vi "NMLWSD_Stability_8Units Rev B.vi"() -> ()   [LabVIEW 2017]
uses:
  C:/Program Files (x86)/Newport/Newport USB Driver/Bin/UsbDllWrap.dll
  Program Files (x86)/Newport/Newport USB Driver/Bin/UsbDllWrap.dll
  <vilib>/Analysis/baseanly.llb/Mean (DBL).vi
  <vilib>/Utility/file.llb/Read Delimited Spreadsheet (string).vi
  <vilib>/Utility/file.llb/Write Delimited Spreadsheet (string).vi
  <vilib>/Utility/file.llb/Read Delimited Spreadsheet (DBL).vi
  <vilib>/Analysis/NI_AALBase.lvlib
panel:
  out "Start Power":dbl=0.005 format="%.3p"
  out "Max Deviation":dbl format="%.2g %%"
  out "Min Power":dbl format="%.3p"
  out "Max Power":dbl format="%.3p"
  out "First Point":dbl format="%<%I:%M %p %m/%d/%y>T"
  out "Data Error":bool
  out "Timeout":bool
  out "Busy":bool
  out "Error":bool
  out "Msg":string="\n\r" caption="Status"
  in  "Stop":bool
  in  "Menu":T1(tab)
  in  "Comments":string[](array[string])=["", "", "", "", "", "", "", ""]
  in  "Start Test":bool
  out "Time":T2(graph) caption="Datar"
  in  "Display Parameter":u16(ring) items=["FW Version:", "On time (s):", "#shutter cycles:", "#power cycles:", "Temperature (°C):", "Temp set pt (°C):", "Tmax diode: (°C):", "Tmin laser: (°C):", "Tamb max: (°C):", "Hamb max: (RH):", "Current Tamb: (°C):", "Current Hamb: (RH):", "I_TEC (A):", "Laser Current (mA):", "IBias Initial(mA):", "MD Current (uA):", "APC_Set (V):", "Mod_Set (V):", "Vtune (V):", "LHM (V):", "Mode:", "WL:", "LHM Cal Gain:", "LHM Cal Offset:", "Power (W):", "Chamber Temperature (°C):", "V Logic (V):", "I Logic (A):", "V Laser (V):", "I Laser (A):", "V TEC (V):", "I TEC (A):", "V 24V (V):", "I 24V (A):", "Power_closed (W):"]
  out "Time 2":T2(graph) caption="Datar"
  in  "Read":bool
  out "Curs":dbl format="%<%I:%M %p %m/%d/%y>T"
  out "Pos":dbl format="%_3g"
  out "Results":bool
  in  "Display UUT #":i32(ring) items=["194910NPI-8NML", "194918NPI-8NML", "194805NPI-7NML", "194806NPI-7NML", "194911NPI-8NML", "194504NPI-8NML", "175003NPI-7NML", "194804NPI-7NML"]
  in  "New File":bool
  in  "Serial Numbers":string[](array[string])=["", "", "", "", "", "", "", ""]
  in  "DUT Count":i32(ring)=1 items=["1"=1, "2"=2, "3"=3, "4"=4, "5"=5, "6"=6, "7"=7, "8"=8]
  in  "Verify WavL":bool
  out "Re-conf Lambda":bool caption="Restart Test"
  out "Ready":bool caption="Restart Test"
  out "cDAQ2":string
  in  "Parameter File":path=path "C:/Test/WSNM Stability/Firmware_System/FW-Sys.csv"
  in  "Select Unit":i32(ring) items=["Unit 1", "Unit 2", "Unit 3", "Unit 4"]
  in  "Save Data":bool
  in  "850nm Folder":path=path "C:/Test/WSNM Stability/Data/850nm"
  in  "780nm Folder":path=path "C:/Test/WSNM Stability/Data/780nm"
  in  "635nm Folder":path=path "C:/Test/WSNM Stability/Data/635nm"
  out "Tpass Shtr Close":bool
  out "Shtr Close":bool
  out "Shtr Open":bool
  in  "Prep, min":dbl=30.0 min=0.0 format="%.2g"
  out "Com Open":bool[](array[boolean])=[FALSE, FALSE, FALSE, FALSE, FALSE, FALSE, FALSE, FALSE, FALSE, FALSE, TRUE, TRUE, TRUE, TRUE, TRUE, TRUE, TRUE, TRUE, TRUE, TRUE, TRUE, TRUE, TRUE, TRUE, TRUE, TRUE, TRUE, TRUE, TRUE, TRUE]
  out "Points":i32[](array[numeric])
  out "Devices":string[](array[string])
  out "COMs":refnum<visa-resource-name>[](array[refnum])
  out "Serial":string[](array[string])=["1"]
  out "System":string[][](table)
  in  "Open Ports":bool
  in  "Close Ports":bool
  in  "Reset PMs":bool
  out "cDAQ1":string
  in  "Open  Shutters":bool
  in  "Measure":bool
  in  "Power":bool
  in  "Clear Data":bool
  in  "Project Folder":path=path "C:/Test/WSNM Stability/Data"
  in  "Log File":path=path "C:/Test/WSNM Stability/Log.txt"
  in  "Settings File":path=path "C:/Test/WSNM Stability/Settings.txt"
  out "TimeS":string caption="Time"
  out "DateS":string caption="Date"
  in  "Stability Time, min":dbl=120.0 min=0.0 format="%.2f"
  in  "Warm-up, min":dbl=25.0 min=0.0 format="%.2g"
  in  "Interval, Seconds":dbl=10.0 min=0.0 format="%.2f"
  in  "Reset PSs":bool
  in  "Close  Shutters":bool
  in  "Shtr Ctrl Open, min":dbl=0.1 min=0.0 max=60.0 format="%.3f"
  in  "Shtr Ctrl Close, Seconds":dbl=6.0 max=60.0 format="%.3f"
  out "Tpass Shtr Open":bool
  in  "COM":refnum<visa-resource-name>="COM1"
  in  "PM USB Address":i32=1
  out "Lambda, nm":i32[](array[numeric])
  out "NML_WL":u16
  out "FW":u16
  in  "WL: NML Only":i32(ring)=1 items=["Red Only", "IR"]
  in  "FW inTest":u16(ring)=1 items=["WSD Board", "NML Board"]
  out "Enable":bool[](array[boolean])
  out "Module Error":bool[](array[boolean])
  out "PM_Range":i32 min=0 max=7 step=1
  out "System Data":dbl[](array[numeric]) format="%#_5p"
  out "MCU Data":dbl[](array[numeric]) format="%#_5p"
  out "Sys Prm":string[](array[string])=["Power (W):", "Chamber Temperature (°C):", "V Logic (V):", "I Logic (A):", "V Laser (V):", "I Laser (A):", "V TEC (V):", "I TEC (A):", "V 24V (V):", "I 24V (A):", "Power_closed (W):"]
  out "All Results":dbl[][][](array[numeric]) format="%8_4g"
  out "Order":string[](array[string])
  out "FW-SYS Info":string[][](table)
  out "FW ID":string[](array[string])
  out "FW Prm":string[](array[string])
  out "Pause":bool
  in  "Supply-PM Count":i32=4 min=1 max=4 step=1
  out "InitCriteria":bool
  out "PS RST":bool=TRUE
  out "Start Time":timestamp
  out "SysFileDelete":i32=30
  out "New Test":bool
  out "Soak Complete":bool=TRUE
  out "read buffer":string
  out "System Messages":string
  out "work buffer":string
  out "error":errorcluster
  out "DUT Count Old":i32=30
  out "Data Time":timestamp
  out "Old Cursor":dbl format="%<%I:%M %p %m/%d>T"
  out "Parameter Displayed":u16
  in  "Ret Prm IR":string[](array[string])=["FW Version:", "On time (s):", "#shutter cycles:", "#power cycles:", "Temperature (°C):", "Temp set pt (°C):", "Tmax diode: (°C):", "Tmin laser: (°C):", "Tamb max: (°C):", "Hamb max: (RH):", "Current Tamb: (°C):", "Current Hamb: (RH):", "I_TEC (A):", "Laser Current (mA):", "IBias Initial(mA):", "MD Current (uA):", "APC_Set (V):", "Mod_Set (V):", "Vtune (V):", "LHM (V):"]
  in  "Ret Prm Red":string[](array[string])=["Temperature (°C):", "Temp set pt (°C):", "Highest temp seen: (°C):", "Lowest temp seen: (°C):", "TEC current (A):", "Laser Current (mA):", "MD Current (uA):", "Power_Set (V):", "Modulation_Set (V):"]
  out "Powertime":dbl[](array[numeric]) format="%#_5p"
  out "Bytes Rcvd":i32=1000
  out "DUT Selected":i32
  out "Display UUT # Old":i32=30
  out "Meas N":i32
  out "Update Graph":bool
  out "Save":bool
  out "Collect":bool
  out "Shtr Ref Time":timestamp
  out "Shtr Ref0":timestamp
  out "reference Out":refnum<k24>
  out "ShtrCtrl Open Old":dbl=3.0 min=0.0 max=60.0 format="%.1f"
  out "ShtrCtrl Close Old":dbl=3.0 max=60.0 format="%.1f"
  out "MCUTrue":bool[][](array[boolean])
  out "SysTrue":bool[][](array[boolean])
  out "MCUCheck":string[][](array[string])
  out "SysCheck":string[][](array[string])
  out "MCUTrue2":bool[][](array[boolean])
  out "MCUReview2":bool[][](array[boolean])
  out "SysTrue2":bool[][](array[boolean])
  out "SysReview2":bool[][](array[boolean])
  out "FW Criteria":string[][](array[string])
  out "Sys Criteria":string[][](array[string])
  out "Ret Prm":string[](array[string])=["FW Version:", "On time (s):", "#shutter cycles:", "#power cycles:", "Temperature (°C):", "Temp set pt (°C):", "Tmax diode: (°C):", "Tmin laser: (°C):", "Tamb max: (°C):", "Hamb max: (RH):", "Current Tamb: (°C):", "Current Hamb: (RH):", "I_TEC (A):", "Laser Current (mA):", "IBias Initial(mA):", "MD Current (uA):", "APC_Set (V):", "Mod_Set (V):", "Vtune (V):", "LHM (V):"]
  out "MCUReview":bool[][](array[boolean])=[[TRUE], [TRUE], [TRUE], [TRUE], [TRUE], [TRUE], [TRUE], [FALSE], [TRUE], [FALSE], [FALSE], [FALSE], [FALSE], [TRUE], [TRUE], [TRUE], [TRUE], [TRUE], [TRUE], [FALSE], [FALSE], [FALSE], [TRUE], [TRUE], [TRUE], [FALSE], [FALSE], [TRUE], [TRUE], [TRUE], [TRUE], [TRUE], [TRUE], [TRUE], [FALSE], [TRUE], [FALSE], [FALSE]]
  out "SysReview":bool[][](array[boolean])
  # "NML/WSD Stability Test"
  # "Newport ISB"
  # "Configure"
  # "Test"
  # "Data"
  # "Folders"
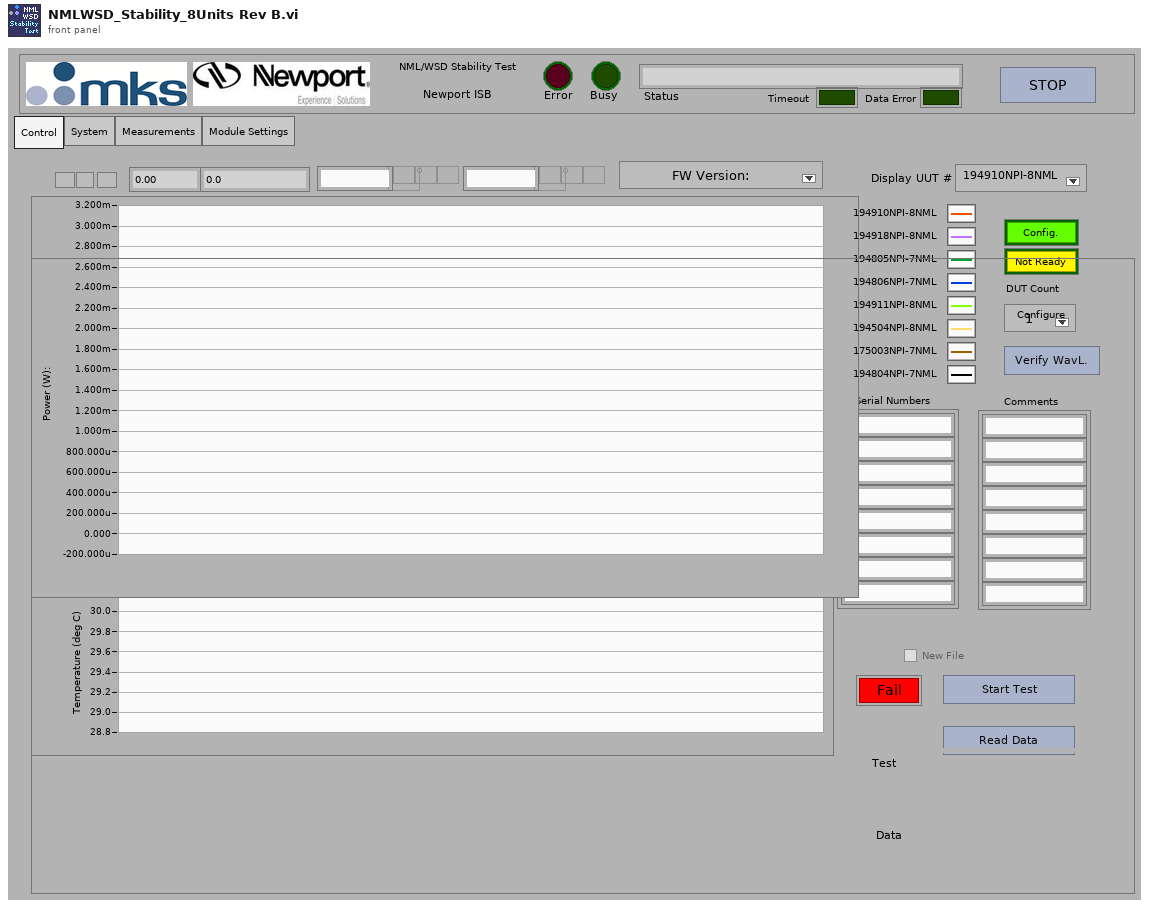
[diagram p1: front panel]
types:
  T1 = enum32{"Control", "System", "Measurements", "Module Settings"}
  T2 = cluster{"TimeStamps":timestamp[], " D Min":dbl[]}[]
  T3 = enum8{"Enabled", "Disabled", "Disabled and Grayed Out"}
  T4 = typedef "LVRangeTypeDef.ctl" = cluster{"Minimum":dbl, "Maximum":dbl, "Increment":dbl, "Minor Increment":dbl, "Start":dbl}
  T5 = typedef "LVRectTypeDef.ctl" = cluster{"Left":i16, "Top":i16, "Right":i16, "Bottom":i16}
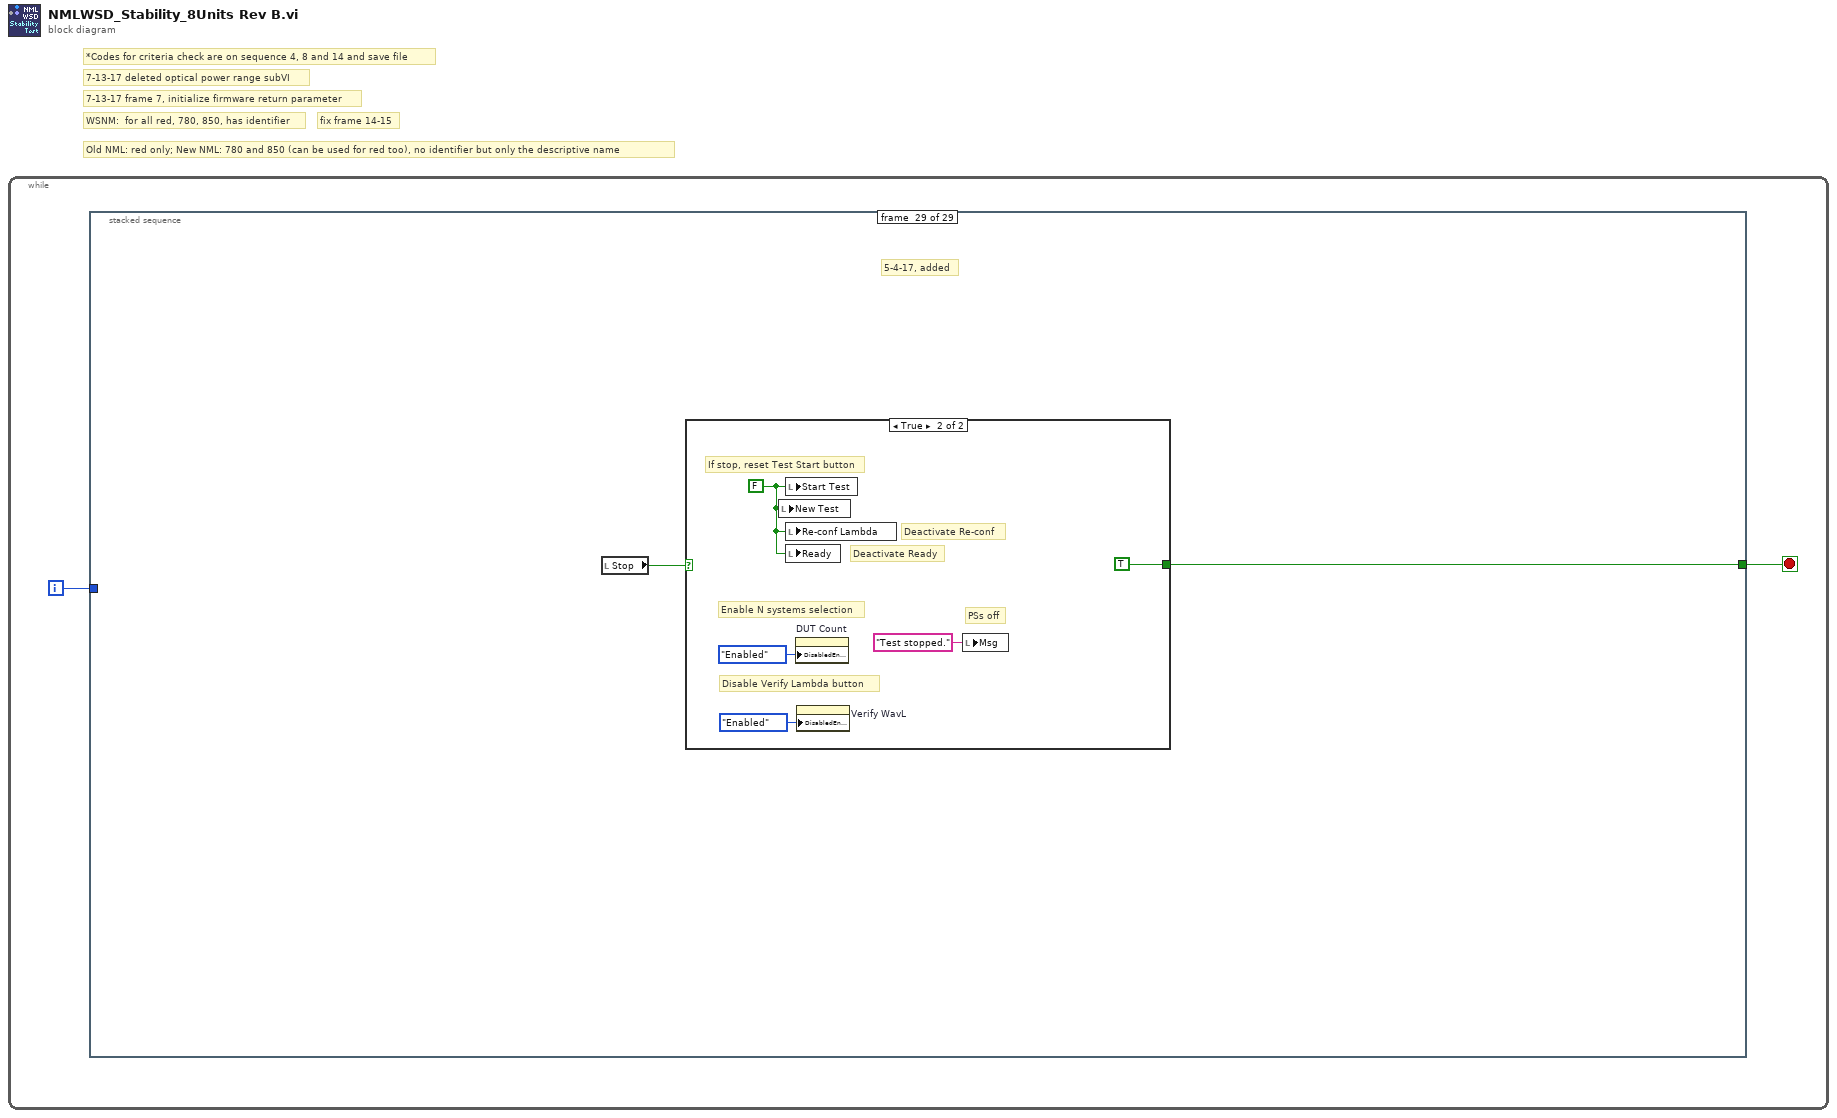
[diagram p0: block diagram]
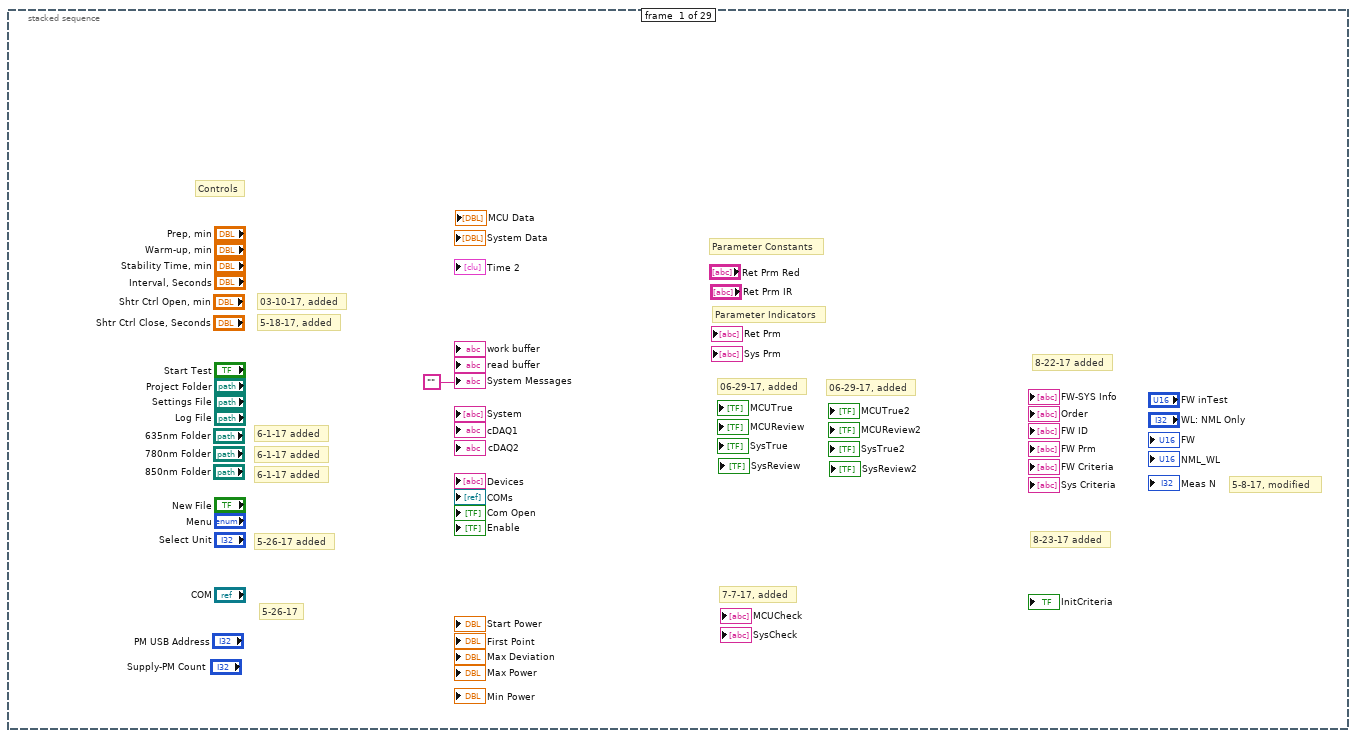
[diagram p2: hidden frame]
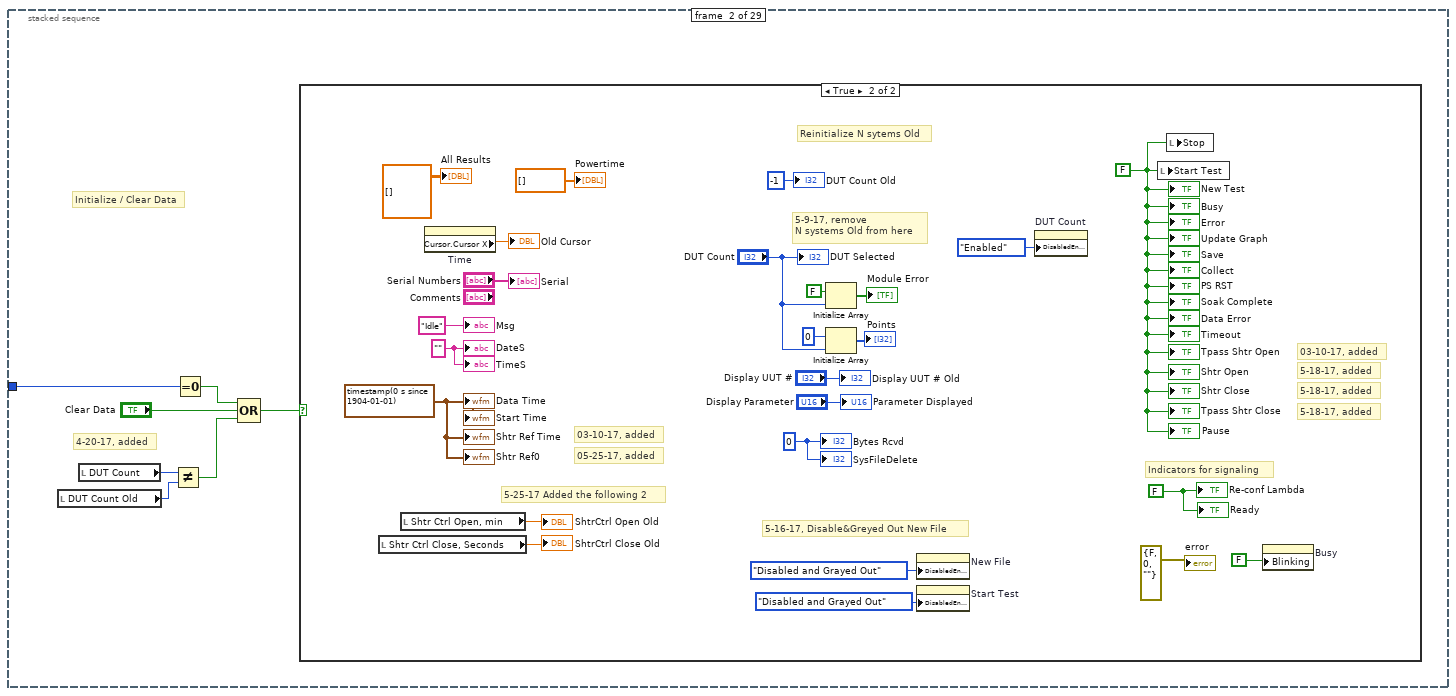
[diagram p3: hidden frame]
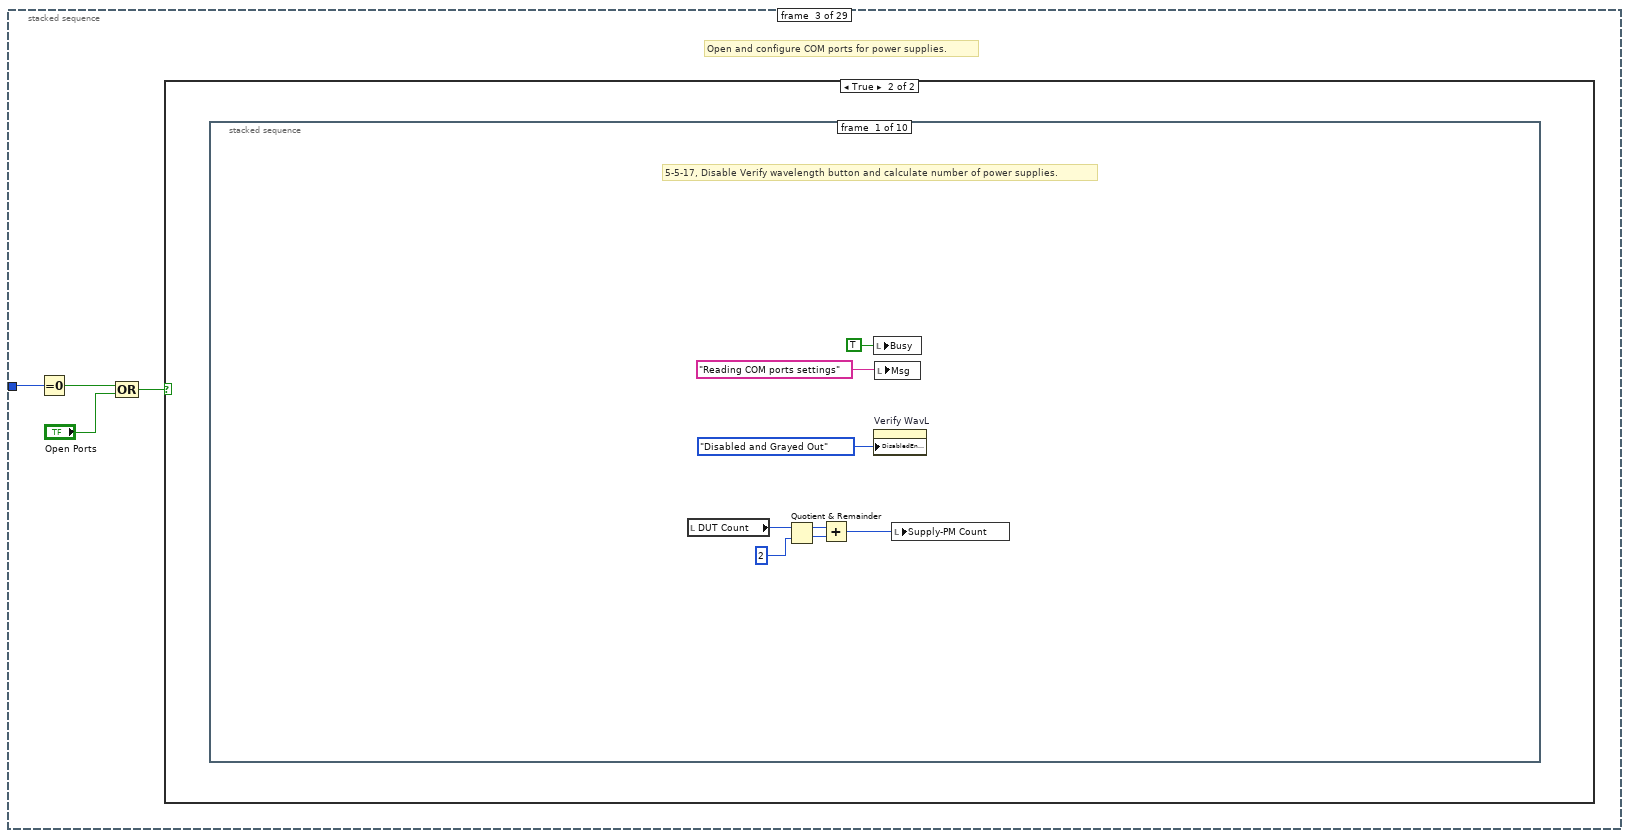
[diagram p5: hidden frame]
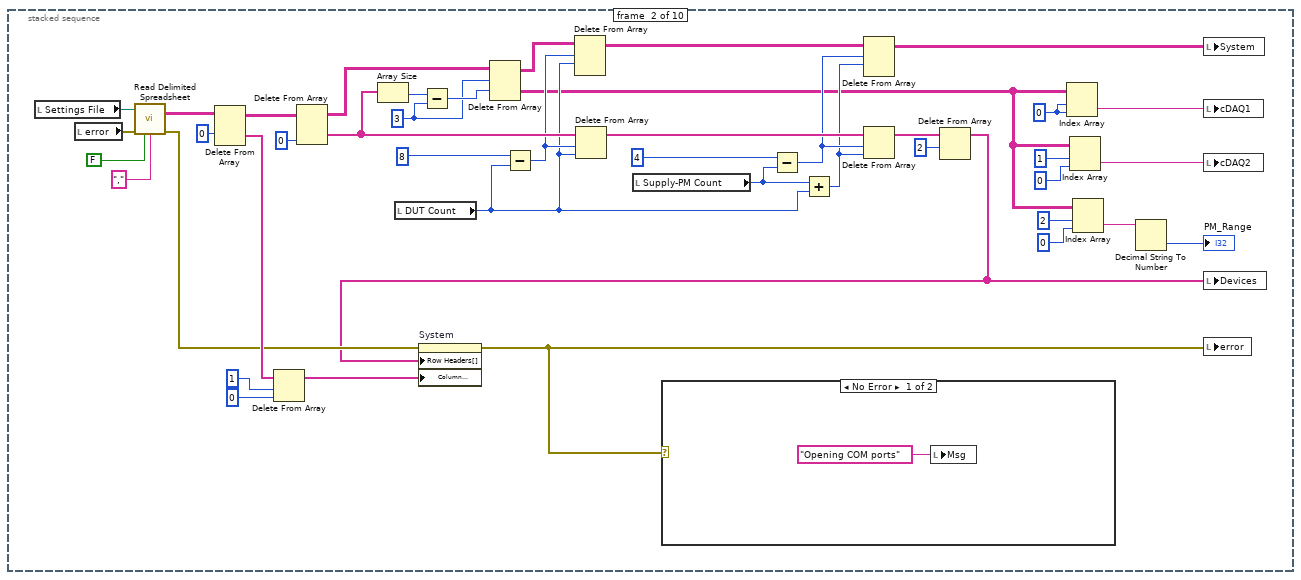
[diagram p7: hidden frame]
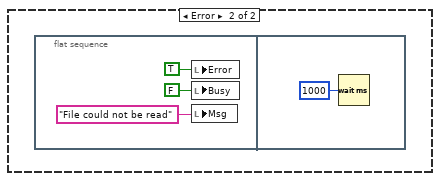
[diagram p8: hidden frame]
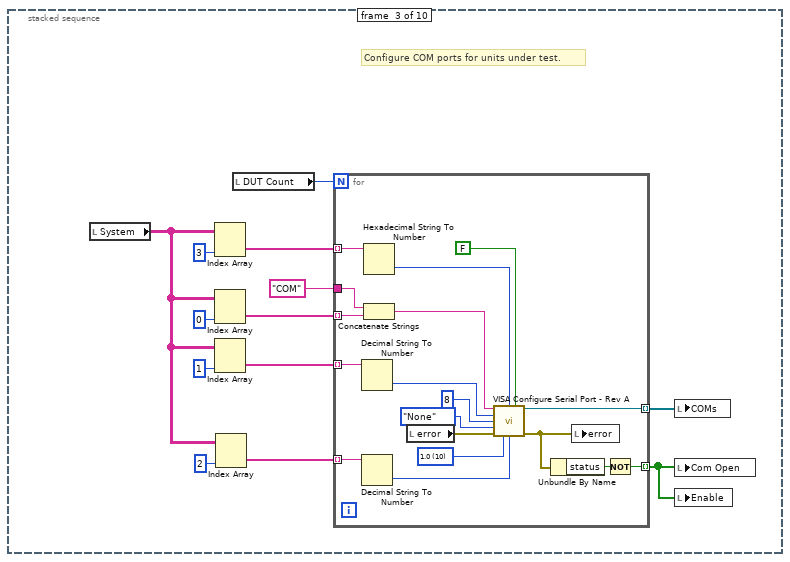
[diagram p9: hidden frame]
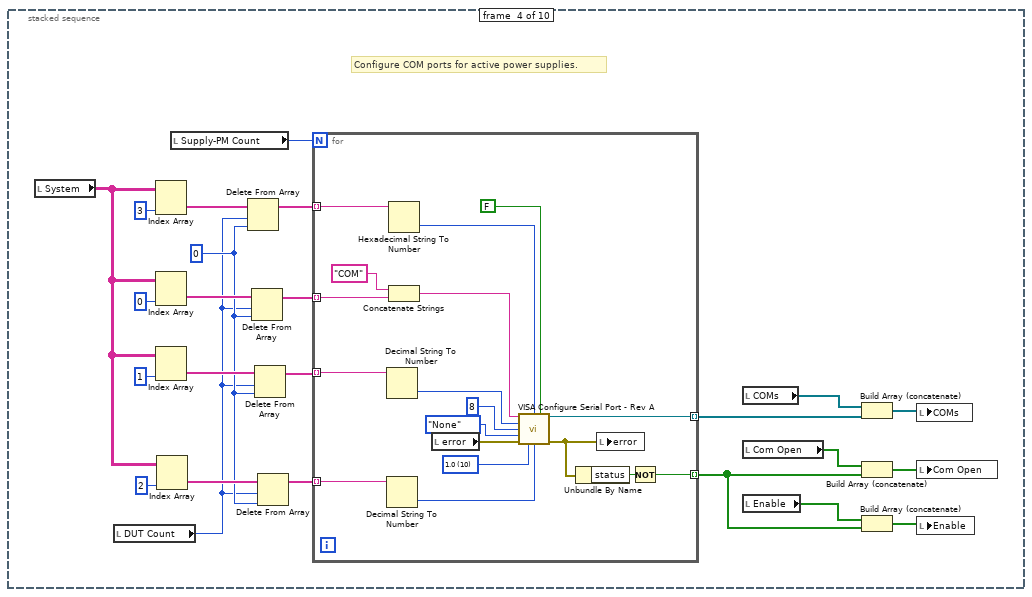
[diagram p10: hidden frame]
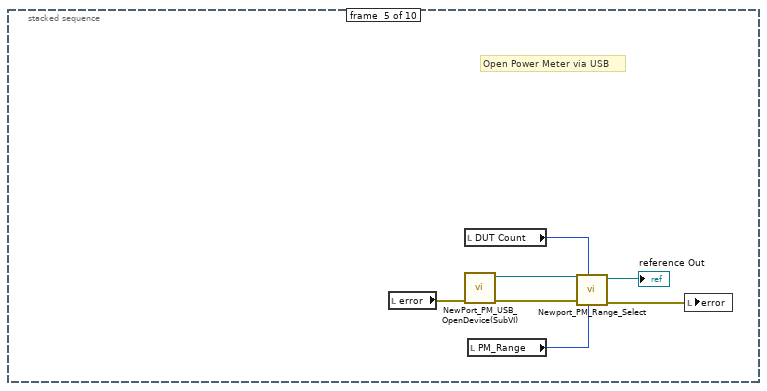
[diagram p11: hidden frame]
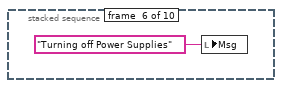
[diagram p12: hidden frame]
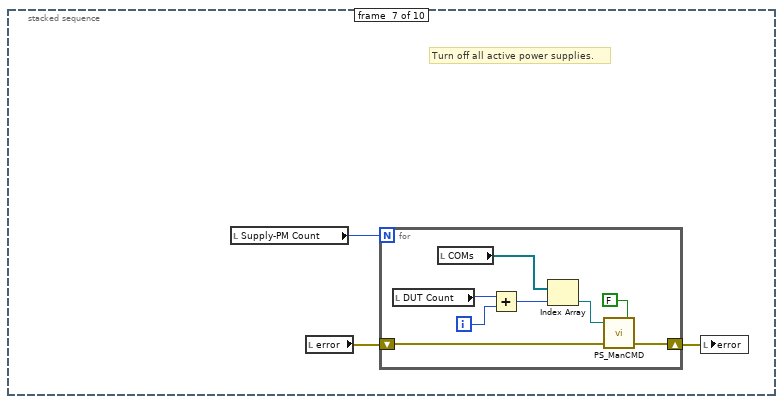
[diagram p13: hidden frame]
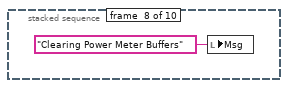
[diagram p14: hidden frame]
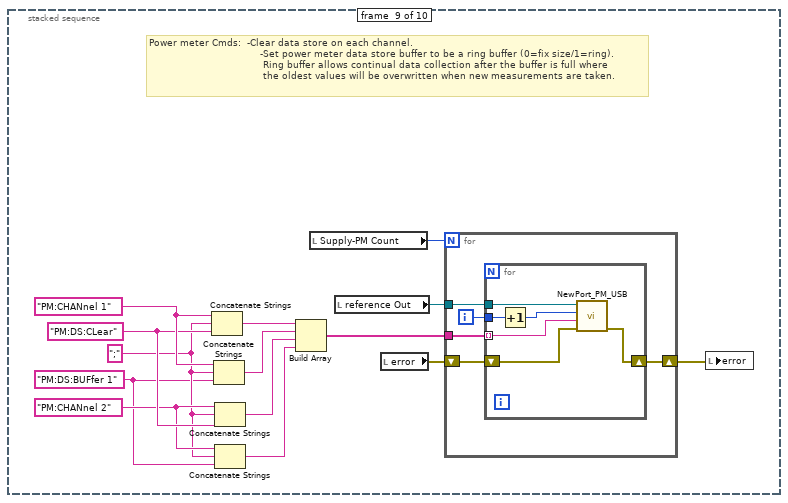
[diagram p15: hidden frame]
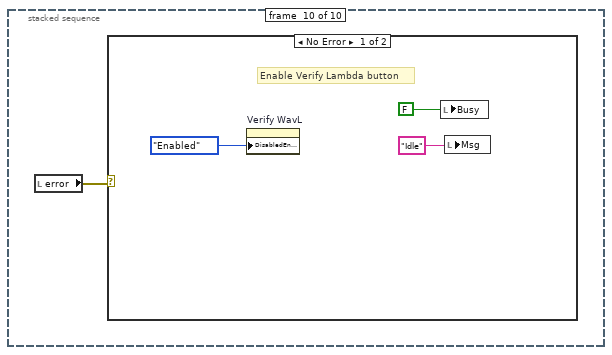
[diagram p16: hidden frame]
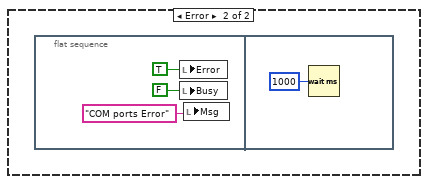
[diagram p17: hidden frame]
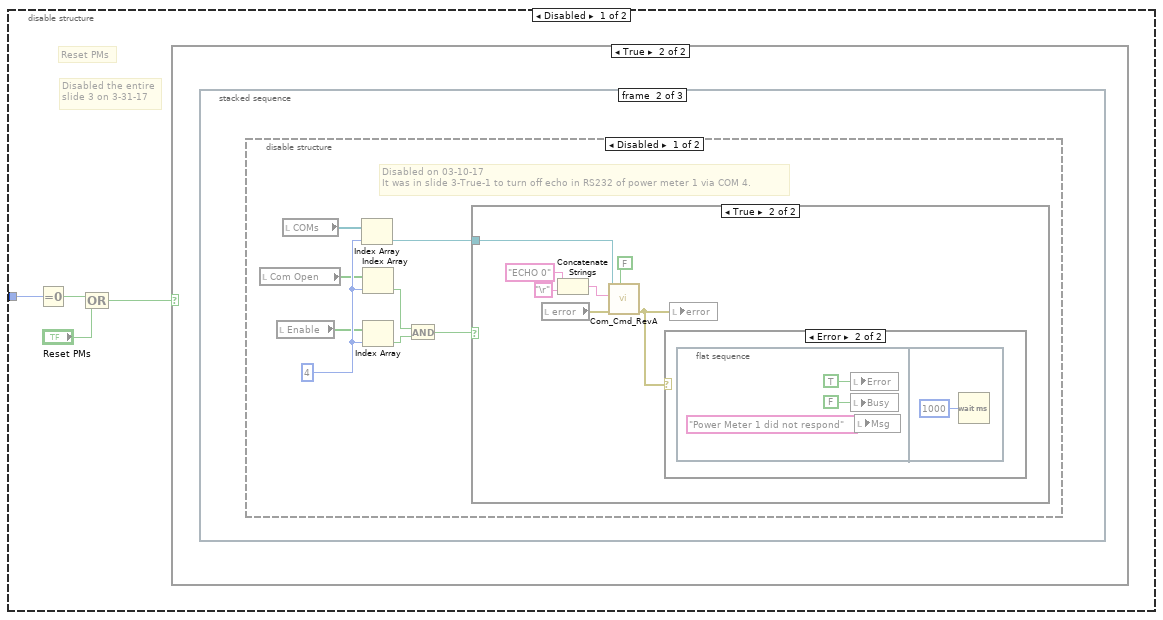
[diagram p19: hidden frame]
diagram:
  # "Old NML: red only; New NML: 780 and 850 (can be used for red too), no identifier but only the descriptive name"
  # "WSNM:  for all red, 780, 850, has identifier"
  # "*Codes for criteria check are on sequence 4, 8 and 14 and save file"
  # "fix frame 14-15"
  # "7-13-17 frame 7, initialize firmware return parameter"
  # "7-13-17 deleted optical power range subVI"
  n1 = while {
    i -> [w2]
    stop <- w1 stop-if-true
    n2 = stacked-sequence {
      tunnel: w2 -> [_ w10 w39 w222 w281 _ w331 _ _ w708 _ _ _ _ _ _ _ _ _ _ _ _ w1938 _ _ _ _ _ _]
      tunnel: [_ _ _ _ _ _ _ _ _ _ _ _ _ _ _ _ _ _ _ _ _ _ _ _ _ _ _ _ w2134] -> w1
      frame #0 {
        # "5-8-17, modified"
        # "8-23-17 added"
        # "8-22-17 added"
        # "06-29-17, added"
        # "7-7-17, added"
        # "06-29-17, added"
        # "6-1-17 added"
        # "6-1-17 added"
        # "6-1-17 added"
        # "5-26-17 added"
        # "5-26-17"
        # "Parameter Indicators"
        # "Parameter Constants"
        # "5-18-17, added"
        # "03-10-17, added"
        # "Controls"
        "System Messages" <- ""
      }
      frame #1 {
        # "4-20-17, added"
        # "Initialize / Clear Data"
        n3 = local read "DUT Count Old"() -> (w5:i32)
        n4 = local read "DUT Count"() -> (w6:i32)
        n5 = Not Equal?(x=w6, y=w5) -> (x != y?=w4:bool)
        n6 = Equal To 0?(x=w10) -> (x = 0?=w9:bool)
        n7 = Compound Arithmetic op=OR(w9, "Clear Data", w4) -> (w7:bool)
        n8 = case shown="True" w7 {
          frame False {
          }
          frame True {
            w12 = FALSE ("Restart Test")
            w22 = "" ("Result")
            w17 = 0 ("Bytes Rcvd")
            w11 = FALSE ("Auto")
            w27 = timestamp(0 s since 1904-01-01) ("Data Time")
            # "Indicators for signaling"
            # "5-25-17 Added the following 2"
            # "5-18-17, added"
            # "5-18-17, added"
            # "5-18-17, added"
            # "5-16-17, Disable&Greyed Out New File"
            # "Reinitialize N sytems Old"
            # "5-9-17, remove \nN systems Old from here"
            # "03-10-17, added"
            # "05-25-17, added"
            # "03-10-17, added"
            n9 = local read "Shtr Ctrl Close, Seconds"() -> (→"ShtrCtrl Close Old":dbl)
            n10 = local read "Shtr Ctrl Open, min"() -> (→"ShtrCtrl Open Old":dbl)
            n11 = property on="Time" class="XYGraph (strict)"() -> ("Cursor.Cursor X"=→"Old Cursor":dbl)  [unwired: 2 in, 2 out]
            n12 = Initialize Array(FALSE ("new element/subarray"), "DUT Count") -> (→"Module Error":bool[])
            n13 = Initialize Array(0 ("dimension size"), "DUT Count") -> (→"Points":i32[])
            n14 = property on="New File" class="Bool (strict)"("DisabledEnum"=T3."Disabled and Grayed Out" ("Disabled")) -> ()  [unwired: 2 in, 2 out]
            n15 = property on="Start Test" class="Bool (strict)"("DisabledEnum"=T3."Disabled and Grayed Out" ("Disabled")) -> ()  [unwired: 2 in, 2 out]
            n16 = property on="DUT Count" class="Ring (strict)"("DisabledEnum"=T3."Enabled" ("Disabled")) -> ()  [unwired: 2 in, 2 out]
            n17 = local write "Start Test"(w11) -> ()
            n18 = local write "Stop"(w11) -> ()
            n19 = property on="Busy" class="Bool (strict)"("Blinking"=FALSE) -> ()  [unwired: 2 in, 2 out]
            "Busy" <- w11
            "Error" <- w11
            "Parameter Displayed" <- "Display Parameter"
            "Update Graph" <- w11
            "Save" <- w11
            "Collect" <- w11
            "Data Time" <- w27
            "DUT Selected" <- "DUT Count"
            "error" <- errorcluster {"status"=FALSE, "code"=0, "source"=""} ("error")
            "Display UUT # Old" <- "Display UUT #"
            "Timeout" <- w11
            "Data Error" <- w11
            "New Test" <- w11
            "Start Time" <- w27
            "Bytes Rcvd" <- w17
            "PS RST" <- w11
            "Soak Complete" <- w11
            "SysFileDelete" <- w17
            "Msg" <- "Idle" ("Msg")
            "DateS" <- w22
            "TimeS" <- w22
            "Shtr Ref Time" <- w27
            "Tpass Shtr Open" <- w11
            "Shtr Ref0" <- w27
            "Serial" <- "Serial Numbers"
            "Powertime" <- dbl[] [] ("Powertime")
            "All Results" <- dbl[][][] [] ("All Results")
            "DUT Count Old" <- -1 ("N systems Old")
            "Shtr Open" <- w11
            "Shtr Close" <- w11
            "Tpass Shtr Close" <- w11
            "Re-conf Lambda" <- w12
            "Ready" <- w12
            "Pause" <- w11
          }
        }
      }
      frame #2 {
        # "Open and configure COM ports for power supplies."
        n20 = Equal To 0?(x=w39) -> (x = 0?=w38:bool)
        n21 = Compound Arithmetic op=OR(w38, "Open Ports") -> (w37:bool)
        n22 = case shown="True" w37 {
          frame False {
          }
          frame True {
            n23 = stacked-sequence {
              frame #0 {
                # "5-5-17, Disable Verify wavelength button and calculate number of power supplies."
                n24 = local read "DUT Count"() -> (w42:i32)
                n25 = Quotient & Remainder(x=w42, y=2) -> (x-y*floor(x/y)=w44:i32, floor(x/y)=w43:i32)
                n26 = Add(x=w44, y=w43) -> (x+y=w41:i32)
                n27 = local write "Busy"(TRUE ("Active")) -> ()
                n28 = property on="Verify WavL" class="Bool"("DisabledEnum"=T3."Disabled and Grayed Out" ("Disabled")) -> ()  [unwired: 2 in, 2 out]
                n29 = local write "Msg"("Reading COM ports settings" ("Msg")) -> ()
                n30 = local write "Supply-PM Count"(w41) -> ()
              }
              frame #1 {
                w53 = 3 ("y")
                w73 = 0 ("index (row)")
                n31 = local read "Settings File"() -> (w90:path)
                n32 = local read "error"() -> (w85:errorcluster)
                n33 = call-poly <vilib>:"Read Delimited Spreadsheet.vi"("file path (dialog if empty)"=w90, "error in (no error)"=w85, "transpose? (F)"=FALSE ("append to file? (new file:F)"), "delimiter (\\t)"="," ("delimiter (\\t)")) -> ("all rows"=w87:string[][], "error out"=w78:errorcluster)  [unwired: 6 in, 4 out]
                n34 = Delete From Array(array=w87, index (row)=0) -> (deleted portion=w82:string[], array with subset deleted=w84:string[][])  [unwired: 2 in]
                n35 = Delete From Array(array=w82, length=1, index=0) -> (array with subset deleted=w79:string[])  [unwired: 1 out]
                n36 = Delete From Array(array=w84, index (col)=0 ("disabled index (col)")) -> (deleted portion=w75:string[], array with subset deleted=w76:string[][])  [unwired: 2 in]
                n37 = Array Size(array=w75) -> (size(s)=w55:i32)
                n38 = local read "DUT Count"() -> (w60:i32)
                n39 = Subtract(x=w55, y=w53) -> (x-y=w74:i32)
                n40 = Delete From Array(array=w76, length=w53, index (row)=w74) -> (deleted portion=w50:string[][], array with subset deleted=w62:string[][])  [unwired: 1 in]
                n41 = Subtract(x=8, y=w60) -> (x-y=w61:i32)
                n42 = Delete From Array(array=w62, length=w61, index (row)=w60) -> (array with subset deleted=w59:string[][])  [unwired: 1 in, 1 out]
                n43 = Delete From Array(array=w75, length=w61, index=w60) -> (array with subset deleted=w67:string[])  [unwired: 1 out]
                n44 = local read "Supply-PM Count"() -> (w65:i32)
                n45 = Subtract(x=4, y=w65) -> (x-y=w58:i32)
                n46 = Add(x=w65, y=w60) -> (x+y=w57:i32)
                n47 = Delete From Array(array=w59, length=w58, index (row)=w57) -> (array with subset deleted=w56:string[][])  [unwired: 1 in, 1 out]
                n48 = Delete From Array(array=w67, length=w58, index=w57) -> (array with subset deleted=w64:string[])  [unwired: 1 out]
                n49 = Delete From Array(array=w64, length=2) -> (array with subset deleted=w63:string[])  [unwired: 1 in, 1 out]
                n50 = property on="System" class="Tbl (strict)"(error in=w78, "Row Headers[]"=w63, "Column Headers[]"=w79) -> (error out=w77:errorcluster)  [unwired: 1 in, 1 out]
                n51 = case shown="No Error" w77 {
                  frame No Error {
                    n52 = local write "Msg"("Opening COM ports" ("Msg")) -> ()
                  }
                  frame Error {
                    n53 = flat-sequence {
                      frame #0 {
                        n54 = local write "Error"(TRUE ("Active")) -> ()
                        n55 = local write "Busy"(FALSE ("Active")) -> ()
                        n56 = local write "Msg"("File could not be read" ("Msg")) -> ()
                      }
                      frame #1 {
                        n57 = Wait (ms)(milliseconds to wait=u32 1000) -> ()  [unwired: 1 out]
                      }
                    }
                  }
                }
                n58 = Index Array(array=w50, index (row)=w73, index (col)=w73) -> (element=w72:string)
                n59 = Index Array(array=w50, index (row)=1, index (col)=0 ("disabled index (col)")) -> (element=w70:string)
                n60 = Index Array(array=w50, index (row)=2, index (col)=0 ("disabled index (col)")) -> (element=w49:string)
                n61 = Decimal String To Number(string=w49) -> (number=→"PM_Range":i32)  [unwired: 2 in, 1 out]
                n62 = local write "System"(w56) -> ()
                n63 = local write "cDAQ1"(w72) -> ()
                n64 = local write "cDAQ2"(w70) -> ()
                n65 = local write "Devices"(w63) -> ()
                n66 = local write "error"(w77) -> ()
              }
              frame #2 {
                # "Configure COM ports for units under test."
                n67 = local read "System"() -> (w101:string[][])
                n68 = Index Array(array=w101, index (col)=3 ("disabled index (col)")) -> (element=w105:string[])  [unwired: 1 in]
                n69 = Index Array(array=w101, index (col)=0 ("disabled index (col)")) -> (element=w106:string[])  [unwired: 1 in]
                n70 = Index Array(array=w101, index (col)=1 ("disabled index (col)")) -> (element=w103:string[])  [unwired: 1 in]
                n71 = Index Array(array=w101, index (col)=2 ("disabled index (col)")) -> (element=w100:string[])  [unwired: 1 in]
                n72 = local read "DUT Count"() -> (w97:i32)
                n73 = for {
                  N: w97 -> [_]
                  tunnel: w106 -> [w126] mode=indexing
                  tunnel: w105 -> [w125] mode=indexing
                  tunnel: w103 -> [w124] mode=indexing
                  tunnel: w100 -> [w123] mode=indexing
                  tunnel: [w111] -> w96 mode=indexing
                  tunnel: [w110] -> w99 mode=indexing
                  tunnel: "COM" ("string") -> [w109]
                  w122 = u16 10 items=["1.0"=10, "1.5"=15, "2.0"=20] ("stop bits 4")
                  n74 = Decimal String To Number(string=w124) -> (number=w115:i32)  [unwired: 2 in, 1 out]
                  n75 = Decimal String To Number(string=w123) -> (number=w114:i32)  [unwired: 2 in, 1 out]
                  n76 = Hexadecimal String To Number(string=w125) -> (number=w117:u32)  [unwired: 2 in, 1 out]
                  n77 = Concatenate Strings(w109, w126) -> (w116:string)
                  n78 = local read "error"() -> (w119:errorcluster)
                  n79 = call "VISA Configure Serial Port - Rev A.vi"("VISA resource name"=w116, "termination char\n(0xA = '\\n' = LF)"=w117, "Enable Termination\nChar (T)"=FALSE ("Enable Termination\nChar (T)"), "baud rate (9600)"=w115, "data bits (8)"=u16 8 ("data bits 4"), "parity (0:none)"=enum16{"None", "Odd", "Even", "Mark", "Space"}."None" ("parity 4"), "error in (no error)"=w119, "stop bits (10: 1 bit)"=w122, "flow control (0:none)"=w114) -> ("VISA resource name out"=w110:refnum<visa-resource-name>, "error out"=w112:errorcluster)  [unwired: 5 in]
                  n80 = Unbundle By Name(w112) -> ("status"=w113:bool)
                  n81 = local write "error"(w112) -> ()
                  n82 = Not(x=w113) -> (.not. x?=w111:bool)
                }
                n83 = local write "COMs"(w99) -> ()
                n84 = local write "Com Open"(w96) -> ()
                n85 = local write "Enable"(w96) -> ()
              }
              frame #3 {
                w136 = 0 ("index")
                # "Configure COM ports for active power supplies."
                n86 = local read "System"() -> (w146:string[][])
                n87 = local read "DUT Count"() -> (w130:i32)
                n88 = Index Array(array=w146, index (col)=3 ("disabled index (col)")) -> (element=w143:string[])  [unwired: 1 in]
                n89 = Index Array(array=w146, index (col)=0 ("disabled index (col)")) -> (element=w141:string[])  [unwired: 1 in]
                n90 = Index Array(array=w146, index (col)=1 ("disabled index (col)")) -> (element=w139:string[])  [unwired: 1 in]
                n91 = Index Array(array=w146, index (col)=2 ("disabled index (col)")) -> (element=w137:string[])  [unwired: 1 in]
                n92 = local read "Supply-PM Count"() -> (w145:i32)
                n93 = Delete From Array(array=w143, length=w130, index=w136) -> (array with subset deleted=w144:string[])  [unwired: 1 out]
                n94 = Delete From Array(array=w141, length=w130, index=w136) -> (array with subset deleted=w142:string[])  [unwired: 1 out]
                n95 = Delete From Array(array=w139, length=w130, index=w136) -> (array with subset deleted=w140:string[])  [unwired: 1 out]
                n96 = Delete From Array(array=w137, length=w130, index=w136) -> (array with subset deleted=w138:string[])  [unwired: 1 out]
                n97 = for {
                  N: w145 -> [_]
                  tunnel: w142 -> [w168] mode=indexing
                  tunnel: w144 -> [w167] mode=indexing
                  tunnel: w140 -> [w166] mode=indexing
                  tunnel: w138 -> [w165] mode=indexing
                  tunnel: [w153] -> w127 mode=indexing
                  tunnel: [w152] -> w134 mode=indexing
                  w164 = u16 10 items=["1.0"=10, "1.5"=15, "2.0"=20] ("stop bits 4")
                  n98 = Decimal String To Number(string=w166) -> (number=w157:i32)  [unwired: 2 in, 1 out]
                  n99 = Decimal String To Number(string=w165) -> (number=w156:i32)  [unwired: 2 in, 1 out]
                  n100 = Hexadecimal String To Number(string=w167) -> (number=w159:u32)  [unwired: 2 in, 1 out]
                  n101 = Concatenate Strings("COM" ("string"), w168) -> (w158:string)
                  n102 = local read "error"() -> (w161:errorcluster)
                  n103 = call "VISA Configure Serial Port - Rev A.vi"("VISA resource name"=w158, "termination char\n(0xA = '\\n' = LF)"=w159, "Enable Termination\nChar (T)"=FALSE ("Enable Termination\nChar (T)"), "baud rate (9600)"=w157, "data bits (8)"=u16 8 ("data bits 4"), "parity (0:none)"=enum16{"None", "Odd", "Even", "Mark", "Space"}."None" ("parity 4"), "error in (no error)"=w161, "stop bits (10: 1 bit)"=w164, "flow control (0:none)"=w156) -> ("VISA resource name out"=w152:refnum<visa-resource-name>, "error out"=w154:errorcluster)  [unwired: 5 in]
                  n104 = Unbundle By Name(w154) -> ("status"=w155:bool)
                  n105 = local write "error"(w154) -> ()
                  n106 = Not(x=w155) -> (.not. x?=w153:bool)
                }
                n107 = local read "COMs"() -> (w135:refnum<visa-resource-name>[])
                n108 = local read "Com Open"() -> (w132:bool[])
                n109 = local read "Enable"() -> (w129:bool[])
                n110 = Build Array (concatenate)(w135, w134) -> (w133:refnum<visa-resource-name>[])
                n111 = Build Array (concatenate)(w132, w127) -> (w131:bool[])
                n112 = Build Array (concatenate)(w129, w127) -> (w128:bool[])
                n113 = local write "COMs"(w133) -> ()
                n114 = local write "Com Open"(w131) -> ()
                n115 = local write "Enable"(w128) -> ()
              }
              frame #4 {
                # "Open Power Meter via USB"
                n116 = local read "error"() -> (w175:errorcluster)
                n117 = local read "DUT Count"() -> (w170:i32)
                n118 = call "NewPort_PM_USB_OpenDevice(SubVI).vi"("error in"=w175) -> ("error out"=w173:errorcluster, "reference Out"=w174:refnum<k24>)  [unwired: 9 in]
                n119 = local read "PM_Range"() -> (w169:i32)
                n120 = call "Newport_PM_Range_Select.vi"("RANGE SEL"=w169, "DUT Count"=w170, "Error In"=w173, "Reference In"=w174) -> ("Error Out"=w171:errorcluster, "Reference Out"=→"reference Out":refnum<k24>)  [unwired: 4 in, 2 out]
                n121 = local write "error"(w171) -> ()
              }
              frame #5 {
                n122 = local write "Msg"("Turning off Power Supplies" ("Msg")) -> ()
              }
              frame #6 {
                # "Turn off all active power supplies."
                n123 = local read "Supply-PM Count"() -> (w177:i32)
                n124 = local read "error"() -> (w178:errorcluster)
                n125 = for {
                  N: w177 -> [_]
                  shift-right: [w183] -> w179
                  shift-left: w178 -> [w184]
                  i -> [w182]
                  n126 = local read "DUT Count"() -> (w180:i32)
                  n127 = local read "COMs"() -> (w185:refnum<visa-resource-name>[])
                  n128 = Add(x=w180, y=w182) -> (x+y=w181:i32)
                  n129 = Index Array(array=w185, index=w181) -> (element=w187:refnum<visa-resource-name>)
                  n130 = call "PS_ManCMD.vi"("Power Sup: T-On/F-Off"=FALSE, "error in"=w184, "VISA resource name"=w187) -> ("error out"=w183:errorcluster)  [unwired: 2 in]
                }
                n131 = local write "error"(w179) -> ()
              }
              frame #7 {
                n132 = local write "Msg"("Clearing Power Meter Buffers" ("Msg")) -> ()
              }
              frame #8 {
                w199 = "PM:CHANnel 2" ("PM:CMD_QUERY In")
                w197 = "PM:DS:BUFfer 1" ("PM:CMD_QUERY In")
                w198 = ";" ("PM:CMD_QUERY In")
                w200 = "PM:DS:CLear" ("PM:CMD_QUERY In")
                w201 = "PM:CHANnel 1" ("PM:CMD_QUERY In")
                # "Power meter Cmds:  -Clear data store on each channel.\n                                     -Set power meter data store buffer to be a ring buffer (0=fix size/1=ring).  \n                                      Ring buffer allows continual data collection after the buffer is full where \n                                      the oldest values will be overwritten when new measurements are taken."
                n133 = Concatenate Strings(w201, w198, w200) -> (w196:string)
                n134 = Concatenate Strings(w201, w198, w197) -> (w195:string)
                n135 = Concatenate Strings(w199, w198, w200) -> (w194:string)
                n136 = Concatenate Strings(w199, w198, w197) -> (w193:string)
                n137 = Build Array(w196, w195, w194, w193) -> (w192:string[])
                n138 = local read "Supply-PM Count"() -> (w189:i32)
                n139 = local read "reference Out"() -> (w202:refnum<k24>)
                n140 = local read "error"() -> (w191:errorcluster)
                n141 = for {
                  N: w189 -> [_]
                  tunnel: w202 -> [w207]
                  tunnel: w192 -> [w203]
                  shift-right: [w205] -> w190
                  shift-left: w191 -> [w206]
                  i -> [w204]
                  n142 = for {
                    tunnel: w207 -> [w213]
                    shift-right: [w211] -> w205
                    shift-left: w206 -> [w212]
                    tunnel: w204 -> [w210]
                    tunnel: w203 -> [w208] mode=indexing
                    n143 = Increment(x=w210) -> (x+1=w209:i32)
                    n144 = call "NewPort_PM_USB.vi"("error in"=w212, "PM:CMD_QUERY In"=w208, "USB Address"=w209, "reference"=w213) -> ("error out"=w211:errorcluster)  [unwired: 5 in, 2 out]
                  }
                }
                n145 = local write "error"(w190) -> ()
              }
              frame #9 {
                n146 = local read "error"() -> (w214:errorcluster)
                n147 = case shown="No Error" w214 {
                  frame No Error {
                    # "Enable Verify Lambda button"
                    n148 = property on="Verify WavL" class="Bool"("DisabledEnum"=T3."Enabled" ("Disabled")) -> ()  [unwired: 2 in, 2 out]
                    n149 = local write "Busy"(FALSE ("Active")) -> ()
                    n150 = local write "Msg"("Idle" ("Msg")) -> ()
                  }
                  frame Error {
                    n151 = flat-sequence {
                      frame #0 {
                        n152 = local write "Error"(TRUE ("Active")) -> ()
                        n153 = local write "Busy"(FALSE ("Active")) -> ()
                        n154 = local write "Msg"("COM ports Error" ("Msg")) -> ()
                      }
                      frame #1 {
                        n155 = Wait (ms)(milliseconds to wait=u32 1000) -> ()  [unwired: 1 out]
                      }
                    }
                  }
                }
              }
            }
          }
        }
      }
      frame #3 {
        n156 = disable-structure shown="Enabled" {
          disable-tunnel: w222 -> [w226 _]
          frame Disabled {
            # "Disabled the entire\nslide 3 on 3-31-17"
            # "Reset PMs"
            n157 = Equal To 0?(x=w226) -> (x = 0?=w225:bool)
            n158 = Compound Arithmetic op=OR(w225, "Reset PMs") -> (w224:bool)
            n159 = case shown="True" w224 {
              frame False {
              }
              frame True {
                n160 = stacked-sequence {
                  frame #0 {
                    n161 = local write "Busy"(TRUE ("Active")) -> ()
                    n162 = local write "Msg"("Resetting Power Meters" ("Msg")) -> ()
                  }
                  frame #1 {
                    n163 = disable-structure shown="Disabled" {
                      frame Disabled {
                        w236 = 4 ("index")
                        # "Disabled on 03-10-17\nIt was in slide 3-True-1 to turn off echo in RS232 of power meter 1 via COM 4."
                        n164 = local read "Com Open"() -> (w229:bool[])
                        n165 = local read "Enable"() -> (w230:bool[])
                        n166 = local read "COMs"() -> (w231:refnum<visa-resource-name>[])
                        n167 = Index Array(array=w231, index=w236) -> (element=w235:refnum<visa-resource-name>)
                        n168 = Index Array(array=w229, index=w236) -> (element=w233:bool)
                        n169 = Index Array(array=w230, index=w236) -> (element=w232:bool)
                        n170 = And(x=w233, y=w232) -> (x .and. y?=w234:bool)
                        n171 = case shown="True" w234 {
                          tunnel: w235 -> [_ w241]
                          frame False {
                          }
                          frame True {
                            n172 = local read "error"() -> (w239:errorcluster)
                            n173 = Concatenate Strings("ECHO 0" ("write buffer"), "\r") -> (w240:string)
                            n174 = call "Com_Cmd_RevA.vi"("Query"=FALSE, "error in"=w239, "write buffer"=w240, "VISA"=w241) -> ("error out"=w237:errorcluster)  [unwired: 2 in, 5 out]
                            n175 = case shown="Error" w237 {
                              frame No Error {
                                n176 = local write "Busy"(FALSE ("Active")) -> ()
                                n177 = local write "Msg"("Idle" ("Msg")) -> ()
                              }
                              frame Error {
                                n178 = flat-sequence {
                                frame #0 {
                                n179 = local write "Error"(TRUE ("Active")) -> ()
                                n180 = local write "Busy"(FALSE ("Active")) -> ()
                                n181 = local write "Msg"("Power Meter 1 did not respond" ("Msg")) -> ()
                                }
                                frame #1 {
                                n182 = Wait (ms)(milliseconds to wait=u32 1000) -> ()  [unwired: 1 out]
                                }
                                }
                              }
                            }
                            n183 = local write "error"(w237) -> ()
                          }
                        }
                      }
                      frame Enabled {
                      }
                    }
                  }
                  frame #2 {
                    n184 = disable-structure shown="Disabled" {
                      frame Disabled {
                        w250 = 5 ("index")
                        # "Disabled on 03-10-17\nIt was in slide 3-True-2 to turn off echo in RS232 of power meter 2 via COM 5."
                        n185 = local read "Com Open"() -> (w257:bool[])
                        n186 = local read "Enable"() -> (w256:bool[])
                        n187 = local read "COMs"() -> (w255:refnum<visa-resource-name>[])
                        n188 = Index Array(array=w255, index=w250) -> (element=w251:refnum<visa-resource-name>)
                        n189 = Index Array(array=w257, index=w250) -> (element=w253:bool)
                        n190 = Index Array(array=w256, index=w250) -> (element=w254:bool)
                        n191 = And(x=w253, y=w254) -> (x .and. y?=w252:bool)
                        n192 = case shown="True" w252 {
                          tunnel: w251 -> [_ w262]
                          frame False {
                          }
                          frame True {
                            n193 = local read "error"() -> (w260:errorcluster)
                            n194 = Concatenate Strings("ECHO 0" ("write buffer"), "\r") -> (w261:string)
                            n195 = call "Com_Cmd_RevA.vi"("Query"=FALSE, "error in"=w260, "write buffer"=w261, "VISA"=w262) -> ("error out"=w258:errorcluster)  [unwired: 2 in, 5 out]
                            n196 = case shown="Error" w258 {
                              frame No Error {
                                n197 = local write "Busy"(FALSE ("Active")) -> ()
                                n198 = local write "Msg"("Idle" ("Msg")) -> ()
                              }
                              frame Error {
                                n199 = flat-sequence {
                                frame #0 {
                                n200 = local write "Error"(TRUE ("Active")) -> ()
                                n201 = local write "Busy"(FALSE ("Active")) -> ()
                                n202 = local write "Msg"("Power Meter 2 did not respond" ("Msg")) -> ()
                                }
                                frame #1 {
                                n203 = Wait (ms)(milliseconds to wait=u32 1000) -> ()  [unwired: 1 out]
                                }
                                }
                              }
                            }
                            n204 = local write "error"(w258) -> ()
                          }
                        }
                      }
                      frame Enabled {
                      }
                    }
                  }
                }
              }
            }
          }
          frame Enabled {
          }
        }
      }
      frame #4 {
        # "Open Shutters"
        n205 = local read "DUT Count"() -> (w275:i32)
        n206 = local read "DUT Count Old"() -> (w278:i32)
        n207 = Equal To 0?(x=w281) -> (x = 0?=w280:bool)
        n208 = Not Equal?(x=w278, y=w275) -> (x != y?=w277:bool)
        n209 = Compound Arithmetic op=OR("Open  Shutters", w280, w277) -> (w279:bool)
        n210 = Greater?(x=w275, y=4) -> (0:w273:bool)
        n211 = local read "error"() -> (w272:errorcluster)
        n212 = case shown="True" w279 {
          tunnel: w273 -> [_ w286]
          tunnel: w272 -> [w282 w285]
          tunnel: [w282 w283] -> w271
          frame False {
          }
          frame True {
            w292 = FALSE
            n213 = case shown="True" w286 {
              tunnel: w285 -> [w295 w297]
              tunnel: [w295 w296] -> w284
              frame False {
              }
              frame True {
                w300 = FALSE
                n214 = local read "cDAQ2"() -> (w302:string)
                n215 = Concatenate Strings(w302, "Mod1" ("string")) -> (w301:string)
                n216 = Build Array(w300, w300, w300, w300) -> (w299:bool[])
                n217 = call "DAQ Assistant10"("data"=w299, "error in"=w297, "device name"=w301) -> ("error out"=w296:errorcluster)  [unwired: 15 in, 1 out]
              }
            }
            n218 = local write "Msg"("Shutters open" ("Msg")) -> ()
            n219 = local write "Shtr Open"(TRUE ("Sttrs Open")) -> ()
            n220 = local read "cDAQ1"() -> (w294:string)
            n221 = local write "Busy"(FALSE ("Active")) -> ()
            n222 = Concatenate Strings(w294, "Mod1" ("string")) -> (w293:string)
            n223 = Build Array(w292, w292, w292, w292) -> (w290:bool[])
            n224 = call "DAQ Assistant5"("data"=w290, "error in"=w284, "device name"=w293) -> ("error out"=w283:errorcluster)  [unwired: 15 in, 1 out]
          }
        }
        n225 = local write "error"(w271) -> ()
      }
      frame #5 {
        # "Close Shutters"
        n226 = local read "DUT Count"() -> (w307:i32)
        n227 = local read "error"() -> (w304:errorcluster)
        n228 = Greater?(x=w307, y=4) -> (0:w305:bool)
        n229 = case shown="True" "Close  Shutters" {
          tunnel: w305 -> [_ w313]
          tunnel: w304 -> [w309 w312]
          tunnel: [w309 w310] -> w303
          frame False {
          }
          frame True {
            w319 = TRUE
            n230 = case shown="True" w313 {
              tunnel: w312 -> [w322 w324]
              tunnel: [w322 w323] -> w311
              frame False {
              }
              frame True {
                w326 = TRUE
                n231 = local read "cDAQ2"() -> (w329:string)
                n232 = Concatenate Strings(w329, "Mod1" ("string")) -> (w328:string)
                n233 = Build Array(w326, w326, w326, w326) -> (w325:bool[])
                n234 = call "DAQ Assistant11"("data"=w325, "error in"=w324, "device name"=w328) -> ("error out"=w323:errorcluster)  [unwired: 15 in, 1 out]
              }
            }
            n235 = local write "Msg"("Shutters closed" ("Msg")) -> ()
            n236 = local write "Shtr Close"(TRUE ("Sttrs Close")) -> ()
            n237 = local read "cDAQ1"() -> (w321:string)
            n238 = Concatenate Strings(w321, "Mod1" ("string")) -> (w320:string)
            n239 = Build Array(w319, w319, w319, w319) -> (w318:bool[])
            n240 = local write "Busy"(FALSE ("Active")) -> ()
            n241 = call "DAQ Assistant7"("data"=w318, "error in"=w311, "device name"=w320) -> ("error out"=w310:errorcluster)  [unwired: 15 in, 1 out]
          }
        }
        n242 = local write "error"(w303) -> ()
      }
      frame #6 {
        # "8-22-17\nExtract firmware parameter and criteria range  Info"
        n243 = local read "WL: NML Only"() -> (w335:i32)
        n244 = local read "NML_WL"() -> (w334:u16)
        n245 = local read "FW inTest"() -> (w338:u16)
        n246 = local read "FW"() -> (w337:u16)
        n247 = Not Equal?(x=w338, y=w337) -> (x != y?=w336:bool)
        n248 = Not Equal?(x=w335, y=w334) -> (x != y?=w333:bool)
        n249 = Equal To 0?(x=w331) -> (x = 0?=w332:bool)
        n250 = Compound Arithmetic op=OR(w332, w336, w333) -> (w330:bool)
        n251 = case shown="True" w330 {
          frame False {
          }
          frame True {
            n252 = stacked-sequence {
              frame #0 {
                w389 = 20 ("index (col)")
                # "8=No ID for NML IR"
                # "2=No ID for NML Red"
                # "14=WSD FW ID"
                # "NML_WL in Test\n0=NML board Red only\n1=NML board near IR"
                # "FW in Test\n0=WSD (dark) board\n1=NML (light) board"
                # "0=order from NML board for Red\n6=order from NML board for IR (can be used for red too)\n12=order from WSD board"
                # "For WSD board criteria"
                # "For NML board IR criteria"
                # "For NML board red criteria"
                # "1=parameters from NML board for Red\n7=parameters from NML board for IR (can be used for red too)\n13=parameters from WSD board"
                # "Delete 0th\nrow"
                n253 = call-poly <vilib>:"Read Delimited Spreadsheet.vi"("file path (dialog if empty)"="Parameter File", "transpose? (F)"=FALSE, "delimiter (\\t)"="," ("delimiter (\\t)")) -> ("all rows"=w378:string[][])  [unwired: 7 in, 5 out]
                n254 = local write "FW-SYS Info"(w378) -> ()
                n255 = Delete From Array(array=w378, length=1, index (row)=0) -> (array with subset deleted=w361:string[][])  [unwired: 1 in, 1 out]
                n256 = local write "Msg"("Reading firmware file..." ("Msg")) -> ()
                n257 = Index Array(array=w361, index (col) #1=1 ("disabled index (col)"), index (col) #2=7 ("disabled index (col)"), index (col) #3=13 ("disabled index (col)")) -> (element #1=w344:string[], element #2=w341:string[], element #3=w351:string[])  [unwired: 3 in]
                n258 = Index Array(array=w361, index (col) #1=0 ("index (col)"), index (col) #2=6 ("index (col)"), index (col) #3=12 ("index (col)")) -> (element #1=w343:string[], element #2=w342:string[], element #3=w354:string[])  [unwired: 3 in]
                n259 = Delete From Array(array=w361, length=2, index (col)=4 ("length")) -> (deleted portion=w382:string[][])  [unwired: 1 in, 1 out]
                n260 = Delete From Array(array=w361, length=2, index (col)=10 ("length")) -> (deleted portion=w383:string[][])  [unwired: 1 in, 1 out]
                n261 = Delete From Array(array=w361, length=2, index (col)=16 ("length")) -> (deleted portion=w348:string[][])  [unwired: 1 in, 1 out]
                n262 = Delete From Array(array=w361, length=2, index (col)=20 ("disabled index (col)")) -> (deleted portion=w360:string[][])  [unwired: 1 in, 1 out]
                n263 = Index Array(array=w361, index (col) #1=2 ("disabled index (col)"), index (col) #2=8 ("index (col)"), index (col) #3=14 ("disabled index (col)")) -> (element #1=w340:string[], element #2=w339:string[], element #3=w345:string[])  [unwired: 3 in]
                n264 = local write "Sys Criteria"(w360) -> ()
                n265 = Array Size(array=w354) -> (size(s)=w381:i32)
                n266 = Subtract(x=w381, y=w389) -> (x-y=w388:i32)
                n267 = local read "WL: NML Only"() -> (w357:i32)
                n268 = local read "FW inTest"() -> (w358:u16)
                n269 = Delete From Array(array=w382) -> (array with subset deleted=w350:string[][])  [unwired: 3 in, 1 out]
                n270 = Delete From Array(array=w383, length=w388, index (row)=w389) -> (array with subset deleted=w349:string[][])  [unwired: 1 in, 1 out]
                n271 = call "Build System Param Arrays.vi"("Input String Array"=w343) -> ("Output String Array"=w356:string[])  [unwired: 9 in, 1 out]
                n272 = call "Build System Param Arrays.vi"("Input String Array"=w342) -> ("Output String Array"=w355:string[])  [unwired: 9 in, 1 out]
                n273 = call "Build System Param Arrays.vi"("Input String Array"=w344) -> ("Output String Array"=w353:string[])  [unwired: 9 in, 1 out]
                n274 = call "Build System Param Arrays.vi"("Input String Array"=w341) -> ("Output String Array"=w352:string[])  [unwired: 9 in, 1 out]
                n275 = call "Build System Param Arrays.vi"("Input String Array"=w340) -> ("Output String Array"=w347:string[])  [unwired: 9 in, 1 out]
                n276 = call "Build System Param Arrays.vi"("Input String Array"=w339) -> ("Output String Array"=w346:string[])  [unwired: 9 in, 1 out]
                n277 = stacked-sequence {
                  tunnel: w358 -> [w396 w426]
                  tunnel: w357 -> [w395 w425]
                  tunnel: w356 -> [w394 w424]
                  tunnel: w355 -> [w393 w423]
                  tunnel: w354 -> [w392 w422]
                  tunnel: w353 -> [_ w421]
                  tunnel: w352 -> [_ w420]
                  tunnel: w351 -> [_ w419]
                  tunnel: w350 -> [_ w418]
                  tunnel: w349 -> [_ w417]
                  tunnel: w348 -> [_ w416]
                  tunnel: w347 -> [_ w415]
                  tunnel: w346 -> [_ w414]
                  tunnel: w345 -> [_ w413]
                  frame #0 {
                    n278 = case shown="1" w396 {
                      tunnel: w392 -> [w398 _]
                      tunnel: [w397 w400] -> w391
                      tunnel: w395 -> [_ w402]
                      tunnel: w394 -> [_ w401]
                      tunnel: w393 -> [_ w399]
                      frame 0, Default {
                        # "WSD FW"
                        n279 = Array Size(array=w398) -> (size(s)=w397:i32)
                      }
                      frame 1 {
                        # "NML FW"
                        n280 = case shown="0, Default" w402 {
                          tunnel: w401 -> [w404 _]
                          tunnel: [w403 w405] -> w400
                          tunnel: w399 -> [_ w408]
                          frame 0, Default {
                            # "NML Red"
                            n281 = Array Size(array=w404) -> (size(s)=w403:i32)
                          }
                          frame 1 {
                            # "NML IR"
                            n282 = Array Size(array=w408) -> (size(s)=w407:i32)
                            n283 = Add(x=w407, y=4) -> (x+y=w405:i32)
                          }
                        }
                      }
                    }
                    n284 = Increment(x=w391) -> (x+1=w390:i32)
                    n285 = property on="Order" class="Arr (strict)"("Number of Rows"=w391) -> ()  [unwired: 2 in, 2 out]
                    n286 = property on="FW Prm" class="Arr (strict)"("Number of Rows"=w391) -> ()  [unwired: 2 in, 2 out]
                    n287 = property on="FW ID" class="Arr (strict)"("Number of Rows"=w391) -> ()  [unwired: 2 in, 2 out]
                    n288 = property on="MCU Data" class="Arr (strict)"("Number of Rows"=w390) -> ()  [unwired: 2 in, 2 out]
                  }
                  frame #1 {
                    # "For Range check"
                    # "For display"
                    # "For tranfer to RetPrm"
                    n289 = case shown="1" w426 {
                      tunnel: w425 -> [w439 _]
                      tunnel: w424 -> [w438 _]
                      tunnel: w423 -> [w437 _]
                      tunnel: [w436 w453] -> w412
                      tunnel: w422 -> [_ w453]
                      tunnel: w421 -> [w435 _]
                      tunnel: [w434 w452] -> w411
                      tunnel: w420 -> [w433 _]
                      tunnel: w419 -> [_ w452]
                      tunnel: w418 -> [w432 _]
                      tunnel: [w431 w451] -> w410
                      tunnel: w417 -> [w430 _]
                      tunnel: w416 -> [_ w451]
                      tunnel: w415 -> [w429 _]
                      tunnel: [w428 w450] -> w409
                      tunnel: w414 -> [w427 _]
                      tunnel: w413 -> [_ w450]
                      frame 1 {
                        # "NML FW"
                        n290 = case shown="0, Default" w439 {
                          tunnel: w438 -> [w443 _]
                          tunnel: w437 -> [_ w449]
                          tunnel: [w443 w449] -> w436
                          tunnel: w435 -> [w441 _]
                          tunnel: [w441 w446] -> w434
                          tunnel: w433 -> [_ w447]
                          tunnel: w432 -> [w442 _]
                          tunnel: [w442 w444] -> w431
                          tunnel: w430 -> [_ w444]
                          tunnel: w429 -> [w440 _]
                          tunnel: [w440 w445] -> w428
                          tunnel: w427 -> [_ w445]
                          frame 0, Default {
                            # "NML Red"
                          }
                          frame 1 {
                            # "NML IR"
                            # "Since NML IR FW doesn't have these 2 parameters(Mode and WL), they are manually added to the firmware parameter list"
                            n291 = Build Array (concatenate)(w447, string[] ["Mode:", "WL:", "LHM Cal Gain:", "LHM Cal Offset:"] ("element")) -> (w446:string[])
                          }
                        }
                      }
                      frame 0, Default {
                        # "WSD FW"
                      }
                    }
                    n292 = local write "FW Criteria"(w410) -> ()
                    n293 = local write "FW Prm"(w411) -> ()
                    n294 = local write "Order"(w412) -> ()
                    n295 = local write "FW ID"(w409) -> ()
                  }
                }
              }
              frame #1 {
                # "Increase parameter size by 1 to store time which is one extra item"
                n296 = local read "FW Prm"() -> (w459:string[])
                n297 = local read "Sys Prm"() -> (w461:string[])
                n298 = Build Array (concatenate)(w459, w461) -> (w454:string[])
                n299 = Array Size(array=w454) -> (size(s)=w460:i32)
                n300 = property on="Display Parameter" class="Ring (strict)"("Strings []"=w454) -> ()  [unwired: 2 in, 2 out]
                n301 = Increment(x=w460) -> (x+1=w458:i32)
                n302 = local write "Meas N"(w458) -> ()
                n303 = local read "WL: NML Only"() -> (w456:i32)
                n304 = local read "FW inTest"() -> (w457:u16)
                n305 = local write "All Results"(dbl[][][] [] ("All Results")) -> ()
                n306 = local write "FW"(w457) -> ()
                n307 = local write "NML_WL"(w456) -> ()
              }
            }
          }
        }
      }
      frame #7 {
        # "3-31-17, wavelength\nconfiguration"
        n308 = case shown="True" "Verify WavL" {
          frame False {
          }
          frame True {
            n309 = stacked-sequence {
              frame #0 {
                w463 = FALSE ("Restart Test")
                # "Indicators for signaling"
                # "Disable Verify Wavelength button"
                n310 = local read "DUT Count"() -> (w470:i32)
                n311 = local write "Re-conf Lambda"(w463) -> ()
                n312 = local write "Ready"(w463) -> ()
                n313 = local write "Busy"(TRUE ("Busy")) -> ()
                n314 = property on="DUT Count" class="Ring (strict)"("DisabledEnum"=T3."Disabled and Grayed Out" ("Disabled")) -> ()  [unwired: 2 in, 2 out]
                n315 = property on="Start Test" class="Bool (strict)"("DisabledEnum"=T3."Disabled and Grayed Out" ("Disabled")) -> ()  [unwired: 2 in, 2 out]
                n316 = Initialize Array(0 ("element"), w470) -> (→"Lambda, nm":i32[])
                n317 = property on="Verify WavL" class="Bool"("DisabledEnum"=T3."Disabled and Grayed Out" ("Disabled")) -> ()  [unwired: 2 in, 2 out]
                n318 = local write "Msg"("Resetting Power Supplies" ("Msg")) -> ()
              }
              frame #1 {
                w483 = "\r\n"
                # "Turn on active power supplies"
                n319 = local read "COMs"() -> (w478:refnum<visa-resource-name>[])
                n320 = local read "Com Open"() -> (w477:bool[])
                n321 = local read "Enable"() -> (w476:bool[])
                n322 = local read "error"() -> (w475:errorcluster)
                n323 = local read "Supply-PM Count"() -> (w472:i32)
                n324 = Concatenate Strings("*CLS" ("write buffer"), w483, "APPL P6V, 5.25, 4.0" ("write buffer"), w483, "APPL P25V, 24.0, 1.0" ("write buffer"), w483, "OUTPut:STATe ON" ("write buffer"), w483) -> (w474:string)
                n325 = for {
                  N: w472 -> [_]
                  tunnel: w478 -> [w492]
                  tunnel: w477 -> [w491]
                  tunnel: w476 -> [w490]
                  shift-right: [w487] -> w473
                  shift-left: w475 -> [w489]
                  tunnel: w474 -> [w488]
                  i -> [w486]
                  n326 = local read "DUT Count"() -> (w484:i32)
                  n327 = Add(x=w484, y=w486) -> (x+y=w485:i32)
                  n328 = Index Array(array=w492, index=w485) -> (element=w496:refnum<visa-resource-name>)
                  n329 = Index Array(array=w491, index=w485) -> (element=w494:bool)
                  n330 = Index Array(array=w490, index=w485) -> (element=w493:bool)
                  n331 = And(x=w494, y=w493) -> (x .and. y?=w495:bool)
                  n332 = case shown="True" w495 {
                    tunnel: w496 -> [_ w502]
                    tunnel: w489 -> [w497 w500]
                    tunnel: w488 -> [_ w499]
                    tunnel: [w497 w498] -> w487
                    frame False {
                    }
                    frame True {
                      n333 = call "PS_ManCMD.vi"("Power Sup: T-On/F-Off"=TRUE, "error in"=w500, "Command"=w499, "VISA resource name"=w502) -> ("error out"=w498:errorcluster)  [unwired: 1 in]
                    }
                  }
                }
                n334 = local write "error"(w473) -> ()
              }
              frame #2 {
                n335 = Wait (ms)(milliseconds to wait=u32 3000) -> ()  [unwired: 1 out]
              }
              frame #3 {
                # "Check if a connection is made"
                # "3-31-17, added\n\nSet lambda to\npower meter by system\nusing controller info.\n\nUnit under test needs\nto be connected in\nsequential order, e.g., 1,2,3,4or 1,2,3, or 1, 2 or 1, but not in alternating or\nnon-sequential order."
                n336 = local read "DUT Count"() -> (w505:i32)
                n337 = for {
                  N: w505 -> [_]
                  shift-right: [w506] -> _
                  shift-left: FALSE -> [w507]
                  i -> [w508]
                  n338 = stacked-sequence {
                    tunnel: w508 -> [w509 w529 w549]
                    tunnel: w507 -> [_ _ w532]
                    tunnel: [_ _ w530] -> w506
                    frame #0 {
                      n339 = Increment(x=w509) -> (x+1=w510:i32)
                      n340 = Number To Decimal String(number=w510) -> (decimal integer string=w511:string)  [unwired: 1 in]
                      n341 = Concatenate Strings("Verifying wavelength for DUT " ("Msg"), w511) -> (w513:string)
                      n342 = local write "Msg"(w513) -> ()
                    }
                    frame #1 {
                      # "Send request to read controller board info"
                      # "NML FW command"
                      # "WSD FW command"
                      # "FW in Test\n0=WSD (dark) board\n1=NML (light) board"
                      n343 = local read "FW inTest"() -> (w527:u16)
                      n344 = Equal To 0?(x=w527) -> (x = 0?=w526:bool)
                      n345 = Select(t="@NVstatus#" ("string"), s=w526, f="@status#" ("string")) -> (s? t:f=w528:string)
                      n346 = local read "COMs"() -> (w517:refnum<visa-resource-name>[])
                      n347 = local read "error"() -> (w523:errorcluster)
                      n348 = Index Array(array=w517, index=w529) -> (element=w516:refnum<visa-resource-name>)
                      n349 = call "Com_Cmd_RevA.vi"("Timeout"=2000, "Query"=TRUE, "error in"=w523, "Delay, ms"=u32 700, "write buffer"=w528, "VISA"=w516) -> ("error out"=w522:errorcluster, "read buffer"=w519:string, "Timeout"=w514:bool, "return count"=w520:u32)  [unwired: 2 out]
                      n350 = local write "Timeout"(w514) -> ()
                      n351 = local write "read buffer"(w519) -> ()
                      n352 = local write "work buffer"(w519) -> ()
                      n353 = local write "Bytes Rcvd"(w520) -> ()
                      n354 = local write "error"(w522) -> ()
                    }
                    frame #2 {
                      # "FW in Test\n0=WSD (dark) board\n1=NML (light) board"
                      # "Replaced subVI CHECK LAMBDA&CONCT with PM LAMBDA&CONCT"
                      # "From Check Lambda&Conct subVI:\n\"Red\"(newNMLFW)=\"1\"(WSD FW)=635\n\"780\"(newNML FW)=\"2\"(WSD FW)=780\n\"850\"(newNML FW)=\"3\"(WSD FW)=850\n\"None\"=\"0\"=0\n\"Highest\"=(OldRed, oldNML FW)=1\nError=No Connect=2"
                      # "8-25-17\nadded conditonal"
                      # "8-25-2017"
                      # "Collect lambda\nand display"
                      # "Identify and collect wavelength info"
                      n355 = local read "work buffer"() -> (w535:string)
                      n356 = local read "FW inTest"() -> (w536:u16)
                      n357 = case shown="1" w536 {
                        tunnel: [w555 w575] -> w546
                        tunnel: [w554 w574] -> w545
                        tunnel: [w553 w573] -> w544
                        tunnel: [w552 w572] -> w543
                        tunnel: [w551 w571] -> w542
                        tunnel: w535 -> [w550 w570]
                        frame 0, Default {
                          w560 = "Highest" ("regular expression")
                          w567 = "3" ("regular expression")
                          w566 = "2" ("regular expression")
                          w563 = "1" ("regular expression")
                          w562 = "0" ("regular expression")
                          # "NML old firmware for red"
                          # "Keep the 5th case (old FW for red) for both WSD and NML"
                          # "WSD"
                          # "WSD 3= 850"
                          # "WSD 2=780"
                          # "WSD 1=Red=635"
                          # "WSD 0=None, need to set lambda"
                          n358 = Match Pattern(string=w550, regular expression="WAVE:") -> (after substring=w557:string)  [unwired: 1 in, 3 out]
                          n359 = Match Pattern(string=w557, regular expression=",") -> (before substring=w569:string)  [unwired: 1 in, 3 out]
                          n360 = Match Pattern(string=w569, regular expression=w563) -> (match substring=w564:string)  [unwired: 1 in, 3 out]
                          n361 = Match Pattern(string=w569, regular expression=w560) -> (match substring=w559:string)  [unwired: 1 in, 3 out]
                          n362 = Match Pattern(string=w569, regular expression=w562) -> (match substring=w561:string)  [unwired: 1 in, 3 out]
                          n363 = Match Pattern(string=w569, regular expression=w566) -> (match substring=w565:string)  [unwired: 1 in, 3 out]
                          n364 = Match Pattern(string=w569, regular expression=w567) -> (match substring=w568:string)  [unwired: 1 in, 3 out]
                          n365 = Equal?(x=w560, y=w559) -> (x = y?=w551:bool)
                          n366 = Equal?(x=w563, y=w564) -> (x = y?=w554:bool)
                          n367 = Equal?(x=w566, y=w565) -> (x = y?=w553:bool)
                          n368 = Equal?(x=w567, y=w568) -> (x = y?=w552:bool)
                          n369 = Equal?(x=w562, y=w561) -> (x = y?=w555:bool)
                        }
                        frame 1 {
                          (unwired) "Highest" ("regular expression")
                          w577 = "Wavelength" ("regular expression")
                          w584 = "850" ("regular expression")
                          w583 = "780" ("regular expression")
                          w580 = "Red" ("regular expression")
                          w579 = "None" ("regular expression")
                          # "NML old firmware for red"
                          # "NML 850"
                          # "NML 780"
                          # "NML Red=635"
                          # "NML none - need to set lambda"
                          # "NML"
                          n370 = Match Pattern(string=w570, regular expression=w580) -> (match substring=w581:string)  [unwired: 1 in, 3 out]
                          n371 = Match Pattern(string=w570, regular expression=w577) -> (match substring=w576:string)  [unwired: 1 in, 3 out]
                          n372 = Match Pattern(string=w570, regular expression=w579) -> (match substring=w578:string)  [unwired: 1 in, 3 out]
                          n373 = Match Pattern(string=w570, regular expression=w583) -> (match substring=w582:string)  [unwired: 1 in, 3 out]
                          n374 = Match Pattern(string=w570, regular expression=w584) -> (match substring=w585:string)  [unwired: 1 in, 3 out]
                          n375 = Equal?(x=w579, y=w578) -> (x = y?=w575:bool)
                          n376 = Equal?(x=w580, y=w581) -> (x = y?=w574:bool)
                          n377 = Equal?(x=w583, y=w582) -> (x = y?=w573:bool)
                          n378 = Equal?(x=w584, y=w585) -> (x = y?=w572:bool)
                          n379 = Equal?(x=w577, y=w576) -> (x = y?=w571:bool)
                        }
                      }
                      n380 = local read "Supply-PM Count"() -> (w534:i32)
                      n381 = local read "DUT Count"() -> (w533:i32)
                      n382 = local read "error"() -> (w537:errorcluster)
                      n383 = control-ref of="Msg"() -> (w540:refnum<vi>)
                      n384 = control-ref of="COMs"() -> (w541:refnum<vi>)
                      n385 = call "PMLambda-Conct Rev A.vi"("Case0:NewFWNone"=w546, "Case1:NewFWRed"=w545, "Case2:NewFW780"=w544, "Case3:NewFW850"=w543, "Case4:OldFWRed\nElse5:FW error"=w542, "error in"=w537, "Supply Cnt"=w534, "N Systems"=w533, "COM Ref In"=w541, "Msg Ref In"=w540, "Loop Index"=w549) -> ("Re-conf Lambda?"=w531:bool, "Lambda, nm"=w539:i32, "error out"=w538:errorcluster)  [unwired: 6 in]
                      n386 = local read "Lambda, nm"() -> (w547:i32[])
                      n387 = local write "error"(w538) -> ()
                      n388 = Or(x=w532, y=w531) -> (x .or. y?=w530:bool)
                      n389 = Replace Array Subset(array=w547, new element=w539, index=w549) -> (w548:i32[])
                      n390 = local write "Re-conf Lambda"(w530) -> ()
                      n391 = local write "Lambda, nm"(w548) -> ()
                    }
                  }
                }
              }
              frame #4 {
                n392 = local read "Re-conf Lambda"() -> (w586:bool)
                n393 = case shown="False" w586 {
                  frame False {
                    # "From Check Lambda&Conct subVI:\n\"Red\"(newNMLFW)=\"1\"(WSD FW)=635\n\"780\"(newNML FW)=\"2\"(WSD FW)=780\n\"850\"(newNML FW)=\"3\"(WSD FW)=850\n\"None\"=\"0\"=0\n\"Highest\"=(OldRed, oldNML FW)=1\nError=No Connect=2"
                    # "4-17-17:\n-Connection is fine from previous step.\n-Check color, if all red or all non-red\n-Check firmware and select parameter\nlist based on color type of the mixture"
                    n394 = local read "DUT Count"() -> (w590:i32)
                    n395 = local read "Lambda, nm"() -> (w591:i32[])
                    n396 = local read "error"() -> (w588:errorcluster)
                    n397 = call "Check WavL Type(SubVI).vi"("N systems"=w590, "Lambda, nm"=w591, "error in"=w588) -> ("all NonRed"=w595:bool, "all Red"=w594:bool, "all NewRed"=w593:bool, "all OldRed"=w592:bool, "error out"=w589:errorcluster)  [unwired: 8 in]
                    n398 = local write "error"(w589) -> ()
                    n399 = case shown="False" w595 {
                      tunnel: [w600 FALSE] -> w587
                      tunnel: w590 -> [w599 _]
                      tunnel: w594 -> [w598 _]
                      tunnel: w593 -> [w597 _]
                      tunnel: w592 -> [w596 _]
                      frame False {
                        n400 = case shown="True" w598 {
                          tunnel: [TRUE ("Restart Test") w624] -> w600
                          tunnel: w599 -> [_ w623]
                          tunnel: w597 -> [_ w622]
                          tunnel: w596 -> [_ w621]
                          frame False {
                            w606 = "\r"
                            # "Unquailified = mix red and non-red"
                            # "PSs off"
                            # "click or close to \nbe true"
                            # "throw error msg"
                            n401 = local read "Supply-PM Count"() -> (w601:i32)
                            n402 = local read "error"() -> (w603:errorcluster)
                            n403 = for {
                              N: w601 -> [_]
                              shift-right: [w616] -> w602
                              shift-left: w603 -> [w617]
                              i -> [w615]
                              n404 = local read "DUT Count"() -> (w613:i32)
                              n405 = local read "COMs"() -> (w618:refnum<visa-resource-name>[])
                              n406 = Add(x=w613, y=w615) -> (x+y=w614:i32)
                              n407 = Index Array(array=w618, index=w614) -> (element=w620:refnum<visa-resource-name>)
                              n408 = call "PS_ManCMD.vi"("Power Sup: T-On/F-Off"=FALSE, "error in"=w617, "VISA resource name"=w620) -> ("error out"=w616:errorcluster)  [unwired: 2 in]
                            }
                            n409 = local write "Msg"("Power Supplies off.  Waiting to reconfigue..." ("Msg")) -> ()
                            n410 = Concatenate Strings("Error! " ("string"), w606, "Mixture contains Red and Non-Red laser diodes." ("string"), w606, "Connect only Red or only Non-Red, and reconfigure." ("string"), w606) -> (w610:string)
                            n411 = call "Display Message to User3"("error in (no error)"=w602, "Enable"=TRUE, "Message"=w610) -> ("error out"=w609:errorcluster)  [unwired: 7 in, 1 out]
                            n412 = local write "error"(w609) -> ()
                          }
                          frame True {
                            n413 = case shown="False" w622 {
                              tunnel: [w627 FALSE] -> w624
                              tunnel: w623 -> [w626 _]
                              tunnel: w621 -> [w625 _]
                              frame False {
                                n414 = case shown="True" w625 {
                                tunnel: [TRUE ("Enable") FALSE] -> w627
                                tunnel: w626 -> [_ w648]
                                frame False {
                                w633 = "\r"
                                # "Unquailified = mix old and new firmwares for red"
                                # "PSs off"
                                # "throw error msg"
                                n415 = local read "Supply-PM Count"() -> (w628:i32)
                                n416 = local read "error"() -> (w630:errorcluster)
                                n417 = for {
                                N: w628 -> [_]
                                shift-right: [w643] -> w629
                                shift-left: w630 -> [w644]
                                i -> [w642]
                                n418 = local read "DUT Count"() -> (w640:i32)
                                n419 = local read "COMs"() -> (w645:refnum<visa-resource-name>[])
                                n420 = Add(x=w640, y=w642) -> (x+y=w641:i32)
                                n421 = Index Array(array=w645, index=w641) -> (element=w647:refnum<visa-resource-name>)
                                n422 = call "PS_ManCMD.vi"("Power Sup: T-On/F-Off"=FALSE, "error in"=w644, "VISA resource name"=w647) -> ("error out"=w643:errorcluster)  [unwired: 2 in]
                                }
                                n423 = local write "Msg"("Power Supplies off.  Waiting to reconfigue..." ("Msg")) -> ()
                                n424 = Concatenate Strings("Error! " ("string"), w633, "Different firmwares are in used for red laser diode." ("string"), w633, "Reload firmware and reconfigure." ("string"), w633) -> (w637:string)
                                n425 = call "Display Message to User4"("error in (no error)"=w629, "Enable"=TRUE, "Message"=w637) -> ("error out"=w636:errorcluster)  [unwired: 7 in, 1 out]
                                n426 = local write "error"(w636) -> ()
                                }
                                frame True {
                                # "Old NML firmware is for red only"
                                # "All on old firmware for red"
                                n427 = for {
                                N: w648 -> [_]
                                i -> [w651]
                                n428 = local read "Lambda, nm"() -> (w653:i32[])
                                n429 = Replace Array Subset(array=w653, new element=635 ("new element/subarray"), index=w651) -> (w652:i32[])
                                n430 = local write "Lambda, nm"(w652) -> ()
                                }
                                }
                                }
                              }
                              frame True {
                                # "All on new NML/WSD firmware for red"
                              }
                            }
                          }
                        }
                      }
                      frame True {
                        # "All on new firmware for 780 & 850 (Non-Red)"
                      }
                    }
                    n431 = local write "Re-conf Lambda"(w587) -> ()
                  }
                  frame True {
                    # "Connection has problem before colors can be checked.  Powers off and test restarted by previous step."
                  }
                }
              }
              frame #5 {
                # "If connection and color checks pass, set wavelengths."
                # "4-20-17, added"
                n432 = local read "Re-conf Lambda"() -> (w656:bool)
                n433 = case shown="False" w656 {
                  frame False {
                    n434 = local read "DUT Count"() -> (w657:i32)
                    n435 = for {
                      N: w657 -> [_]
                      i -> [w662]
                      w660 = FALSE ("Set Lambda\nSingle CH(F)\nDual CHs(T)")
                      # "Select channel: F=CH1, T=CH2"
                      # "Set lambda to PM for each UUT"
                      # "Select PM and CH# by unit position along\nwith corresponding wavelength (lambda)."
                      n436 = Quotient & Remainder(x=w662, y=2) -> (x-y*floor(x/y)=w665:i32, floor(x/y)=w659:i32)
                      n437 = local read "Lambda, nm"() -> (w672:i32[])
                      n438 = Increment(x=w659) -> (x+1=w658:i32)
                      n439 = Number To Boolean Array(number=w665) -> (Boolean array=w664:bool[])
                      n440 = Index Array(array=w664, index=0) -> (element=w661:bool)
                      n441 = Index Array(array=w672, index=w662) -> (element=w671:i32)
                      n442 = local read "reference Out"() -> (w669:refnum<k24>)
                      n443 = local read "error"() -> (w668:errorcluster)
                      n444 = call "NewPort_PM_USB_Read-Set.vi"("reference"=w669, "USB Address"=w658, "Read Power(F)\nSet Lambda(T)"=TRUE ("Read Power(T)\nSet Lambda(F)"), "Single: CH\nLambda (nm)"=w671, "error in"=w668, "Pick Single CH \nCH1(F)\nCH2(T)"=w661, "Set Lambda\nSingle CH(F)\nDual CHs(T)"=w660, "Read Power\nSingle CH(F)\nDual CHs(T)"=w660) -> ("error out"=w667:errorcluster)  [unwired: 6 in, 1 out]
                      n445 = local write "error"(w667) -> ()
                    }
                  }
                  frame True {
                    # "Test restarted due to either not pass connection check or color type check."
                  }
                }
              }
              frame #6 {
                # "5-16-17, revised\n6-29-17, revised"
                # "Reset buttons and flags"
                n446 = local read "Re-conf Lambda"() -> (w673:bool)
                n447 = case shown="True" w673 {
                  frame False {
                    w678 = T3."Enabled" ("Disabled")
                    # "8-23-17"
                    # "5-16-17 added"
                    # "5-16-17 added"
                    # "5-16-17 added"
                    # "Enable Test Start button"
                    # "Signal wavelength is set"
                    n448 = local write "Ready"(TRUE ("Ready")) -> ()
                    n449 = local write "Busy"(FALSE ("Busy")) -> ()
                    n450 = property on="New File" class="Bool (strict)"("DisabledEnum"=w678) -> ()  [unwired: 2 in, 2 out]
                    n451 = local write "InitCriteria"(TRUE ("InitCriteria")) -> ()
                    n452 = property on="Start Test" class="Bool (strict)"("DisabledEnum"=w678) -> ()  [unwired: 2 in, 2 out]
                    n453 = local write "Msg"("Wavelengths are set.  Ready to Test." ("Msg")) -> ()
                  }
                  frame True {
                    # "Resume Verify Lambda button"
                    # "Resume N systems selection, restart test"
                    n454 = property on="DUT Count" class="Ring (strict)"("DisabledEnum"=T3."Enabled" ("Disabled")) -> ()  [unwired: 2 in, 2 out]
                    n455 = local write "Busy"(FALSE ("Busy")) -> ()
                    n456 = property on="Verify WavL" class="Bool"("DisabledEnum"=T3."Enabled" ("Disabled")) -> ()  [unwired: 2 in, 2 out]
                    n457 = local write "Msg"("Error in setting wavelength.  Waiting to reconfigure..." ("Msg")) -> ()
                  }
                }
              }
            }
          }
        }
      }
      frame #8 {
        # "Re-initialize UUT review indicators if wavelength (Lambda) verification passed."
        n458 = local read "InitCriteria"() -> (w683:bool)
        n459 = case shown="True" w683 {
          frame False {
          }
          frame True {
            # "Initialize criteria and check arrays."
            # "6-29-17 Data status indicator"
            # "6-29-17 Data status indicator"
            # "6-29-17 added\nInitialize True array for \nchecking data status"
            # "6-29-17 added\nInitialize True array for \nchecking data status"
            n460 = local read "DUT Count"() -> (w689:i32)
            n461 = local read "FW Prm"() -> (w700:string[])
            n462 = Array Size(array=w700) -> (size(s)=w690:i32)
            n463 = Initialize Array(TRUE, w690, w689) -> (w688:bool[][])
            n464 = Initialize Array(FALSE, w690, w689) -> (w687:bool[][])
            n465 = local write "MCUTrue"(w688) -> ()
            n466 = local write "MCUTrue2"(w688) -> ()
            n467 = Initialize Array("N/A", w690, w689) -> (w695:string[][])
            n468 = local write "MCUReview2"(w687) -> ()
            n469 = local write "MCUReview"(w687) -> ()
            n470 = local write "MCUCheck"(w695) -> ()
            n471 = local read "Sys Prm"() -> (w701:string[])
            n472 = Array Size(array=w701) -> (size(s)=w691:i32)
            n473 = Initialize Array(TRUE, w691, w689) -> (w686:bool[][])
            n474 = Initialize Array(FALSE, w691, w689) -> (w685:bool[][])
            n475 = local write "SysTrue2"(w686) -> ()
            n476 = local write "SysTrue"(w686) -> ()
            n477 = local write "InitCriteria"(FALSE ("InitCriteria")) -> ()
            n478 = Initialize Array("N/A", w691, w689) -> (w692:string[][])
            n479 = local write "SysReview2"(w685) -> ()
            n480 = local write "SysReview"(w685) -> ()
            n481 = local write "SysCheck"(w692) -> ()
          }
        }
      }
      frame #9 {
        # "Refresh indicators if # of systems changed\nor if at startup with first loop iteration."
        n482 = local read "Serial Numbers"() -> (w707:string[])
        n483 = local read "DUT Count Old"() -> (w710:i32)
        n484 = local read "DUT Count"() -> (w709:i32)
        n485 = local read "Serial"() -> (w706:string[])
        n486 = Not Equal?(x=w707, y=w706) -> (x != y?=w702:bool)
        n487 = Not Equal?(x=w709, y=w710) -> (x != y?=w704:bool)
        n488 = Equal To 0?(x=w708) -> (x = 0?=w703:bool)
        n489 = Compound Arithmetic op=OR(w702, w704, w703) -> (w705:bool)
        n490 = case shown="True" w705 {
          frame False {
          }
          frame True {
            w712 = 0 items=["1", "2", "3", "4", "5", "6", "7", "8"] ("System #")
            # "5-12-17 added"
            n491 = disable-structure shown="Disabled" {
              frame Disabled {
                # "Best to wait until data is \ncollected before updating\ngraphs and power\ncalculations.  - Dale"
                n492 = local write "Update Graph"(TRUE ("Update")) -> ()
              }
              frame Enabled {
              }
            }
            n493 = local read "Serial Numbers"() -> (w716:string[])
            n494 = local read "DUT Count"() -> (w711:i32)
            n495 = local write "Serial"(w716) -> ()
            n496 = for {
              N: w711 -> [_]
              tunnel: w716 -> [w723] mode=indexing
              i -> [w728]
              w726 = "                " ("String")
              n497 = String Subset(string=w723, length (rest)=16 ("length (rest)")) -> (substring=w721:string)  [unwired: 1 in]
              n498 = String Length(string=w721) -> (length=w725:i32)
              n499 = String Length(string=w726) -> (length=w727:i32)
              n500 = Subtract(x=w727, y=w725) -> (x-y=w724:i32)
              n501 = Replace Substring(2:w725, 3:w724, 4:w721, 5:w726) -> (1:w720:string)  [unwired: 1 out]
              n502 = property on="Time" class="XYGraph (strict)"("Active Plot"=w728, "Plot.Plot Name"=w720) -> ()  [unwired: 2 in, 2 out]
            }
            n503 = Array Subset(array=w716, index=0, length=w711) -> (w717:string[])
            n504 = property on="Display UUT #" class="Ring (strict)"("Strings []"=w717) -> ()  [unwired: 2 in, 2 out]
            n505 = local read "DUT Count"() -> (w713:i32)
            n506 = local write "Display UUT #"(w712) -> ()
            n507 = local write "DUT Selected"(w713) -> ()
            n508 = local write "DUT Count Old"(w713) -> ()
            n509 = property on="Time" class="XYGraph (strict)"("LegNumRows"=w713) -> ()  [unwired: 2 in, 2 out]
            n510 = Initialize Array(0 ("dimension size"), w713) -> (w715:i32[])
            n511 = local write "Points"(w715) -> ()
          }
        }
      }
      frame #10 {
        # "5-23-17 added condition statement for pause condition."
        # "Prepare for Test Startup"
        # "Check start status"
        n512 = local read "Start Test"() -> (w730:bool)
        n513 = local read "New Test"() -> (w729:bool)
        n514 = Not Equal?(x=w730, y=w729) -> (x != y?=w731:bool)
        n515 = case shown="True" w731 {
          frame False {
          }
          frame True {
            # "5-23-17 moved Prepped=F from outter\nframe to pause=0 true frame."
            n516 = local read "Start Test"() -> (w732:bool)
            n517 = local read "Start Test"() -> (w734:bool)
            n518 = local read "New File"() -> (w733:bool)
            n519 = And(x=w734, y=w733) -> (x .and. y?=w735:bool)
            n520 = case shown="True" w732 {
              frame False {
                n521 = property on="New File" class="Bool (strict)"("DisabledEnum"=T3."Enabled" ("Disabled")) -> ()  [unwired: 2 in, 2 out]
                n522 = local write "Pause"(TRUE ("Pause")) -> ()
                n523 = property on="Busy" class="Bool (strict)"("Blinking"=FALSE) -> ()  [unwired: 2 in, 2 out]
                n524 = property on="Verify WavL" class="Bool"("DisabledEnum"=T3."Enabled" ("Disabled")) -> ()  [unwired: 2 in, 2 out]
                n525 = property on="DUT Count" class="Ring (strict)"("DisabledEnum"=T3."Enabled" ("Disabled")) -> ()  [unwired: 2 in, 2 out]
              }
              frame True {
                # "5-23-17 added"
                n526 = local read "Pause"() -> (w742:bool)
                n527 = case shown="False" w742 {
                  frame False {
                    # "Sttr Ref0 is for refresh shutter time parameters only"
                    # "PSs off"
                    # "5-23-17 moved Prepped=F from outer frame to here."
                    # "5-16-17, Disable&Greyed Out New File"
                    # "The 1st time Test starts"
                    n528 = Get Date/Time In Seconds() -> (seconds since 1Jan1904=w747:timestamp)
                    n529 = local write "Start Time"(w747) -> ()
                    n530 = property on="Busy" class="Bool (strict)"("Blinking"=TRUE) -> ()  [unwired: 2 in, 2 out]
                    n531 = local write "Shtr Ref0"(w747) -> ()
                    n532 = local write "Soak Complete"(FALSE ("Started")) -> ()
                    n533 = local read "Supply-PM Count"() -> (w743:i32)
                    n534 = local write "Msg"("Power Supplies off for prep..." ("Msg")) -> ()
                    n535 = local read "error"() -> (w744:errorcluster)
                    n536 = for {
                      N: w743 -> [_]
                      shift-right: [w754] -> w745
                      shift-left: w744 -> [w755]
                      i -> [w753]
                      n537 = local read "DUT Count"() -> (w751:i32)
                      n538 = local read "COMs"() -> (w756:refnum<visa-resource-name>[])
                      n539 = Add(x=w751, y=w753) -> (x+y=w752:i32)
                      n540 = Index Array(array=w756, index=w752) -> (element=w758:refnum<visa-resource-name>)
                      n541 = call "PS_ManCMD.vi"("Power Sup: T-On/F-Off"=FALSE, "error in"=w755, "VISA resource name"=w758) -> ("error out"=w754:errorcluster)  [unwired: 2 in]
                    }
                    n542 = property on="New File" class="Bool (strict)"("DisabledEnum"=T3."Disabled and Grayed Out" ("Disabled")) -> ()  [unwired: 2 in, 2 out]
                    n543 = local write "error"(w745) -> ()
                  }
                  frame True {
                    # "After a pause, Test re-starts and update time for recalculating\nprep time if prevously prep time isn't finished timing."
                    # "5-23-17 added"
                    n544 = Get Date/Time In Seconds() -> (seconds since 1Jan1904=w760:timestamp)
                    n545 = local write "Pause"(FALSE ("Pause")) -> ()
                    n546 = local write "Start Time"(w760) -> ()
                    n547 = property on="New File" class="Bool (strict)"("DisabledEnum"=T3."Disabled and Grayed Out" ("Disabled")) -> ()  [unwired: 2 in, 2 out]
                  }
                }
              }
            }
            n548 = case shown="True" w735 {
              frame False {
                n549 = local write "SysFileDelete"(i16 0 ("SysDel")) -> ()
              }
              frame True {
                w782 = T2 [] ("Time")
                # "6-29-17 Data status indicator"
                # "6-29-17 Data status indicator"
                # "6-29-17 added\nInitialize True array for \nchecking data status"
                # "6-29-17 added\nInitialize True array for \nchecking data status"
                n550 = local read "DUT Count"() -> (w781:i32)
                n551 = disable-structure shown="Disabled" {
                  frame Disabled {
                    w795 = FALSE ("Power Sup: T-On/F-Off")
                    # "11-1-17, added"
                    # "PSs off"
                    # "11-1-17 Added"
                    n552 = local read "COMs"() -> (w794:refnum<visa-resource-name>[])
                    n553 = Index Array(array=w794, index=4) -> (element=w797:refnum<visa-resource-name>)
                    n554 = local read "error"() -> (w790:errorcluster)
                    n555 = call "PS_ManCMD.vi"("Power Sup: T-On/F-Off"=w795, "error in"=w790, "VISA resource name"=w797) -> ("error out"=w791:errorcluster)  [unwired: 2 in]
                    n556 = Index Array(array=w794, index=5) -> (element=w796:refnum<visa-resource-name>)
                    n557 = call "PS_ManCMD.vi"("Power Sup: T-On/F-Off"=w795, "error in"=w791, "VISA resource name"=w796) -> ("error out"=w788:errorcluster)  [unwired: 2 in]
                    n558 = local write "Msg"("Power Supplies off for prep..." ("Msg")) -> ()
                    n559 = local write "error"(w788) -> ()
                    n560 = Get Date/Time In Seconds() -> (seconds since 1Jan1904=w800:timestamp)
                    n561 = local write "Soak Complete"(FALSE ("Started")) -> ()
                    n562 = local write "Start Time"(w800) -> ()
                    n563 = local write "Shtr Ref0"(w800) -> ()
                    n564 = property on="Busy" class="Bool (strict)"("Blinking"=TRUE) -> ()  [unwired: 2 in, 2 out]
                  }
                  frame Enabled {
                  }
                }
                n565 = local read "Meas N"() -> (w780:i32)
                n566 = Initialize Array(0.0 ("element"), w781, 1 ("dimension size"), w780) -> (w787:dbl[][][])
                n567 = Initialize Array(0 ("dimension size"), w781) -> (w786:i32[])
                n568 = local write "SysFileDelete"(w781) -> ()
                n569 = local write "All Results"(w787) -> ()
                n570 = local write "Points"(w786) -> ()
                n571 = local write "Time"(w782) -> ()
                n572 = local write "Time 2"(w782) -> ()
                n573 = local read "FW Prm"() -> (w778:string[])
                n574 = local read "DUT Count"() -> (w767:i32)
                n575 = Array Size(array=w778) -> (size(s)=w768:i32)
                n576 = Initialize Array(TRUE, w768, w767) -> (w766:bool[][])
                n577 = Initialize Array(FALSE, w768, w767) -> (w765:bool[][])
                n578 = local write "MCUTrue"(w766) -> ()
                n579 = local write "MCUTrue2"(w766) -> ()
                n580 = Initialize Array("N/A", w768, w767) -> (w773:string[][])
                n581 = local write "MCUReview2"(w765) -> ()
                n582 = local write "MCUReview"(w765) -> ()
                n583 = local write "MCUCheck"(w773) -> ()
                n584 = local read "Sys Prm"() -> (w779:string[])
                n585 = Array Size(array=w779) -> (size(s)=w769:i32)
                n586 = Initialize Array(TRUE, w769, w767) -> (w764:bool[][])
                n587 = Initialize Array(FALSE, w769, w767) -> (w763:bool[][])
                n588 = local write "SysTrue2"(w764) -> ()
                n589 = local write "SysTrue"(w764) -> ()
                n590 = Initialize Array("N/A", w769, w767) -> (w770:string[][])
                n591 = local write "SysReview2"(w763) -> ()
                n592 = local write "SysReview"(w763) -> ()
                n593 = local write "SysCheck"(w770) -> ()
              }
            }
            n594 = local read "Start Test"() -> (w736:bool)
            n595 = local write "New Test"(w736) -> ()
          }
        }
      }
      frame #11 {
        # "Check to see if soak interval completed."
        n596 = local read "Soak Complete"() -> (w803:bool)
        n597 = local read "Start Test"() -> (w801:bool)
        n598 = Not(x=w803) -> (.not. x?=w802:bool)
        n599 = Compound Arithmetic op=AND(w802, w801) -> (w804:bool)
        n600 = case shown="True" w804 {
          frame False {
          }
          frame True {
            n601 = local read "Prep, min"() -> (w810:dbl)
            n602 = local read "Start Time"() -> (w808:timestamp)
            n603 = Multiply(x=w810, y=60.0) -> (x*y=w811:dbl)
            n604 = Get Date/Time In Seconds() -> (seconds since 1Jan1904=w805:timestamp)
            n605 = Add(x=w808, y=w811) -> (x+y=w806:timestamp)
            n606 = Greater?(x=w805, y=w806) -> (0:w807:bool)
            n607 = case shown="True" w807 {
              tunnel: w806 -> [w823 _]
              tunnel: w805 -> [w822 _]
              frame False {
                n608 = Subtract(x=w823, y=w822) -> (x-y=w821:dbl)
                n609 = Quotient & Remainder(x=w821, y=60.0) -> (x-y*floor(x/y)=w818:dbl, floor(x/y)=w819:dbl)
                n610 = Number To Decimal String(number=w819) -> (decimal integer string=w816:string)  [unwired: 1 in]
                n611 = Number To Decimal String(number=w818) -> (decimal integer string=w814:string)  [unwired: 1 in]
                n612 = Concatenate Strings("Soaking in progress. Time to start is " ("Msg"), w816, " min " ("Msg"), w814, " sec " ("Msg")) -> (w812:string)
                n613 = local write "Msg"(w812) -> ()
              }
              frame True {
                n614 = property on="Busy" class="Bool (strict)"("Blinking"=FALSE) -> ()  [unwired: 2 in, 2 out]
                n615 = local write "Soak Complete"(TRUE ("Prepped")) -> ()
                n616 = local write "PS RST"(TRUE ("PS RST")) -> ()
                n617 = local write "Msg"("Soaking is done" ("Msg")) -> ()
              }
            }
          }
        }
      }
      frame #12 {
        # "Reset Power Supplies"
        n618 = local read "PS RST"() -> (w828:bool)
        n619 = Compound Arithmetic op=OR(w828, "Reset PSs") -> (w830:bool)
        n620 = case shown="True" w830 {
          frame False {
          }
          frame True {
            n621 = stacked-sequence {
              frame #0 {
                n622 = local write "Busy"(TRUE ("Active")) -> ()
                n623 = local write "Msg"("Resetting Power Supplies" ("Msg")) -> ()
              }
              frame #1 {
                # "Turn on/reset power supplies"
                n624 = local read "Supply-PM Count"() -> (w833:i32)
                n625 = local read "error"() -> (w834:errorcluster)
                n626 = for {
                  N: w833 -> [_]
                  shift-right: [w853] -> w835
                  shift-left: w834 -> [w854]
                  i -> [w852]
                  w844 = "\r\n"
                  n627 = local read "DUT Count"() -> (w839:i32)
                  n628 = local read "Com Open"() -> (w848:bool[])
                  n629 = local read "COMs"() -> (w855:refnum<visa-resource-name>[])
                  n630 = local read "Enable"() -> (w849:bool[])
                  n631 = Add(x=w839, y=w852) -> (x+y=w847:i32)
                  n632 = Index Array(array=w855, index=w847) -> (element=w856:refnum<visa-resource-name>)
                  n633 = Index Array(array=w848, index=w847) -> (element=w851:bool)
                  n634 = Index Array(array=w849, index=w847) -> (element=w850:bool)
                  n635 = Concatenate Strings("*CLS" ("write buffer"), w844, "APPL P6V, 5.25, 4.0" ("write buffer"), w844, "APPL P25V, 24.0, 1.0" ("write buffer"), w844, "OUTPut:STATe ON" ("write buffer"), w844) -> (w840:string)
                  n636 = And(x=w851, y=w850) -> (x .and. y?=w846:bool)
                  n637 = case shown="True" w846 {
                    tunnel: w856 -> [_ w862]
                    tunnel: w854 -> [w857 w860]
                    tunnel: [w857 w859] -> w853
                    tunnel: w840 -> [_ w858]
                    frame False {
                    }
                    frame True {
                      n638 = call "PS_ManCMD.vi"("Power Sup: T-On/F-Off"=TRUE, "error in"=w860, "Command"=w858, "VISA resource name"=w862) -> ("error out"=w859:errorcluster)  [unwired: 1 in]
                    }
                  }
                }
                n639 = local write "Msg"("Waiting to power up..." ("Msg")) -> ()
                n640 = local write "Busy"(FALSE ("Active")) -> ()
                n641 = local write "PS RST"(FALSE ("PS RST")) -> ()
                n642 = local write "error"(w835) -> ()
              }
              frame #2 {
                n643 = Wait (ms)(milliseconds to wait=u32 3000) -> ()  [unwired: 1 out]
              }
              frame #3 {
                # "5-25-17 Revised\nResult of adding is the start of every shutter open time interval in shutter control period."
                # "Time PS on + offset = after prep time=shutter control reference time begins"
                n644 = local read "Warm-up, min"() -> (w866:dbl)
                n645 = Get Date/Time In Seconds() -> (seconds since 1Jan1904=w868:timestamp)
                n646 = Multiply(x=w866, y=60.0) -> (x*y=w865:dbl)
                n647 = Add(x=w868, y=w865) -> (x+y=w864:timestamp)
                n648 = local write "Shtr Ref Time"(w864) -> ()
              }
            }
          }
        }
      }
      frame #13 {
        # "When shutter time parameters change during test,\nreset shutter control initial reference time."
        n649 = local read "Shtr Ctrl Close, Seconds"() -> (w873:dbl)
        n650 = local read "Shtr Ctrl Open, min"() -> (w875:dbl)
        n651 = local read "ShtrCtrl Close Old"() -> (w872:dbl)
        n652 = local read "ShtrCtrl Open Old"() -> (w874:dbl)
        n653 = Not Equal?(x=w873, y=w872) -> (x != y?=w870:bool)
        n654 = Not Equal?(x=w875, y=w874) -> (x != y?=w871:bool)
        n655 = Or(x=w871, y=w870) -> (x .or. y?=w869:bool)
        n656 = case shown="True" w869 {
          frame False {
          }
          frame True {
            # "Sttr Ref0 is for refresh shutter time parameters only"
            n657 = local read "Warm-up, min"() -> (w883:dbl)
            n658 = local read "Prep, min"() -> (w886:dbl)
            n659 = Multiply(x=w886, y=60.0) -> (x*y=w882:dbl)
            n660 = Multiply(x=w883, y=60.0) -> (x*y=w881:dbl)
            n661 = local read "Shtr Ctrl Close, Seconds"() -> (w887:dbl)
            n662 = local read "Shtr Ctrl Open, min"() -> (w888:dbl)
            n663 = Add(x=w882, y=w881) -> (x+y=w879:dbl)
            n664 = local read "Shtr Ref0"() -> (w880:timestamp)
            n665 = Get Date/Time In Seconds() -> (seconds since 1Jan1904=w876:timestamp)
            n666 = Add(x=w880, y=w879) -> (x+y=w878:timestamp)
            n667 = Greater?(x=w876, y=w878) -> (0:w877:bool)
            n668 = local write "ShtrCtrl Open Old"(w888) -> ()
            n669 = local write "ShtrCtrl Close Old"(w887) -> ()
            n670 = case shown="True" w877 {
              tunnel: w876 -> [_ w889]
              frame False {
                # "All time reference no change if time is less than Prep+Warm up"
              }
              frame True {
                # "Reset time reference\nif shutter time parameters\nchange after passing\nPrep+Warm up time"
                n671 = local write "Shtr Ref Time"(w889) -> ()
              }
            }
          }
        }
      }
      frame #14 {
        # "If no pause condition, check for test start conditions."
        n672 = local read "Pause"() -> (w890:bool)
        n673 = case shown="False" w890 {
          frame False {
            # "\"UUT Selected\" will start to increment\nonce data collection is initiated.   This\nincrementing will reset to -1 after all\nunits have been tested."
            # "Once the \"Start Test\" button is selected, \ndata collection will wait until soak time is\ncompleted and interval time has elapsed\nto change \"UUT Selected\" from maximum\nnumeric value (set at startup) to a value of\n-1.  This value kicks off data collection as \ninterpreted in the next sequence frame."
            n674 = local read "DUT Selected"() -> (w899:i32)
            n675 = local read "DUT Count"() -> (w898:i32)
            n676 = local read "Soak Complete"() -> (w891:bool)
            n677 = local read "Start Test"() -> (w895:bool)
            n678 = Get Date/Time In Seconds() -> (seconds since 1Jan1904=w901:timestamp)
            n679 = local read "Data Time"() -> (w900:timestamp)
            n680 = local read "Interval, Seconds"() -> (w896:dbl)
            n681 = Decrement(x=w898) -> (x-1=w897:i32)
            n682 = Add(x=w900, y=w896) -> (x+y=w902:timestamp)
            n683 = Greater Or Equal?(x=w899, y=w897) -> (x >= y?=w893:bool)
            n684 = Greater?(x=w901, y=w902) -> (0:w894:bool)
            n685 = Compound Arithmetic op=AND(w891, w895, w894, w893) -> (w892:bool)
            n686 = case shown="True" w892 {
              frame False {
              }
              frame True {
                # "Shtr Ref Time updated when soak time\nfinished.  Includes addition of warmup."
                # "Data Time updated at start of previous\ndata collection sequence (or at startup)."
                # "Assigning a negative one value to UUT Selected\nenables data collection to start in subsequent frame."
                # "Note\nContinuous shutter cycle control: \nlong opening (3min) and short closing (3sec)"
                # "5-5-17, change Auto from enable to disable and grey out\n5-23-17, change Auto back to enable"
                n687 = local write "DUT Selected"(-1 ("Sys in Test")) -> ()
                n688 = property on="Display Parameter" class="Ring (strict)"("DisabledEnum"=T3."Enabled" ("Disabled")) -> ()  [unwired: 2 in, 2 out]
                n689 = local write "Busy"(TRUE ("Active")) -> ()
                n690 = property on="Measure" class="Bool"("DisabledEnum"=T3."Disabled and Grayed Out" ("Disabled")) -> ()  [unwired: 2 in, 2 out]
                n691 = property on="Start Test" class="Bool (strict)"("DisabledEnum"=T3."Enabled" ("Disabled")) -> ()  [unwired: 2 in, 2 out]
                n692 = local write "Msg"("Collection Started" ("Msg")) -> ()
                n693 = local read "Data Time"() -> (w903:timestamp)
                n694 = local read "Shtr Ref Time"() -> (w906:timestamp)
                n695 = local read "Shtr Ctrl Open, min"() -> (w908:dbl)
                n696 = Multiply(x=w908, y=60.0) -> (x*y=w905:dbl)
                n697 = Add(x=w906, y=w905) -> (x+y=w904:timestamp)
                n698 = Greater?(x=w903, y=w904) -> (0:w910:bool)
                n699 = case shown="True" w910 {
                  frame False {
                  }
                  frame True {
                    # "Shutters open for\n3 minutes yet?"
                    # "5-18-17, added"
                    n700 = local write "Tpass Shtr Open"(TRUE ("Pass 3 Minute")) -> ()
                    n701 = local write "Shtr Open"(FALSE ("Sttrs Open")) -> ()
                  }
                }
              }
            }
          }
          frame True {
          }
        }
      }
      frame #15 {
        # "Enable data collection if UUT selected is equal to or less than total UUT Count."
        n702 = local read "Pause"() -> (w918:bool)
        n703 = case shown="False" w918 {
          frame False {
            # "\"UUT Selected\" starts out at \nmaximum value causing\nfalse case for inner case \nstructure to be selected until\nsoak and elaspe time satisfied\nthen \"UUT Selected\" will be set\nto -1 .  Then true case of inner\ncase structure will be selected."
            n704 = local read "DUT Selected"() -> (w921:i32)
            n705 = local read "DUT Count"() -> (w919:i32)
            n706 = Decrement(x=w919) -> (x-1=w920:i32)
            n707 = Less?(x=w921, y=w920) -> (x < y?=w922:bool)
            n708 = case shown="False" w922 {
              tunnel: w921 -> [_ w931]
              frame False {
                w924 = T3."Enabled" ("Disabled")
                # "5-5-17, 1st change from enable to\ndisable and grey out; 2nd change\nto disable this.  5-17-17 change back to enable.\n5-26-17 Disable Auto here."
                n709 = local read "Start Test"() -> (w923:bool)
                n710 = disable-structure shown="Enabled" {
                  frame Disabled {
                    n711 = property on="Start Test" class="Bool (strict)"("DisabledEnum"=T3."Enabled" ("Disabled")) -> ()  [unwired: 2 in, 2 out]
                  }
                  frame Enabled {
                  }
                }
                n712 = case shown="False" w923 {
                  frame False {
                    n713 = local write "Busy"(FALSE ("Active")) -> ()
                    n714 = local write "Msg"("Idle" ("Msg")) -> ()
                  }
                  frame True {
                  }
                }
                n715 = property on="Display Parameter" class="Ring (strict)"("DisabledEnum"=w924) -> ()  [unwired: 2 in, 2 out]
                n716 = property on="Measure" class="Bool"("DisabledEnum"=w924) -> ()  [unwired: 2 in, 2 out]
              }
              frame True {
                n717 = local read "Enable"() -> (w930:bool[])
                n718 = Increment(x=w931) -> (x+1=w928:i32)
                n719 = Index Array(array=w930, index=w928) -> (element=w929:bool)
                n720 = local write "DUT Selected"(w928) -> ()
                n721 = local write "Display UUT #"(w928) -> ()
                n722 = local write "Collect"(w929) -> ()
              }
            }
          }
          frame True {
          }
        }
      }
      frame #16 {
        # "Measure"
        n723 = local read "Collect"() -> (w934:bool)
        n724 = Or(x=w934, y="Measure") -> (x .or. y?=w932:bool)
        n725 = case shown="True" w932 {
          frame False {
          }
          frame True {
            n726 = stacked-sequence {
              frame #0 {
                w935 = dbl[] [] ("Ret Data")
                n727 = local write "MCU Data"(w935) -> ()
                n728 = local write "System Data"(w935) -> ()
                n729 = local write "Data Error"(FALSE ("Data Err")) -> ()
                n730 = local write "Busy"(TRUE ("Active")) -> ()
                n731 = local write "Msg"("Reading Controller Data" ("Msg")) -> ()
              }
              frame #1 {
                # "Get time stamp"
                n732 = Get Date/Time In Seconds() -> (seconds since 1Jan1904=w943:timestamp)
                n733 = local write "Data Time"(w943) -> ()
                n734 = Format Date/Time String(time format string (%c)="%m/%d/%y", seconds (now)=w943) -> (date/time string=w941:string)  [unwired: 1 in]
                n735 = Format Date/Time String(time format string (%c)="%H:%M:%S", seconds (now)=w943) -> (date/time string=w942:string)  [unwired: 1 in]
                n736 = local write "TimeS"(w942) -> ()
                n737 = local write "DateS"(w941) -> ()
              }
              frame #2 {
                # "NML"
                # "WSD"
                # "FW in Test\n0=WSD (dark) board\n1=NML (light) board"
                # "Send request to controller board"
                n738 = local read "FW inTest"() -> (w945:u16)
                n739 = Equal To 0?(x=w945) -> (x = 0?=w944:bool)
                n740 = Select(t="@NVstatus#" ("string"), s=w944, f="@status#" ("string")) -> (s? t:f=w948:string)
                n741 = local read "Display UUT #"() -> (w952:i32)
                n742 = local read "COMs"() -> (w951:refnum<visa-resource-name>[])
                n743 = local read "error"() -> (w959:errorcluster)
                n744 = Index Array(array=w951, index=w952) -> (element=w950:refnum<visa-resource-name>)
                n745 = call "Com_Cmd_RevA.vi"("Timeout"=2000, "Query"=TRUE, "error in"=w959, "Delay, ms"=u32 700, "write buffer"=w948, "VISA"=w950) -> ("error out"=w958:errorcluster, "read buffer"=w954:string, "Timeout"=w955:bool, "return count"=w956:u32)  [unwired: 2 out]
                n746 = local write "read buffer"(w954) -> ()
                n747 = local write "work buffer"(w954) -> ()
                n748 = local write "Timeout"(w955) -> ()
                n749 = local write "Bytes Rcvd"(w956) -> ()
                n750 = local write "error"(w958) -> ()
              }
              frame #3 {
                # "FW in Test\n0=WSD (dark) board\n1=NML (light) board"
                # "Verify Data"
                n751 = local read "FW inTest"() -> (w960:u16)
                n752 = case shown="1" w960 {
                  frame 0, Default {
                    # "WSD"
                    n753 = local read "FW ID"() -> (w964:string[])
                    n754 = Array Size(array=w964) -> (size(s)=w961:i32)
                    n755 = for {
                      N: w961 -> [_]
                      shift-right: [w966] -> w963
                      shift-left: FALSE ("Data Err") -> [w967]
                      tunnel: w964 -> [w965] mode=indexing
                      # "Verify microcontroller has all parameters that the array FW ID has,\nand extract the value for each parameter and store it in MCU data."
                      n756 = case shown="\"True\", Default" w965 {
                        tunnel: w965 -> [w976 w996]
                        tunnel: w967 -> [w978 w1009]
                        tunnel: [w977 w1008] -> w966
                        frame "FIRM:" {
                          w982 = -99999.999 ("default (0 dbl)")
                          # "Convert hex to decimal\nand will convert back to hex in saved file."
                          # "Extract firmware version hex\nafter ID and before comma"
                          # "Verify ID"
                          n757 = local read "work buffer"() -> (w970:string)
                          n758 = Match Pattern(string=w970, regular expression=w976) -> (match substring=w973:string, after substring=w980:string)  [unwired: 1 in, 2 out]
                          n759 = Equal?(x=w976, y=w973) -> (x = y?=w984:bool)
                          n760 = Match Pattern(string=w980, regular expression=",") -> (before substring=w972:string)  [unwired: 1 in, 3 out]
                          n761 = Search and Replace String(input string=w972, search string="0x") -> (result string=w974:string)  [unwired: 6 in, 3 out]
                          n762 = Concatenate Strings(w973, w972, "," ("string")) -> (w969:string)
                          n763 = Scan Value(string=w974, format string="%x", default (0 dbl)=w982) -> (value=w987:dbl)  [unwired: 1 out]
                          n764 = Search and Replace String(input string=w970, search string=w969) -> (result string=w968:string)  [unwired: 6 in, 3 out]
                          n765 = local read "MCU Data"() -> (w985:dbl[])
                          n766 = local write "work buffer"(w968) -> ()
                          n767 = Not Equal?(x=w987, y=w982) -> (x != y?=w983:bool)
                          n768 = And(x=w984, y=w983) -> (x .and. y?=w988:bool)
                          n769 = Build Array (concatenate)(w985, w987) -> (w986:dbl[])
                          n770 = Not(x=w988) -> (.not. x?=w989:bool)
                          n771 = local write "MCU Data"(w986) -> ()
                          n772 = Or(x=w989, y=w978) -> (x .or. y?=w977:bool)
                        }
                        frame "True", Default {
                          w1000 = -99999.999 ("default (0 dbl)")
                          # "Extract value after ID and\nbefore comma"
                          # "Verify ID"
                          n773 = local read "work buffer"() -> (w992:string)
                          n774 = Match Pattern(string=w992, regular expression=w996) -> (match substring=w994:string, after substring=w998:string)  [unwired: 1 in, 2 out]
                          n775 = Equal?(x=w996, y=w994) -> (x = y?=w1002:bool)
                          n776 = Match Pattern(string=w998, regular expression=",") -> (before substring=w993:string)  [unwired: 1 in, 3 out]
                          n777 = local read "MCU Data"() -> (w1003:dbl[])
                          n778 = Concatenate Strings(w994, w993, "," ("string")) -> (w991:string)
                          n779 = Scan Value(string=w993, format string="%9.6f", default (0 dbl)=w1000) -> (value=w1005:dbl)  [unwired: 1 out]
                          n780 = Search and Replace String(input string=w992, search string=w991) -> (result string=w990:string)  [unwired: 6 in, 3 out]
                          n781 = Not Equal?(x=w1005, y=w1000) -> (x != y?=w1001:bool)
                          n782 = Build Array (concatenate)(w1003, w1005) -> (w1004:dbl[])
                          n783 = local write "work buffer"(w990) -> ()
                          n784 = And(x=w1002, y=w1001) -> (x .and. y?=w1006:bool)
                          n785 = local write "MCU Data"(w1004) -> ()
                          n786 = Not(x=w1006) -> (.not. x?=w1007:bool)
                          n787 = Or(x=w1007, y=w1009) -> (x .or. y?=w1008:bool)
                        }
                      }
                    }
                    n788 = local write "Data Error"(w963) -> ()
                  }
                  frame 1 {
                    w1010 = 0 items=["635nm (Red OldNMLredFW)", "Red-780-850nm (IR NewNML FW)", "Mix NML FW"] ("Color")
                    # "NML_WL in Test\n0=T=NML board Red only\n1=F=NML board near IR"
                    # "IR"
                    # "Red"
                    # "NML"
                    n789 = local read "WL: NML Only"() -> (w1011:i32)
                    n790 = local read "FW Prm"() -> (w1017:string[])
                    n791 = Array Size(array=w1017) -> (size(s)=w1014:i32)
                    n792 = Subtract(x=w1014, y=4) -> (x-y=w1012:i32)
                    n793 = Equal?(x=w1011, y=w1010) -> (x = y?=w1016:bool)
                    n794 = Select(t=w1014, s=w1016, f=w1012) -> (s? t:f=w1015:i32)
                    n795 = for {
                      N: w1015 -> [_]
                      tunnel: w1017 -> [w1020] mode=indexing
                      shift-right: [w1021] -> w1019
                      shift-left: FALSE ("Data Err") -> [w1022]
                      n796 = case shown="\"FW Version:\"" w1020 {
                        tunnel: w1022 -> [w1033 w1056 w1086 w1115]
                        tunnel: [w1032 w1055 w1085 w1114] -> w1021
                        tunnel: w1020 -> [w1023 w1049 w1084 w1096]
                        frame "True", Default {
                          w1041 = -99999.999 ("default (0 dbl)")
                          # "Other MCU parameters"
                          n797 = local read "work buffer"() -> (w1026:string)
                          n798 = Match Pattern(string=w1026, regular expression=w1023) -> (match substring=w1024:string, after substring=w1030:string)  [unwired: 1 in, 2 out]
                          n799 = Match Pattern(string=w1030, regular expression="\r\n") -> (before substring=w1028:string)  [unwired: 1 in, 3 out]
                          n800 = Equal?(x=w1024, y=w1023) -> (x = y?=w1039:bool)
                          n801 = Concatenate Strings(w1024, w1028, "\r\n") -> (w1027:string)
                          n802 = Scan Value(string=w1028, format string="%9.6f", default (0 dbl)=w1041) -> (value=w1036:dbl)  [unwired: 1 out]
                          n803 = Search and Replace String(input string=w1026, search string=w1027) -> (result string=w1025:string)  [unwired: 6 in, 3 out]
                          n804 = Not Equal?(x=w1036, y=w1041) -> (x != y?=w1040:bool)
                          n805 = And(x=w1039, y=w1040) -> (x .and. y?=w1035:bool)
                          n806 = local write "work buffer"(w1025) -> ()
                          n807 = local read "MCU Data"() -> (w1038:dbl[])
                          n808 = Not(x=w1035) -> (.not. x?=w1034:bool)
                          n809 = Or(x=w1034, y=w1033) -> (x .or. y?=w1032:bool)
                          n810 = Build Array (concatenate)(w1038, w1036) -> (w1037:dbl[])
                          n811 = local write "MCU Data"(w1037) -> ()
                        }
                        frame "FW Version:" {
                          w1043 = "\r\n"
                          w1064 = -99999.999 ("default (0 dbl)")
                          # "FW version"
                          n812 = local read "work buffer"() -> (w1051:string)
                          n813 = Match Pattern(string=w1051, regular expression=w1049) -> (match substring=w1047:string, after substring=w1046:string)  [unwired: 1 in, 2 out]
                          n814 = Match Pattern(string=w1046, regular expression="\r\n") -> (before substring=w1053:string)  [unwired: 1 in, 3 out]
                          n815 = Equal?(x=w1047, y=w1049) -> (x = y?=w1062:bool)
                          n816 = Match Pattern(string=w1046, regular expression="x") -> (after substring=w1045:string)  [unwired: 1 in, 3 out]
                          n817 = Concatenate Strings(w1047, w1053, w1043) -> (w1052:string)
                          n818 = Match Pattern(string=w1045, regular expression=w1043) -> (before substring=w1044:string)  [unwired: 1 in, 3 out]
                          n819 = Search and Replace String(input string=w1051, search string=w1052) -> (result string=w1050:string)  [unwired: 6 in, 3 out]
                          n820 = local read "MCU Data"() -> (w1061:dbl[])
                          n821 = local write "work buffer"(w1050) -> ()
                          n822 = Scan Value(string=w1044, format string="%9.6f", default (0 dbl)=w1064) -> (value=w1059:dbl)  [unwired: 1 out]
                          n823 = Not Equal?(x=w1059, y=w1064) -> (x != y?=w1063:bool)
                          n824 = And(x=w1062, y=w1063) -> (x .and. y?=w1058:bool)
                          n825 = Build Array (concatenate)(w1061, w1059) -> (w1060:dbl[])
                          n826 = Not(x=w1058) -> (.not. x?=w1057:bool)
                          n827 = Or(x=w1057, y=w1056) -> (x .or. y?=w1055:bool)
                          n828 = local write "MCU Data"(w1060) -> ()
                        }
                        frame "I_TEC (A):" {
                          w1093 = -99999.999 ("default (0 dbl)")
                          # "Infared iTEC"
                          n829 = local read "work buffer"() -> (w1069:string)
                          n830 = Match Pattern(string=w1069, regular expression=w1084) -> (match substring=w1067:string, after substring=w1066:string)  [unwired: 1 in, 2 out]
                          n831 = Equal?(x=w1084, y=w1067) -> (x = y?=w1091:bool)
                          n832 = Match Pattern(string=w1066, regular expression="cooling") -> (after substring=w1079:string, offset past match=w1081:i32)  [unwired: 1 in, 2 out]
                          n833 = Match Pattern(string=w1066, regular expression="heating") -> (after substring=w1078:string, offset past match=w1080:i32)  [unwired: 1 in, 2 out]
                          n834 = Greater?(x=w1081, y=w1080) -> (0:w1077:bool)
                          n835 = Select(t=w1079, s=w1077, f=w1078) -> (s? t:f=w1068:string)
                          n836 = Concatenate Strings(w1067, w1066, "\r\n") -> (w1072:string)
                          n837 = Search and Replace String(input string=w1069, search string=w1072) -> (result string=w1071:string)  [unwired: 6 in, 3 out]
                          n838 = Scan Value(string=w1068, format string="%9.6f", default (0 dbl)=w1093) -> (value=w1074:dbl)  [unwired: 1 out]
                          n839 = Multiply(x=w1074, y=-1.0) -> (x*y=w1075:dbl)
                          n840 = Not Equal?(x=w1074, y=w1093) -> (x != y?=w1092:bool)
                          n841 = Select(t=w1074, s=w1077, f=w1075) -> (s? t:f=w1073:dbl)
                          n842 = local write "work buffer"(w1071) -> ()
                          n843 = And(x=w1091, y=w1092) -> (x .and. y?=w1088:bool)
                          n844 = local read "MCU Data"() -> (w1090:dbl[])
                          n845 = Not(x=w1088) -> (.not. x?=w1087:bool)
                          n846 = Or(x=w1087, y=w1086) -> (x .or. y?=w1085:bool)
                          n847 = Build Array (concatenate)(w1090, w1073) -> (w1089:dbl[])
                          n848 = local write "MCU Data"(w1089) -> ()
                        }
                        frame "TEC current (A):" {
                          w1122 = -99999.999 ("default (0 dbl)")
                          # "Red iTEC"
                          n849 = local read "work buffer"() -> (w1098:string)
                          n850 = Match Pattern(string=w1098, regular expression=w1096) -> (match substring=w1095:string, after substring=w1097:string)  [unwired: 1 in, 2 out]
                          n851 = Match Pattern(string=w1097, regular expression="cooling") -> (after substring=w1109:string, offset past match=w1111:i32)  [unwired: 1 in, 2 out]
                          n852 = Match Pattern(string=w1097, regular expression="heating") -> (after substring=w1108:string, offset past match=w1110:i32)  [unwired: 1 in, 2 out]
                          n853 = Equal?(x=w1095, y=w1096) -> (x = y?=w1120:bool)
                          n854 = Greater?(x=w1111, y=w1110) -> (0:w1106:bool)
                          n855 = Select(t=w1109, s=w1106, f=w1108) -> (s? t:f=w1107:string)
                          n856 = Concatenate Strings(w1095, w1097, "\r\n") -> (w1101:string)
                          n857 = Scan Value(string=w1107, format string="%9.6f", default (0 dbl)=w1122) -> (value=w1103:dbl)  [unwired: 1 out]
                          n858 = Multiply(x=w1103, y=-1.0) -> (x*y=w1104:dbl)
                          n859 = Search and Replace String(input string=w1098, search string=w1101) -> (result string=w1100:string)  [unwired: 6 in, 3 out]
                          n860 = Select(t=w1103, s=w1106, f=w1104) -> (s? t:f=w1102:dbl)
                          n861 = local write "work buffer"(w1100) -> ()
                          n862 = local read "MCU Data"() -> (w1119:dbl[])
                          n863 = Not Equal?(x=w1103, y=w1122) -> (x != y?=w1121:bool)
                          n864 = And(x=w1120, y=w1121) -> (x .and. y?=w1117:bool)
                          n865 = Not(x=w1117) -> (.not. x?=w1116:bool)
                          n866 = Build Array (concatenate)(w1119, w1102) -> (w1118:dbl[])
                          n867 = Or(x=w1116, y=w1115) -> (x .or. y?=w1114:bool)
                          n868 = local write "MCU Data"(w1118) -> ()
                        }
                      }
                    }
                    n869 = local write "Data Error"(w1019) -> ()
                  }
                }
              }
              frame #4 {
                # "Mode"
                n870 = local read "FW inTest"() -> (w1124:u16)
                n871 = case shown="1" w1124 {
                  frame 0, Default {
                    # "WSD.  No Mode No actions"
                  }
                  frame 1 {
                    # "NML_WL in Test\n0=T=NML board Red only\n1=F=NML board near IR"
                    # "NML"
                    n872 = local read "WL: NML Only"() -> (w1125:i32)
                    n873 = case shown="1" w1125 {
                      frame 0, Default {
                        # "Old NML Red only.  No actions"
                      }
                      frame 1 {
                        w1133 = "Error" ("regular expression")
                        w1134 = "Shutter Error" ("regular expression")
                        w1137 = "Warning" ("regular expression")
                        w1138 = "Normal" ("regular expression")
                        n874 = local read "work buffer"() -> (w1131:string)
                        n875 = Match Pattern(string=w1131, regular expression=w1134) -> (match substring=w1135:string)  [unwired: 1 in, 3 out]
                        n876 = Match Pattern(string=w1131, regular expression=w1137) -> (match substring=w1136:string)  [unwired: 1 in, 3 out]
                        n877 = Match Pattern(string=w1131, regular expression=w1133) -> (match substring=w1132:string)  [unwired: 1 in, 3 out]
                        n878 = Match Pattern(string=w1131, regular expression=w1138) -> (match substring=w1141:string)  [unwired: 1 in, 3 out]
                        n879 = Equal?(x=w1134, y=w1135) -> (x = y?=w1127:bool)
                        n880 = Equal?(x=w1137, y=w1136) -> (x = y?=w1128:bool)
                        n881 = Equal?(x=w1133, y=w1132) -> (x = y?=w1126:bool)
                        n882 = Equal?(x=w1138, y=w1141) -> (x = y?=w1130:bool)
                        n883 = case shown="False" w1130 {
                          tunnel: [w1144 0.0] -> w1129
                          tunnel: w1128 -> [w1145 _]
                          tunnel: w1127 -> [w1143 _]
                          tunnel: w1126 -> [w1142 _]
                          frame False {
                            n884 = case shown="False" w1145 {
                              tunnel: [w1147 1.0] -> w1144
                              tunnel: w1143 -> [w1148 _]
                              tunnel: w1142 -> [w1146 _]
                              frame False {
                                n885 = case shown="True" w1148 {
                                tunnel: [w1149 3.0] -> w1147
                                tunnel: w1146 -> [w1150 _]
                                frame False {
                                n886 = case shown="False" w1150 {
                                tunnel: [-99999.999 ("default (0 dbl)") 2.0] -> w1149
                                frame False {
                                n887 = local write "Data Error"(TRUE ("Data Err")) -> ()
                                }
                                frame True {
                                }
                                }
                                }
                                frame True {
                                }
                                }
                              }
                              frame True {
                              }
                            }
                          }
                          frame True {
                          }
                        }
                        n888 = local read "MCU Data"() -> (w1140:dbl[])
                        n889 = Build Array (concatenate)(w1140, w1129) -> (w1139:dbl[])
                        n890 = local write "MCU Data"(w1139) -> ()
                      }
                    }
                  }
                }
              }
              frame #5 {
                # "WL"
                n891 = local read "FW inTest"() -> (w1157:u16)
                n892 = case shown="1" w1157 {
                  frame 0, Default {
                    # "WSD.  No Mode No actions"
                  }
                  frame 1 {
                    # "NML_WL in Test\n0=T=NML board Red only\n1=F=NML board near IR"
                    # "NML"
                    n893 = local read "WL: NML Only"() -> (w1158:i32)
                    n894 = case shown="1" w1158 {
                      frame 0, Default {
                        # "Old NML Red only.  No actions"
                      }
                      frame 1 {
                        w1166 = "850" ("regular expression")
                        w1167 = "780" ("regular expression")
                        w1170 = "Red" ("regular expression")
                        w1171 = "None" ("regular expression")
                        # "NML IR"
                        n895 = local read "work buffer"() -> (w1164:string)
                        n896 = Match Pattern(string=w1164, regular expression=w1167) -> (match substring=w1168:string)  [unwired: 1 in, 3 out]
                        n897 = Match Pattern(string=w1164, regular expression=w1170) -> (match substring=w1169:string)  [unwired: 1 in, 3 out]
                        n898 = Match Pattern(string=w1164, regular expression=w1166) -> (match substring=w1165:string)  [unwired: 1 in, 3 out]
                        n899 = Match Pattern(string=w1164, regular expression=w1171) -> (match substring=w1174:string)  [unwired: 1 in, 3 out]
                        n900 = Equal?(x=w1167, y=w1168) -> (x = y?=w1160:bool)
                        n901 = Equal?(x=w1170, y=w1169) -> (x = y?=w1161:bool)
                        n902 = Equal?(x=w1166, y=w1165) -> (x = y?=w1159:bool)
                        n903 = Equal?(x=w1171, y=w1174) -> (x = y?=w1163:bool)
                        n904 = case shown="False" w1163 {
                          tunnel: [w1177 0.0] -> w1162
                          tunnel: w1161 -> [w1178 _]
                          tunnel: w1160 -> [w1176 _]
                          tunnel: w1159 -> [w1175 _]
                          frame False {
                            n905 = case shown="False" w1178 {
                              tunnel: [w1180 1.0] -> w1177
                              tunnel: w1176 -> [w1181 _]
                              tunnel: w1175 -> [w1179 _]
                              frame False {
                                n906 = case shown="False" w1181 {
                                tunnel: [w1182 2.0] -> w1180
                                tunnel: w1179 -> [w1183 _]
                                frame False {
                                n907 = case shown="True" w1183 {
                                tunnel: [-99999.999 ("default (0 dbl)") 3.0] -> w1182
                                frame False {
                                n908 = local write "Data Error"(TRUE ("Data Err")) -> ()
                                }
                                frame True {
                                }
                                }
                                }
                                frame True {
                                }
                                }
                              }
                              frame True {
                              }
                            }
                          }
                          frame True {
                          }
                        }
                        n909 = local read "MCU Data"() -> (w1173:dbl[])
                        n910 = Build Array (concatenate)(w1173, w1162) -> (w1172:dbl[])
                        n911 = local write "MCU Data"(w1172) -> ()
                      }
                    }
                  }
                }
              }
              frame #6 {
                # "LHM Calibration Gain and Offset"
                n912 = local read "FW inTest"() -> (w1190:u16)
                n913 = case shown="1" w1190 {
                  frame 0, Default {
                    # "WSD.  No Mode No actions"
                  }
                  frame 1 {
                    # "NML_WL in Test\n0=T=NML board Red only\n1=F=NML board near IR"
                    # "NML"
                    n914 = local read "WL: NML Only"() -> (w1191:i32)
                    n915 = case shown="1" w1191 {
                      frame 0, Default {
                        # "Old NML Red only.  No actions"
                      }
                      frame 1 {
                        w1192 = "LHM Calibration:" ("regular expression")
                        w1200 = -99999.999 ("default (0 dbl)")
                        # "NML IR"
                        n916 = local read "work buffer"() -> (w1207:string)
                        n917 = Match Pattern(string=w1207, regular expression=w1192) -> (match substring=w1193:string, after substring=w1208:string)  [unwired: 1 in, 2 out]
                        n918 = Equal?(x=w1193, y=w1192) -> (x = y?=w1214:bool)
                        n919 = Match Pattern(string=w1208, regular expression="Gain=") -> (after substring=w1203:string)  [unwired: 1 in, 3 out]
                        n920 = Match Pattern(string=w1208, regular expression="Offset=") -> (after substring=w1204:string)  [unwired: 1 in, 3 out]
                        n921 = Match Pattern(string=w1203, regular expression=",") -> (before substring=w1202:string)  [unwired: 1 in, 3 out]
                        n922 = Concatenate Strings(w1193, w1208, "\r\n") -> (w1210:string)
                        n923 = Search and Replace String(input string=w1207, search string=w1210) -> (result string=w1209:string)  [unwired: 6 in, 3 out]
                        n924 = Scan Value(string=w1202, format string="%9.6f", default (0 dbl)=w1200) -> (value=w1217:dbl)  [unwired: 1 out]
                        n925 = Scan Value(string=w1204, format string="%9.6f", default (0 dbl)=w1200) -> (value=w1218:dbl)  [unwired: 1 out]
                        n926 = Not Equal?(x=w1218, y=w1200) -> (x != y?=w1206:bool)
                        n927 = local write "work buffer"(w1209) -> ()
                        n928 = Not Equal?(x=w1217, y=w1200) -> (x != y?=w1215:bool)
                        n929 = local read "MCU Data"() -> (w1213:dbl[])
                        n930 = Compound Arithmetic op=AND(w1214, w1215, w1206) -> (w1205:bool)
                        n931 = Not(x=w1205) -> (.not. x?=w1211:bool)
                        n932 = Build Array (concatenate)(w1213, w1217, w1218) -> (w1212:dbl[])
                        n933 = Or(x=w1211, y=FALSE ("Data Err")) -> (x .or. y?=w1216:bool)
                        n934 = local write "Data Error"(w1216) -> ()
                        n935 = local write "MCU Data"(w1212) -> ()
                      }
                    }
                  }
                }
              }
              frame #7 {
                # "Log error if timeout or data error occurs."
                n936 = local read "Serial"() -> (w1229:string[])
                n937 = local read "Display UUT #"() -> (w1228:i32)
                n938 = local read "Timeout"() -> (w1234:bool)
                n939 = local read "Data Error"() -> (w1236:bool)
                n940 = Select(t=" Data Corrupted" ("Msg"), s=w1236, f=" Data Received" ("Msg")) -> (s? t:f=w1233:string)
                n941 = Index Array(array=w1229, index=w1228) -> (element=w1227:string)
                n942 = Concatenate Strings("Unit " ("Msg"), w1227) -> (w1226:string)
                n943 = Select(t=" Not Responded" ("Msg"), s=w1234, f=w1233) -> (s? t:f=w1225:string)
                n944 = local read "Timeout"() -> (w1232:bool)
                n945 = local read "Data Error"() -> (w1231:bool)
                n946 = Concatenate Strings(w1226, w1225) -> (w1222:string)
                n947 = Concatenate Strings(w1222, "\r\n") -> (w1220:string)
                n948 = local write "Msg"(w1222) -> ()
                n949 = Or(x=w1232, y=w1231) -> (x .or. y?=w1219:bool)
                n950 = case shown="True" w1219 {
                  tunnel: w1220 -> [_ w1241]
                  frame False {
                    n951 = local read "Display UUT #"() -> (w1240:i32)
                    n952 = local read "Module Error"() -> (w1239:bool[])
                    n953 = Replace Array Subset(array=w1239, new element=FALSE ("new element/subarray"), index=w1240) -> (w1237:bool[])
                    n954 = local write "Module Error"(w1237) -> ()
                  }
                  frame True {
                    w1242 = "\t"
                    w1247 = "" ("replace string (\"\")")
                    w1248 = "\r\n"
                    n955 = local read "Module Error"() -> (w1253:bool[])
                    n956 = local read "Display UUT #"() -> (w1254:i32)
                    n957 = Get Date/Time In Seconds() -> (seconds since 1Jan1904=w1260:timestamp)
                    n958 = Format Date/Time String(time format string (%c)="%m/%d/%y", seconds (now)=w1260) -> (date/time string=w1250:string)  [unwired: 1 in]
                    n959 = Format Date/Time String(time format string (%c)="%H:%M:%S", seconds (now)=w1260) -> (date/time string=w1249:string)  [unwired: 1 in]
                    n960 = Replace Array Subset(array=w1253, new element=TRUE ("new element/subarray"), index=w1254) -> (w1251:bool[])
                    n961 = local read "System Messages"() -> (w1264:string)
                    n962 = Search and Replace String(input string=w1250, search string=w1248, replace string=w1247) -> (result string=w1244:string)  [unwired: 5 in, 3 out]
                    n963 = Search and Replace String(input string=w1249, search string=w1248, replace string=w1247) -> (result string=w1243:string)  [unwired: 5 in, 3 out]
                    n964 = local write "Module Error"(w1251) -> ()
                    n965 = Build Array(w1244, w1242, w1243, w1242, w1241) -> (w1245:string[])
                    n966 = local read "Log File"() -> (w1259:path)
                    n967 = Concatenate Strings(w1264, w1245) -> (w1263:string)
                    n968 = local write "System Messages"(w1263) -> ()
                    n969 = call-poly <vilib>:"Write Delimited Spreadsheet.vi"("file path (dialog if empty)"=w1259, "1D data"=w1245, "append to file? (new file:F)"=TRUE ("transpose? (no:F)"), "transpose? (no:F)"=TRUE ("append to file? (new file:F)"), "delimiter (\\t)"="," ("delimiter (\\t)")) -> ("new file path (Not A Path if cancelled)"=w1255:path)  [unwired: 9 in, 1 out]
                    n970 = local write "Log File"(w1255) -> ()
                    n971 = Wait Until Next ms Multiple(millisecond multiple=u32 300) -> ()  [unwired: 1 out]
                  }
                }
              }
              frame #8 {
                n972 = local write "Msg"("Reading optical power from 2936R meter" ("Msg")) -> ()
              }
              frame #9 {
                # "Channel Select"
                # "Ch2"
                # "Ch1"
                # "Read PM"
                n973 = disable-structure shown="Enabled" {
                  frame Disabled {
                    # "Disabled on 03-10-17:\nRead from power meter via rs232"
                    n974 = local read "Display UUT #"() -> (w1299:i32)
                    n975 = Less?(x=w1299, y=u16 2) -> (x < y?=w1309:bool)
                    n976 = Equal?(x=w1299, y=u16 0) -> (x = y?=w1302:bool)
                    n977 = Equal?(x=w1299, y=u16 2) -> (x = y?=w1301:bool)
                    n978 = local read "COMs"() -> (w1311:refnum<visa-resource-name>[])
                    n979 = Or(x=w1302, y=w1301) -> (x .or. y?=w1300:bool)
                    n980 = Select(t=u16 4 ("y"), s=w1309, f=u16 5 ("y")) -> (s? t:f=w1306:u16)
                    n981 = Concatenate Strings("PM:PWS?" ("Command 2"), "\r") -> (w1296:string)
                    n982 = Index Array(array=w1311, index=w1306) -> (element=w1305:refnum<visa-resource-name>)
                    n983 = local read "error"() -> (w1320:errorcluster)
                    n984 = call "Com_Cmd_RevA.vi"("Timeout"=1000, "Query"=TRUE ("Query 2"), "error in"=w1320, "Delay, ms"=u32 10, "write buffer"=w1296, "VISA"=w1305) -> ("error out"=w1321:errorcluster, "read buffer"=w1289:string, "Timeout"=w1323:bool, "return count"=w1322:u32)  [unwired: 2 out]
                    n985 = Search and Replace String(input string=w1289, search string=w1296) -> (result string=w1295:string, offset past replacement=w1294:i32)  [unwired: 6 in, 2 out]
                    n986 = Increment(x=w1294) -> (x+1=w1293:i32)
                    n987 = local write "Timeout"(w1323) -> ()
                    n988 = local write "read buffer"(w1289) -> ()
                    n989 = local write "Bytes Rcvd"(w1322) -> ()
                    n990 = local write "error"(w1321) -> ()
                    n991 = String Subset(string=w1295, offset (0)=w1293) -> (substring=w1298:string)  [unwired: 1 in]
                    n992 = Match Pattern(string=w1298, regular expression="\\s") -> (after substring=w1316:string)  [unwired: 1 in, 3 out]
                    n993 = Match Pattern(string=w1316, regular expression="\\s") -> (after substring=w1314:string)  [unwired: 1 in, 3 out]
                    n994 = local read "System Data"() -> (w1327:dbl[])
                    n995 = Fract/Exp String To Number(string=w1298, offset=0) -> (number=w1313:dbl)  [unwired: 2 in, 1 out]
                    n996 = Fract/Exp String To Number(string=w1314, offset=0) -> (number=w1312:dbl)  [unwired: 2 in, 1 out]
                    n997 = Select(t=w1313, s=w1300, f=w1312) -> (s? t:f=w1292:dbl)
                    n998 = Build Array (concatenate)(w1327, w1292) -> (w1326:dbl[])
                    n999 = local write "System Data"(w1326) -> ()
                  }
                  frame Enabled {
                  }
                }
                n1000 = local read "Display UUT #"() -> (w1268:i32)
                n1001 = local read "reference Out"() -> (w1286:refnum<k24>)
                n1002 = Quotient & Remainder(x=w1268, y=2) -> (x-y*floor(x/y)=w1273:i32, floor(x/y)=w1266:i32)
                n1003 = local read "error"() -> (w1287:errorcluster)
                n1004 = Increment(x=w1266) -> (x+1=w1267:i32)
                n1005 = call "NewPort_PM_USB_Read-Set.vi"("reference"=w1286, "USB Address"=w1267, "Read Power(F)\nSet Lambda(T)"=FALSE ("Read Power(T)\nSet Lambda(F)"), "error in"=w1287, "Read Power\nSingle CH(F)\nDual CHs(T)"=TRUE ("Set Lambda\nSingle CH(F)\nDual CHs(T)")) -> ("Query-String Format\nfrom Read Buffer"=w1283:string, "error out"=w1277:errorcluster)  [unwired: 9 in]
                n1006 = Number To Boolean Array(number=w1273) -> (Boolean array=w1272:bool[])
                n1007 = local write "error"(w1277) -> ()
                n1008 = Index Array(array=w1272, index=0) -> (element=w1270:bool)
                n1009 = Match Pattern(string=w1283, regular expression=",") -> (before substring=w1282:string, after substring=w1281:string)  [unwired: 1 in, 2 out]
                n1010 = Not(x=w1270) -> (.not. x?=w1269:bool)
                n1011 = Fract/Exp String To Number(string=w1282) -> (number=w1276:dbl)  [unwired: 3 in, 1 out]
                n1012 = Fract/Exp String To Number(string=w1281) -> (number=w1275:dbl)  [unwired: 3 in, 1 out]
                n1013 = Select(t=w1276, s=w1269, f=w1275) -> (s? t:f=w1278:dbl)
                n1014 = local read "System Data"() -> (w1288:dbl[])
                n1015 = Build Array (concatenate)(w1288, w1278) -> (w1279:dbl[])
                n1016 = local write "System Data"(w1279) -> ()
              }
              frame #10 {
                n1017 = local write "Msg"("Reading Temperature" ("Msg")) -> ()
              }
              frame #11 {
                # "Get Temp"
                n1018 = local read "cDAQ1"() -> (w1334:string)
                n1019 = Concatenate Strings(w1334, "Mod4" ("string")) -> (w1329:string)
                n1020 = call "DAQ Assistant"("device name"=w1329) -> ("data"=w1330:dynamicdata)  [unwired: 16 in, 2 out]
                n1021 = Split Signals(w1330) -> (w1332:dynamicdata)  [unwired: 4 in, 3 out]
                n1022 = local read "System Data"() -> (w1337:dbl[])
                n1023 = call "Convert from Dynamic Data6"("Dynamic Data Type"=w1332) -> ("Array"=w1331:dbl[])  [unwired: 3 in]
                n1024 = call-poly <vilib>:"Mean.vi"("X"=w1331) -> ("mean"=w1335:dbl)  [unwired: 1 out]
                n1025 = Build Array (concatenate)(w1337, w1335) -> (w1336:dbl[])
                n1026 = local write "System Data"(w1336) -> ()
              }
              frame #12 {
                n1027 = local write "Msg"("Reading DAQ data" ("Msg")) -> ()
              }
              frame #13 {
                # "Get DAQ data"
                n1028 = local read "Display UUT #"() -> (w1339:i32)
                n1029 = case shown="3" w1339 {
                  tunnel: [w1381 w1385 w1386 w1390 w1397 w1401 w1402 w1406] -> w1357
                  frame 0, Default {
                    n1030 = local read "cDAQ1"() -> (w1380:string)
                    n1031 = Concatenate Strings(w1380, "Mod3" ("string")) -> (w1378:string)
                    n1032 = call "DAQ Assistant2"("device name"=w1378) -> ("data"=w1381:dynamicdata)  [unwired: 16 in, 2 out]
                  }
                  frame 1 {
                    n1033 = local read "cDAQ1"() -> (w1384:string)
                    n1034 = Concatenate Strings(w1384, "Mod3" ("string")) -> (w1382:string)
                    n1035 = call "DAQ Assistant3"("device name"=w1382) -> ("data"=w1385:dynamicdata)  [unwired: 16 in, 2 out]
                  }
                  frame 2 {
                    n1036 = local read "cDAQ1"() -> (w1389:string)
                    n1037 = Concatenate Strings(w1389, "Mod2" ("string")) -> (w1387:string)
                    n1038 = call "DAQ Assistant4"("device name"=w1387) -> ("data"=w1386:dynamicdata)  [unwired: 16 in, 2 out]
                  }
                  frame 3 {
                    n1039 = local read "cDAQ1"() -> (w1393:string)
                    n1040 = Concatenate Strings(w1393, "Mod2" ("string")) -> (w1391:string)
                    n1041 = call "DAQ Assistant6"("device name"=w1391) -> ("data"=w1390:dynamicdata)  [unwired: 16 in, 2 out]
                  }
                  frame 4 {
                    n1042 = local read "cDAQ2"() -> (w1396:string)
                    n1043 = Concatenate Strings(w1396, "Mod3" ("string")) -> (w1394:string)
                    n1044 = call "DAQ Assistant12"("device name"=w1394) -> ("data"=w1397:dynamicdata)  [unwired: 16 in, 2 out]
                  }
                  frame 5 {
                    n1045 = local read "cDAQ2"() -> (w1400:string)
                    n1046 = Concatenate Strings(w1400, "Mod3" ("string")) -> (w1398:string)
                    n1047 = call "DAQ Assistant13"("device name"=w1398) -> ("data"=w1401:dynamicdata)  [unwired: 16 in, 2 out]
                  }
                  frame 6 {
                    n1048 = local read "cDAQ2"() -> (w1405:string)
                    n1049 = Concatenate Strings(w1405, "Mod2" ("string")) -> (w1403:string)
                    n1050 = call "DAQ Assistant14"("device name"=w1403) -> ("data"=w1402:dynamicdata)  [unwired: 16 in, 2 out]
                  }
                  frame 7 {
                    n1051 = local read "cDAQ2"() -> (w1409:string)
                    n1052 = Concatenate Strings(w1409, "Mod2" ("string")) -> (w1407:string)
                    n1053 = call "DAQ Assistant15"("device name"=w1407) -> ("data"=w1406:dynamicdata)  [unwired: 16 in, 2 out]
                  }
                }
                n1054 = Split Signals(w1357) -> (w1359:dynamicdata, w1361:dynamicdata, w1362:dynamicdata, w1363:dynamicdata, w1352:dynamicdata, w1349:dynamicdata, w1350:dynamicdata, w1351:dynamicdata)  [unwired: 8 in]
                n1055 = call "Convert from Dynamic Data2"("Dynamic Data Type"=w1359) -> ("Array"=w1360:dbl[])  [unwired: 3 in]
                n1056 = call "Convert from Dynamic Data3"("Dynamic Data Type"=w1361) -> ("Array"=w1364:dbl[])  [unwired: 3 in]
                n1057 = call "Convert from Dynamic Data4"("Dynamic Data Type"=w1362) -> ("Array"=w1365:dbl[])  [unwired: 3 in]
                n1058 = call "Convert from Dynamic Data5"("Dynamic Data Type"=w1363) -> ("Array"=w1366:dbl[])  [unwired: 3 in]
                n1059 = call "Convert from Dynamic Data10"("Dynamic Data Type"=w1352) -> ("Array"=w1356:dbl[])  [unwired: 3 in]
                n1060 = call "Convert from Dynamic Data11"("Dynamic Data Type"=w1349) -> ("Array"=w1355:dbl[])  [unwired: 3 in]
                n1061 = call "Convert from Dynamic Data12"("Dynamic Data Type"=w1350) -> ("Array"=w1354:dbl[])  [unwired: 3 in]
                n1062 = call "Convert from Dynamic Data13"("Dynamic Data Type"=w1351) -> ("Array"=w1353:dbl[])  [unwired: 3 in]
                n1063 = call-poly <vilib>:"Mean.vi"("X"=w1360) -> ("mean"=w1375:dbl)  [unwired: 1 out]
                n1064 = call-poly <vilib>:"Mean.vi"("X"=w1364) -> ("mean"=w1340:dbl)  [unwired: 1 out]
                n1065 = call-poly <vilib>:"Mean.vi"("X"=w1365) -> ("mean"=w1373:dbl)  [unwired: 1 out]
                n1066 = call-poly <vilib>:"Mean.vi"("X"=w1366) -> ("mean"=w1341:dbl)  [unwired: 1 out]
                n1067 = call-poly <vilib>:"Mean.vi"("X"=w1356) -> ("mean"=w1371:dbl)  [unwired: 1 out]
                n1068 = call-poly <vilib>:"Mean.vi"("X"=w1355) -> ("mean"=w1342:dbl)  [unwired: 1 out]
                n1069 = call-poly <vilib>:"Mean.vi"("X"=w1354) -> ("mean"=w1343:dbl)  [unwired: 1 out]
                n1070 = call-poly <vilib>:"Mean.vi"("X"=w1353) -> ("mean"=w1344:dbl)  [unwired: 1 out]
                n1071 = Multiply(x=w1340, y=0.25 ("mean")) -> (x*y=w1374:dbl)
                n1072 = Multiply(x=w1341, y=0.25 ("mean")) -> (x*y=w1372:dbl)
                n1073 = Multiply(x=w1342, y=0.25 ("mean")) -> (x*y=w1370:dbl)
                n1074 = Multiply(x=w1343, y=4.922 ("mean")) -> (x*y=w1369:dbl)
                n1075 = Multiply(x=w1344, y=0.25 ("mean")) -> (x*y=w1368:dbl)
                n1076 = Build Array(w1375, w1374, w1373, w1372, w1371, w1370, w1369, w1368) -> (w1367:dbl[])
                n1077 = local read "System Data"() -> (w1377:dbl[])
                n1078 = Build Array (concatenate)(w1377, w1367) -> (w1376:dbl[])
                n1079 = local write "System Data"(w1376) -> ()
              }
              frame #14 {
                # "03-10-17, added"
                # "Time to control\nshutter yet?\n(control from \nlong open to \nshort close)"
                n1080 = local read "Tpass Shtr Open"() -> (w1411:bool)
                n1081 = local read "Data Time"() -> (w1410:timestamp)
                n1082 = case shown="True" w1411 {
                  tunnel: w1410 -> [_ w1415]
                  frame False {
                    # "If required time duration for open shutter not met, use zero value as place holder for closed shutter power reading."
                    n1083 = local read "System Data"() -> (w1412:dbl[])
                    n1084 = Build Array (concatenate)(w1412, 0.0 ("element")) -> (w1414:dbl[])
                    n1085 = local write "System Data"(w1414) -> ()
                  }
                  frame True {
                    n1086 = stacked-sequence {
                      tunnel: w1415 -> [_ _ _ _ w1528]
                      frame #0 {
                        w1416 = 4 ("y")
                        w1420 = FALSE
                        # "F=open, T=closed"
                        # "Close shutter individually with respect to the particular unit under test"
                        n1087 = local read "Display UUT #"() -> (w1417:i32)
                        n1088 = Build Array(w1420, w1420, w1420, w1420) -> (w1419:bool[])
                        n1089 = Greater Or Equal?(x=w1417, y=w1416) -> (x >= y?=w1418:bool)
                        n1090 = case shown="False" w1418 {
                          tunnel: w1417 -> [w1424 w1431]
                          tunnel: w1419 -> [w1426 w1433]
                          tunnel: w1416 -> [w1423 _]
                          frame True {
                            n1091 = Subtract(x=w1424, y=w1423) -> (x-y=w1422:i32)
                            n1092 = Replace Array Subset(array=w1426, new element=TRUE, index=w1422) -> (w1425:bool[])
                            n1093 = local read "cDAQ2"() -> (w1428:string)
                            n1094 = Concatenate Strings(w1428, "Mod1" ("string")) -> (w1430:string)
                            n1095 = call "DAQ Assistant8"("data"=w1425, "device name"=w1430) -> ()  [unwired: 16 in, 2 out]
                          }
                          frame False {
                            n1096 = Replace Array Subset(array=w1433, new element=TRUE, index=w1431) -> (w1432:bool[])
                            n1097 = local read "cDAQ1"() -> (w1435:string)
                            n1098 = Concatenate Strings(w1435, "Mod1" ("string")) -> (w1437:string)
                            n1099 = call "DAQ Assistant17"("data"=w1432, "device name"=w1437) -> ()  [unwired: 16 in, 2 out]
                          }
                        }
                        n1100 = local write "Msg"("Shutter closed for selected unit." ("Msg")) -> ()
                      }
                      frame #1 {
                        # "Indicator"
                        # "Indicator"
                        # "Indicator"
                        # "5-18-17, revised and added control and indicators"
                        # "Close shutter for 6 seconds"
                        n1101 = local read "Shtr Ctrl Close, Seconds"() -> (w1438:dbl)
                        n1102 = To Unsigned Long Integer(number=w1438) -> (unsigned 32bit integer=w1439:u32)
                        n1103 = Multiply(x=w1439, y=u32 1000 ("milliseconds to wait")) -> (x*y=w1444:u32)
                        n1104 = Wait (ms)(milliseconds to wait=w1444) -> ()  [unwired: 1 out]
                        n1105 = local write "Tpass Shtr Close"(FALSE ("Pass SttrClose")) -> ()
                        n1106 = local write "Shtr Close"(TRUE ("Sttrs Close")) -> ()
                        n1107 = local write "Shtr Open"(FALSE ("Sttrs Open")) -> ()
                      }
                      frame #2 {
                        # "Channel Select"
                        # "Ch2"
                        # "Ch1"
                        # "03-16-17:  \nRevised NP-PM USB READ/SET subVI"
                        # "USB-read power meter\nat shutter closed"
                        n1108 = local read "Display UUT #"() -> (w1454:i32)
                        n1109 = disable-structure shown="Enabled" {
                          frame Disabled {
                            # "Disabled on 03-10-17:\nRead from power meter via rs232 option"
                            n1110 = local read "Display UUT #"() -> (w1478:i32)
                            n1111 = Less?(x=w1478, y=2) -> (x < y?=w1488:bool)
                            n1112 = Equal?(x=w1478, y=0) -> (x = y?=w1481:bool)
                            n1113 = Equal?(x=w1478, y=2) -> (x = y?=w1480:bool)
                            n1114 = local read "COMs"() -> (w1490:refnum<visa-resource-name>[])
                            n1115 = Or(x=w1481, y=w1480) -> (x .or. y?=w1479:bool)
                            n1116 = Select(t=u16 4 ("y"), s=w1488, f=u16 5 ("y")) -> (s? t:f=w1485:u16)
                            n1117 = Concatenate Strings("PM:PWS?" ("Command 2"), "\r") -> (w1475:string)
                            n1118 = Index Array(array=w1490, index=w1485) -> (element=w1484:refnum<visa-resource-name>)
                            n1119 = local read "error"() -> (w1499:errorcluster)
                            n1120 = call "Com_Cmd_RevA.vi"("Timeout"=1000, "Query"=TRUE ("Query 2"), "error in"=w1499, "Delay, ms"=u32 10, "write buffer"=w1475, "VISA"=w1484) -> ("error out"=w1500:errorcluster, "read buffer"=w1468:string, "Timeout"=w1502:bool, "return count"=w1501:u32)  [unwired: 2 out]
                            n1121 = Search and Replace String(input string=w1468, search string=w1475) -> (result string=w1474:string, offset past replacement=w1473:i32)  [unwired: 6 in, 2 out]
                            n1122 = Increment(x=w1473) -> (x+1=w1472:i32)
                            n1123 = local write "Timeout"(w1502) -> ()
                            n1124 = local write "read buffer"(w1468) -> ()
                            n1125 = local write "Bytes Rcvd"(w1501) -> ()
                            n1126 = local write "error"(w1500) -> ()
                            n1127 = String Subset(string=w1474, offset (0)=w1472) -> (substring=w1477:string)  [unwired: 1 in]
                            n1128 = Match Pattern(string=w1477, regular expression="\\s") -> (after substring=w1495:string)  [unwired: 1 in, 3 out]
                            n1129 = Match Pattern(string=w1495, regular expression="\\s") -> (after substring=w1493:string)  [unwired: 1 in, 3 out]
                            n1130 = local read "System Data"() -> (w1506:dbl[])
                            n1131 = Fract/Exp String To Number(string=w1477, offset=0) -> (number=w1492:dbl)  [unwired: 2 in, 1 out]
                            n1132 = Fract/Exp String To Number(string=w1493, offset=0) -> (number=w1491:dbl)  [unwired: 2 in, 1 out]
                            n1133 = Select(t=w1492, s=w1479, f=w1491) -> (s? t:f=w1471:dbl)
                            n1134 = Build Array (concatenate)(w1506, w1471) -> (w1505:dbl[])
                            n1135 = local write "System Data"(w1505) -> ()
                          }
                          frame Enabled {
                          }
                        }
                        n1136 = local read "reference Out"() -> (w1465:refnum<k24>)
                        n1137 = Quotient & Remainder(x=w1454, y=2) -> (x-y*floor(x/y)=w1456:i32, floor(x/y)=w1446:i32)
                        n1138 = local read "error"() -> (w1466:errorcluster)
                        n1139 = Increment(x=w1446) -> (x+1=w1445:i32)
                        n1140 = call "NewPort_PM_USB_Read-Set.vi"("reference"=w1465, "USB Address"=w1445, "Read Power(F)\nSet Lambda(T)"=FALSE ("Read Power(T)\nSet Lambda(F)"), "error in"=w1466, "Read Power\nSingle CH(F)\nDual CHs(T)"=TRUE ("Set Lambda\nSingle CH(F)\nDual CHs(T)")) -> ("Query-String Format\nfrom Read Buffer"=w1464:string, "error out"=w1459:errorcluster)  [unwired: 9 in]
                        n1141 = Number To Boolean Array(number=w1456) -> (Boolean array=w1455:bool[])
                        n1142 = local write "error"(w1459) -> ()
                        n1143 = Index Array(array=w1455, index=0) -> (element=w1453:bool)
                        n1144 = Match Pattern(string=w1464, regular expression=",") -> (before substring=w1463:string, after substring=w1462:string)  [unwired: 1 in, 2 out]
                        n1145 = Not(x=w1453) -> (.not. x?=w1452:bool)
                        n1146 = Fract/Exp String To Number(string=w1463) -> (number=w1458:dbl)  [unwired: 3 in, 1 out]
                        n1147 = Fract/Exp String To Number(string=w1462) -> (number=w1457:dbl)  [unwired: 3 in, 1 out]
                        n1148 = Select(t=w1458, s=w1452, f=w1457) -> (s? t:f=w1460:dbl)
                        n1149 = local read "System Data"() -> (w1467:dbl[])
                        n1150 = Build Array (concatenate)(w1467, w1460) -> (w1461:dbl[])
                        n1151 = local write "System Data"(w1461) -> ()
                      }
                      frame #3 {
                        w1515 = FALSE
                        # "Indicator"
                        # "Indicator"
                        # "Indicator"
                        # "5-18-17, added indicators"
                        # "F=open, T=closed"
                        n1152 = Build Array(w1515, w1515, w1515, w1515) -> (w1510:bool[])
                        n1153 = local read "Display UUT #"() -> (w1509:i32)
                        n1154 = Greater?(x=w1509, y=4) -> (0:w1507:bool)
                        n1155 = case shown="False" w1507 {
                          tunnel: w1510 -> [w1516 w1520]
                          frame True {
                            n1156 = local read "cDAQ2"() -> (w1517:string)
                            n1157 = Concatenate Strings(w1517, "Mod1" ("string")) -> (w1519:string)
                            n1158 = call "DAQ Assistant16"("data"=w1516, "device name"=w1519) -> ()  [unwired: 16 in, 2 out]
                          }
                          frame False {
                            n1159 = local read "cDAQ1"() -> (w1521:string)
                            n1160 = Concatenate Strings(w1521, "Mod1" ("string")) -> (w1523:string)
                            n1161 = call "DAQ Assistant18"("data"=w1520, "device name"=w1523) -> ()  [unwired: 16 in, 2 out]
                          }
                        }
                        n1162 = local write "Shtr Close"(FALSE ("Sttrs Close")) -> ()
                        n1163 = local write "Shtr Open"(TRUE ("Sttrs Open")) -> ()
                        n1164 = local write "Tpass Shtr Close"(TRUE ("Pass SttrClose")) -> ()
                        n1165 = local write "Msg"("Shutter opened." ("Msg")) -> ()
                      }
                      frame #4 {
                        # "Are all systems finish shutter control?"
                        n1166 = local read "DUT Selected"() -> (w1527:i32)
                        n1167 = local read "DUT Count"() -> (w1526:i32)
                        n1168 = Decrement(x=w1526) -> (x-1=w1525:i32)
                        n1169 = Greater Or Equal?(x=w1527, y=w1525) -> (x >= y?=w1524:bool)
                        n1170 = case shown="False" w1524 {
                          tunnel: w1528 -> [_ w1530]
                          frame False {
                          }
                          frame True {
                            # "Flag"
                            # "5-18-17, moved from 12-false\nReset shutter open time control flag \nafte all systems are tested"
                            # "Update the start time of shutter open"
                            n1171 = local write "Tpass Shtr Open"(FALSE ("Pass 3 Minute")) -> ()
                            n1172 = local write "Shtr Ref Time"(w1530) -> ()
                          }
                        }
                      }
                    }
                  }
                }
              }
              frame #15 {
                # "Keeps track of # of\ndata samples for\neach UUT."
                n1173 = local read "Display UUT #"() -> (w1537:i32)
                n1174 = local read "All Results"() -> (w1534:dbl[][][])
                n1175 = local read "Points"() -> (w1536:i32[])
                n1176 = Array Size(array=w1534) -> (size(s)=w1531:i32[])
                n1177 = Index Array(array=w1536, index=w1537) -> (element=w1540:i32)
                n1178 = Increment(x=w1540) -> (x+1=w1538:i32)
                n1179 = Replace Array Subset(array=w1536, new element=w1538, index=w1537) -> (w1539:i32[])
                n1180 = local write "Points"(w1539) -> ()
                n1181 = Index Array(array=w1531, index=1) -> (element=w1533:i32)
                n1182 = Greater?(x=w1538, y=w1533) -> (0:w1535:bool)
                n1183 = case shown="False" w1535 {
                  tunnel: w1534 -> [_ w1547]
                  tunnel: w1540 -> [_ w1546]
                  frame False {
                  }
                  frame True {
                    # "Equivalent to using \"Build Array\" to expand the \"All Results\" array incrementally\nas needed when number of acquired data points exceeds previous allocation."
                    n1184 = local read "DUT Count"() -> (w1545:i32)
                    n1185 = local read "Meas N"() -> (w1541:i32)
                    n1186 = Initialize Array(0.0 ("element"), w1545, w1541) -> (w1543:dbl[][])
                    n1187 = Insert Into Array(array=w1547, index (dim 1)=w1546, new element=w1543) -> (w1542:dbl[][][])  [unwired: 2 in]
                    n1188 = local write "All Results"(w1542) -> ()
                  }
                }
              }
              frame #16 {
                # "Store newly acquired MCU and System Data to All Results Array."
                # "\"All Results\" Local Variable Indice Definition:\n0 = Unit #\n1 = Sample #\n2 = Parameter Values"
                n1189 = local read "All Results"() -> (w1554:dbl[][][])
                n1190 = local read "Points"() -> (w1555:i32[])
                n1191 = local read "Display UUT #"() -> (w1558:i32)
                n1192 = local read "Data Time"() -> (w1549:timestamp)
                n1193 = local read "MCU Data"() -> (w1551:dbl[])
                n1194 = local read "System Data"() -> (w1552:dbl[])
                n1195 = To Double Precision Float(number=w1549) -> (double precision float=w1548:dbl)
                n1196 = Index Array(array=w1555, index=w1558) -> (element=w1556:i32)
                n1197 = Build Array (concatenate)(w1548, w1551, w1552) -> (w1550:dbl[])
                n1198 = Decrement(x=w1556) -> (x-1=w1557:i32)
                n1199 = Replace Array Subset(array=w1554, new element=w1550, index (dim 0)=w1558, index (dim 1)=w1557) -> (w1553:dbl[][][])  [unwired: 1 in]
                n1200 = local write "All Results"(w1553) -> ()
              }
              frame #17 {
                # "8-23-17\nCriteria check\nfor NML or WSD"
                n1201 = disable-structure shown="Enabled" {
                  frame Disabled {
                    # "6-29-17 added, check\nif data is in range"
                    # "6-29-17 added, check\nif data is in range"
                    # "Pass: Green (F); \nFail:  Yellow (T)"
                    # "max"
                    # "min"
                    # "Pass: Green (F); \nFail:  Yellow (T)"
                    # "max"
                    # "min"
                    n1202 = local read "FW Criteria"() -> (w1568:string[][])
                    n1203 = local read "Sys Criteria"() -> (w1563:string[][])
                    n1204 = Index Array(array=w1568, index (col)=1 ("disabled index (col)")) -> (element=w1570:string[])  [unwired: 1 in]
                    n1205 = Index Array(array=w1568, index (col)=0 ("disabled index (col)")) -> (element=w1571:string[])  [unwired: 1 in]
                    n1206 = Index Array(array=w1563, index (col)=1 ("disabled index (col)")) -> (element=w1561:string[])  [unwired: 1 in]
                    n1207 = Index Array(array=w1563, index (col)=0 ("disabled index (col)")) -> (element=w1560:string[])  [unwired: 1 in]
                    n1208 = Array Size(array=w1570) -> (size(s)=w1569:i32)
                    n1209 = Array Size(array=w1561) -> (size(s)=w1562:i32)
                    n1210 = for {
                      N: w1569 -> [_]
                      tunnel: w1570 -> [w1601] mode=indexing
                      tunnel: w1571 -> [w1599] mode=indexing
                      tunnel: [w1593] -> w1572
                      i -> [w1589]
                      # "delete time"
                      # "Serves as \"Shift Register\" \nfor MCUValueTrue"
                      n1211 = local read "MCU Data"() -> (w1604:dbl[])
                      n1212 = local read "Display UUT #"() -> (w1590:i32)
                      n1213 = local read "MCUTrue"() -> (w1595:bool[][])
                      n1214 = Scan Value(string=w1601, format string="%9.6f") -> (value=w1600:dbl)  [unwired: 1 in, 1 out]
                      n1215 = Index Array(array=w1604, index=w1589) -> (element=w1603:dbl)
                      n1216 = Scan Value(string=w1599, format string="%9.6f") -> (value=w1597:dbl)  [unwired: 1 in, 1 out]
                      n1217 = Index Array(array=w1595, index (row)=w1589, index (col)=w1590) -> (element=w1596:bool)
                      n1218 = In Range and Coerce(upper limit=w1600, x=w1603, lower limit=w1597) -> (In Range?=w1591:bool)  [unwired: 1 out]
                      n1219 = And(x=w1591, y=w1596) -> (x .and. y?=w1592:bool)
                      n1220 = Replace Array Subset(array=w1595, new element=w1592, index (row)=w1589, index (col)=w1590) -> (w1594:bool[][])
                      n1221 = Not(x=w1594) -> (.not. x?=w1593:bool[][])
                      n1222 = local write "MCUTrue"(w1594) -> ()
                    }
                    n1223 = for {
                      N: w1562 -> [_]
                      tunnel: w1561 -> [w1586] mode=indexing
                      tunnel: w1560 -> [w1584] mode=indexing
                      tunnel: [w1577] -> w1559
                      i -> [w1574]
                      # "Serves as \"Shift Register\" \nfor MCUValueTrue"
                      n1224 = local read "System Data"() -> (w1576:dbl[])
                      n1225 = local read "SysTrue"() -> (w1580:bool[][])
                      n1226 = local read "Display UUT #"() -> (w1573:i32)
                      n1227 = Scan Value(string=w1586, format string="%9.6f") -> (value=w1585:dbl)  [unwired: 1 in, 1 out]
                      n1228 = Index Array(array=w1576, index=w1574) -> (element=w1588:dbl)
                      n1229 = Scan Value(string=w1584, format string="%9.6f") -> (value=w1582:dbl)  [unwired: 1 in, 1 out]
                      n1230 = Index Array(array=w1580, index (row)=w1574, index (col)=w1573) -> (element=w1581:bool)
                      n1231 = In Range and Coerce(upper limit=w1585, x=w1588, lower limit=w1582) -> (In Range?=w1575:bool)  [unwired: 1 out]
                      n1232 = And(x=w1575, y=w1581) -> (x .and. y?=w1579:bool)
                      n1233 = Replace Array Subset(array=w1580, new element=w1579, index (row)=w1574, index (col)=w1573) -> (w1578:bool[][])
                      n1234 = Not(x=w1578) -> (.not. x?=w1577:bool[][])
                      n1235 = local write "SysTrue"(w1578) -> ()
                    }
                    n1236 = local write "MCUReview"(w1572) -> ()
                    n1237 = local write "SysReview"(w1559) -> ()
                  }
                  frame Enabled {
                  }
                }
              }
              frame #18 {
                # "Question for Jie:  Why  use either \"R\" or no string characters for results of MCUCheck and SysCheck?  Why are these indicators needed in addition to the Boolean arrays?"
                # "7-7-17 Added, convert parameter review status from boolean to string"
                # "8-23-17\nContiue criteria check"
                n1238 = disable-structure shown="Enabled" {
                  frame Disabled {
                    n1239 = local read "Display UUT #"() -> (w1609:i32)
                    n1240 = local read "MCUReview"() -> (w1605:bool[][])
                    n1241 = local read "SysReview"() -> (w1608:bool[][])
                    n1242 = Index Array(array=w1608, index (col)=w1609) -> (element=w1607:bool[])  [unwired: 1 in]
                    n1243 = Index Array(array=w1605, index (col)=w1609) -> (element=w1606:bool[])  [unwired: 1 in]
                    n1244 = for {
                      tunnel: w1607 -> [w1617] mode=indexing
                      tunnel: w1609 -> [w1613]
                      i -> [w1612]
                      n1245 = Select(t="R", s=w1617, f="") -> (s? t:f=w1611:string)
                      n1246 = local read "SysCheck"() -> (w1614:string[][])
                      n1247 = Replace Array Subset(array=w1614, new element=w1611, index (row)=w1612, index (col)=w1613) -> (w1610:string[][])
                      n1248 = local write "SysCheck"(w1610) -> ()
                    }
                    n1249 = for {
                      tunnel: w1606 -> [w1618] mode=indexing
                      tunnel: w1609 -> [w1622]
                      i -> [w1621]
                      n1250 = Select(t="R", s=w1618, f="") -> (s? t:f=w1620:string)
                      n1251 = local read "MCUCheck"() -> (w1623:string[][])
                      n1252 = Replace Array Subset(array=w1623, new element=w1620, index (row)=w1621, index (col)=w1622) -> (w1619:string[][])
                      n1253 = local write "MCUCheck"(w1619) -> ()
                    }
                  }
                  frame Enabled {
                  }
                }
              }
              frame #19 {
                n1254 = local write "Msg"("Idle" ("Msg")) -> ()
                n1255 = local write "Busy"(FALSE ("Active")) -> ()
                n1256 = local write "Save"(TRUE ("Update")) -> ()
                n1257 = local write "Update Graph"(TRUE ("Update")) -> ()
                n1258 = local write "Collect"(FALSE ("Collect")) -> ()
              }
            }
          }
        }
      }
      frame #17 {
        n1259 = case shown="True" "Power" {
          frame False {
          }
          frame True {
            n1260 = stacked-sequence {
              frame #0 {
                n1261 = local write "Msg"("Reading Power from Power Meter" ("Msg")) -> ()
                n1262 = local write "Busy"(TRUE ("Active")) -> ()
              }
              frame #1 {
                # "Channel Select"
                # "Ch2"
                # "Ch1"
                n1263 = local read "Display UUT #"() -> (w1643:i32)
                n1264 = disable-structure shown="Disabled" {
                  frame Disabled {
                    # "Disabled on 03-10-17:\nRead from power meter via rs232"
                    n1265 = local read "Display UUT #"() -> (w1667:i32)
                    n1266 = Less?(x=w1667, y=2) -> (x < y?=w1677:bool)
                    n1267 = Equal?(x=w1667, y=0) -> (x = y?=w1670:bool)
                    n1268 = Equal?(x=w1667, y=2) -> (x = y?=w1669:bool)
                    n1269 = local read "COMs"() -> (w1679:refnum<visa-resource-name>[])
                    n1270 = Or(x=w1670, y=w1669) -> (x .or. y?=w1668:bool)
                    n1271 = Select(t=u16 4 ("y"), s=w1677, f=u16 5 ("y")) -> (s? t:f=w1674:u16)
                    n1272 = Concatenate Strings("PM:PWS?" ("Command 2"), "\r") -> (w1664:string)
                    n1273 = Index Array(array=w1679, index=w1674) -> (element=w1673:refnum<visa-resource-name>)
                    n1274 = local read "error"() -> (w1688:errorcluster)
                    n1275 = call "Com_Cmd_RevA.vi"("Timeout"=1000, "Query"=TRUE ("Query 2"), "error in"=w1688, "Delay, ms"=u32 10, "write buffer"=w1664, "VISA"=w1673) -> ("error out"=w1689:errorcluster, "read buffer"=w1657:string, "Timeout"=w1691:bool, "return count"=w1690:u32)  [unwired: 2 out]
                    n1276 = Search and Replace String(input string=w1657, search string=w1664) -> (result string=w1663:string, offset past replacement=w1662:i32)  [unwired: 6 in, 2 out]
                    n1277 = Increment(x=w1662) -> (x+1=w1661:i32)
                    n1278 = local write "Timeout"(w1691) -> ()
                    n1279 = local write "read buffer"(w1657) -> ()
                    n1280 = local write "Bytes Rcvd"(w1690) -> ()
                    n1281 = local write "error"(w1689) -> ()
                    n1282 = String Subset(string=w1663, offset (0)=w1661) -> (substring=w1666:string)  [unwired: 1 in]
                    n1283 = Match Pattern(string=w1666, regular expression="\\s") -> (after substring=w1684:string)  [unwired: 1 in, 3 out]
                    n1284 = Match Pattern(string=w1684, regular expression="\\s") -> (after substring=w1682:string)  [unwired: 1 in, 3 out]
                    n1285 = local read "Powertime"() -> (w1695:dbl[])
                    n1286 = Fract/Exp String To Number(string=w1666, offset=0) -> (number=w1681:dbl)  [unwired: 2 in, 1 out]
                    n1287 = Fract/Exp String To Number(string=w1682, offset=0) -> (number=w1680:dbl)  [unwired: 2 in, 1 out]
                    n1288 = Select(t=w1681, s=w1668, f=w1680) -> (s? t:f=w1660:dbl)
                    n1289 = Build Array (concatenate)(w1695, w1660) -> (w1694:dbl[])
                    n1290 = local write "Powertime"(w1694) -> ()
                  }
                  frame Enabled {
                  }
                }
                n1291 = local read "reference Out"() -> (w1654:refnum<k24>)
                n1292 = local read "error"() -> (w1655:errorcluster)
                n1293 = Quotient & Remainder(x=w1643, y=2) -> (x-y*floor(x/y)=w1645:i32, floor(x/y)=w1635:i32)
                n1294 = Increment(x=w1635) -> (x+1=w1634:i32)
                n1295 = call "NewPort_PM_USB_Read-Set.vi"("reference"=w1654, "USB Address"=w1634, "Read Power(F)\nSet Lambda(T)"=FALSE ("Read Power(T)\nSet Lambda(F)"), "error in"=w1655, "Read Power\nSingle CH(F)\nDual CHs(T)"=TRUE ("Set Lambda\nSingle CH(F)\nDual CHs(T)")) -> ("Query-String Format\nfrom Read Buffer"=w1653:string, "error out"=w1648:errorcluster)  [unwired: 9 in]
                n1296 = Number To Boolean Array(number=w1645) -> (Boolean array=w1644:bool[])
                n1297 = local write "error"(w1648) -> ()
                n1298 = Index Array(array=w1644, index=0) -> (element=w1642:bool)
                n1299 = Match Pattern(string=w1653, regular expression=",") -> (before substring=w1652:string, after substring=w1651:string)  [unwired: 1 in, 2 out]
                n1300 = Not(x=w1642) -> (.not. x?=w1641:bool)
                n1301 = Fract/Exp String To Number(string=w1652) -> (number=w1647:dbl)  [unwired: 3 in, 1 out]
                n1302 = Fract/Exp String To Number(string=w1651) -> (number=w1646:dbl)  [unwired: 3 in, 1 out]
                n1303 = Select(t=w1647, s=w1641, f=w1646) -> (s? t:f=w1649:dbl)
                n1304 = local read "System Data"() -> (w1656:dbl[])
                n1305 = Build Array (concatenate)(w1656, w1649) -> (w1650:dbl[])
                n1306 = local write "System Data"(w1650) -> ()
              }
              frame #2 {
                n1307 = local write "Busy"(FALSE ("Active")) -> ()
                n1308 = local write "Msg"("Idle" ("Msg")) -> ()
              }
            }
          }
        }
      }
      frame #18 {
        # "Save to file"
        n1309 = local read "Save"() -> (w1698:bool)
        n1310 = case shown="True" w1698 {
          frame False {
          }
          frame True {
            n1311 = stacked-sequence {
              frame #0 {
                n1312 = local write "Msg"("Saving data" ("Msg")) -> ()
              }
              frame #1 {
                # "NML"
                # "WSD"
                # "6-1-17 revised"
                n1313 = local read "Serial"() -> (w1765:string[])
                n1314 = local read "Display UUT #"() -> (w1764:i32)
                n1315 = local read "Comments"() -> (w1759:string[])
                n1316 = local read "Display UUT #"() -> (w1760:i32)
                n1317 = local read "Start Time"() -> (w1713:timestamp)
                n1318 = local read "MCU Data"() -> (w1724:dbl[])
                n1319 = Index Array(array=w1765, index=w1764) -> (element=w1745:string)
                n1320 = Index Array(array=w1759, index=w1760) -> (element=w1705:string)
                n1321 = Format Date/Time String(time format string (%c)="%m-%d-%y", seconds (now)=w1713) -> (date/time string=w1708:string)  [unwired: 1 in]
                n1322 = Format Date/Time String(time format string (%c)="%H-%M-%S", seconds (now)=w1713) -> (date/time string=w1712:string)  [unwired: 1 in]
                n1323 = local read "Data Time"() -> (w1717:timestamp)
                n1324 = local read "System Data"() -> (w1723:dbl[])
                n1325 = Equal?(x=w1705, y="") -> (x = y?=w1703:bool)
                n1326 = Index Array(array=w1724, index=0) -> (element=w1731:dbl)
                n1327 = To Double Precision Float(number=w1717) -> (double precision float=w1716:dbl)
                n1328 = Select(t="", s=w1703, f="_" ("string")) -> (s? t:f=w1700:string)
                n1329 = To Quad Integer(1:w1731) -> (0:w1732:i64)
                n1330 = Build Array (concatenate)(w1724, w1723) -> (w1729:dbl[])
                n1331 = Number To Hexadecimal String(1:i16 4 ("width (-)"), 2:w1732) -> (0:w1734:string)
                n1332 = local read "Display UUT #"() -> (w1758:i32)
                n1333 = local read "Lambda, nm"() -> (w1757:i32[])
                n1334 = Concatenate Strings(w1745, "_" ("string"), w1705, w1700) -> (w1709:string)
                n1335 = To Time Stamp(1:w1716) -> (0:w1728:timestamp)
                n1336 = Concatenate Strings("0x" ("string"), w1734) -> (w1736:string)
                n1337 = local read "780nm Folder"() -> (w1754:path)
                n1338 = local read "850nm Folder"() -> (w1753:path)
                n1339 = Concatenate Strings(w1709, w1708, "_" ("string"), w1712, ".CSV" ("string")) -> (w1710:string)
                n1340 = local read "Project Folder"() -> (w1752:path)
                n1341 = local read "635nm Folder"() -> (w1755:path)
                n1342 = Number To Exponential String(number=w1729, precision (6)=i16 6) -> (E-format string=w1741:string[])  [unwired: 2 in]
                n1343 = Format Date/Time String(time format string (%c)="%m/%d/%y", seconds (now)=w1728) -> (date/time string=w1722:string)  [unwired: 1 in]
                n1344 = Format Date/Time String(time format string (%c)="%H:%M:%S", seconds (now)=w1728) -> (date/time string=w1721:string)  [unwired: 1 in]
                n1345 = Number To Exponential String(number=w1716, precision (6)=i16 12) -> (E-format string=w1720:string)  [unwired: 2 in]
                n1346 = Number To Decimal String(number=w1757) -> (decimal integer string=w1756:string[])  [unwired: 1 in]
                n1347 = Replace Array Subset(array=w1741, new element=w1736, index=0) -> (w1740:string[])
                n1348 = local read "error"() -> (w1751:errorcluster)
                n1349 = local read "FW inTest"() -> (w1738:u16)
                n1350 = Index Array(array=w1756, index=w1758) -> (element=w1744:string)
                n1351 = call "SelectFileFolder(SubVI).vi"("635nmSubFolder"=w1755, "Project Folder in"=w1752, "Wavelength String"=w1744, "780nmSubFolder"=w1754, "850nmSubFolder"=w1753, "name or relative path"=w1710, "error in"=w1751) -> ("appended path"=w1748:path, "error out"=w1750:errorcluster)  [unwired: 7 in]
                n1352 = local read "New File"() -> (w1763:bool)
                n1353 = Equal To 0?(x=w1738) -> (x = 0?=w1739:bool)
                n1354 = call <vilib>:"Check if File or Folder Exists.vi"("error in (no error)"=w1750, "path"=w1748) -> ("error out"=w1746:errorcluster, "file or folder exists?"=w1762:bool, "dup path"=w1742:path)  [unwired: 7 in]
                n1355 = Select(t=w1740, s=w1739, f=w1741) -> (s? t:f=w1719:string[])
                n1356 = Not(x=w1763) -> (.not. x?=w1761:bool)
                n1357 = And(x=w1762, y=w1761) -> (x .and. y?=w1749:bool)
                n1358 = Build Array (concatenate)(w1722, w1721, w1720, w1719) -> (w1747:string[])
                n1359 = case shown="False" w1749 {
                  tunnel: w1742 -> [w1768 w1786]
                  tunnel: w1747 -> [w1769 w1787]
                  tunnel: w1746 -> [w1767 w1785]
                  tunnel: w1745 -> [w1770 _]
                  tunnel: w1744 -> [w1771 _]
                  tunnel: [w1766 w1784] -> w1743
                  frame False {
                    # "To write"
                    n1360 = local read "FW Prm"() -> (w1779:string[])
                    n1361 = local read "Sys Prm"() -> (w1776:string[])
                    n1362 = Build Array("Serial Number " ("time format string (%c)"), w1770) -> (w1781:string[])
                    n1363 = Build Array("Color " ("time format string (%c)"), w1771) -> (w1780:string[])
                    n1364 = Build Array (concatenate)(string[] ["Date", "Time", "Time Stamp"] ("element"), w1779, w1776) -> (w1777:string[])
                    n1365 = Build Array(w1781, w1780, w1777, w1769) -> (w1772:string[][])
                    n1366 = call-poly <vilib>:"Write Delimited Spreadsheet.vi"("file path (dialog if empty)"=w1768, "2D data"=w1772, "append to file? (new file:F)"=FALSE ("append to file? (F)"), "error in (no error)"=w1767, "transpose? (no:F)"=FALSE ("transpose? (F)"), "delimiter (\\t)"="," ("delimiter (\\t)")) -> ("error out"=w1766:errorcluster)  [unwired: 8 in, 1 out]
                  }
                  frame True {
                    # "To append"
                    n1367 = call-poly <vilib>:"Write Delimited Spreadsheet.vi"("file path (dialog if empty)"=w1786, "1D data"=w1787, "append to file? (new file:F)"=TRUE ("append to file? (F)"), "error in (no error)"=w1785, "transpose? (no:F)"=FALSE ("transpose? (F)"), "delimiter (\\t)"="," ("delimiter (\\t)")) -> ("error out"=w1784:errorcluster)  [unwired: 8 in, 1 out]
                  }
                }
                n1368 = local write "error"(w1743) -> ()
              }
              frame #2 {
                n1369 = disable-structure shown="Disabled" {
                  frame Disabled {
                    # "Temporarily disabled"
                    # "7-7-17 Added frame to Save parameter\nreview file"
                    # "Review file name"
                    n1370 = local read "Display UUT #"() -> (w1801:i32)
                    n1371 = local read "Display UUT #"() -> (w1806:i32)
                    n1372 = local read "Comments"() -> (w1807:string[])
                    n1373 = local read "Data Time"() -> (w1792:timestamp)
                    n1374 = local read "Serial"() -> (w1800:string[])
                    n1375 = Index Array(array=w1800, index=w1801) -> (element=w1824:string)
                    n1376 = To Double Precision Float(number=w1792) -> (double precision float=w1791:dbl)
                    n1377 = Index Array(array=w1807, index=w1806) -> (element=w1808:string)
                    n1378 = local read "Lambda, nm"() -> (w1811:i32[])
                    n1379 = Concatenate Strings("RVW_" ("string"), w1824, "_" ("string"), w1808, ".CSV" ("string")) -> (w1817:string)
                    n1380 = local read "780nm Folder"() -> (w1814:path)
                    n1381 = local read "850nm Folder"() -> (w1815:path)
                    n1382 = To Time Stamp(1:w1791) -> (0:w1797:timestamp)
                    n1383 = local read "Project Folder"() -> (w1816:path)
                    n1384 = local read "635nm Folder"() -> (w1813:path)
                    n1385 = local read "Display UUT #"() -> (w1810:i32)
                    n1386 = Number To Decimal String(number=w1811) -> (decimal integer string=w1812:string[])  [unwired: 1 in]
                    n1387 = Format Date/Time String(time format string (%c)="%m/%d/%y", seconds (now)=w1797) -> (date/time string=w1796:string)  [unwired: 1 in]
                    n1388 = Format Date/Time String(time format string (%c)="%H:%M:%S", seconds (now)=w1797) -> (date/time string=w1795:string)  [unwired: 1 in]
                    n1389 = Number To Exponential String(number=w1791, precision (6)=i16 12) -> (E-format string=w1794:string)  [unwired: 2 in]
                    n1390 = local read "error"() -> (w1818:errorcluster)
                    n1391 = Index Array(array=w1812, index=w1810) -> (element=w1825:string)
                    n1392 = local read "Display UUT #"() -> (w1829:i32)
                    n1393 = local read "MCUCheck"() -> (w1830:string[][])
                    n1394 = local read "SysCheck"() -> (w1831:string[][])
                    n1395 = call "SelectFileFolder(SubVI).vi"("635nmSubFolder"=w1813, "Project Folder in"=w1816, "Wavelength String"=w1825, "780nmSubFolder"=w1814, "850nmSubFolder"=w1815, "name or relative path"=w1817, "error in"=w1818) -> ("appended path"=w1821:path, "error out"=w1819:errorcluster)  [unwired: 7 in]
                    n1396 = local read "New File"() -> (w1803:bool)
                    n1397 = call <vilib>:"Check if File or Folder Exists.vi"("error in (no error)"=w1819, "path"=w1821) -> ("error out"=w1823:errorcluster, "file or folder exists?"=w1804:bool, "dup path"=w1827:path)  [unwired: 7 in]
                    n1398 = Index Array(array=w1830, index (col)=w1829) -> (element=w1832:string[])  [unwired: 1 in]
                    n1399 = Index Array(array=w1831, index (col)=w1829) -> (element=w1833:string[])  [unwired: 1 in]
                    n1400 = Not(x=w1803) -> (.not. x?=w1805:bool)
                    n1401 = And(x=w1804, y=w1805) -> (x .and. y?=w1820:bool)
                    n1402 = Build Array (concatenate)(w1796, w1795, w1794, w1832, w1833) -> (w1822:string[])
                    n1403 = case shown="False" w1820 {
                      tunnel: w1827 -> [w1837 w1856]
                      tunnel: w1822 -> [w1838 w1853]
                      tunnel: w1823 -> [w1836 w1855]
                      tunnel: w1824 -> [w1839 _]
                      tunnel: w1825 -> [w1840 _]
                      tunnel: [w1835 w1854] -> w1826
                      frame False {
                        # "To write"
                        n1404 = local read "FW Prm"() -> (w1848:string[])
                        n1405 = local read "Sys Prm"() -> (w1845:string[])
                        n1406 = Build Array("Color " ("time format string (%c)"), w1840) -> (w1849:string[])
                        n1407 = Build Array (concatenate)(string[] ["Date", "Time", "Time Stamp"] ("element"), w1848, w1845) -> (w1846:string[])
                        n1408 = Build Array("Serial Number " ("time format string (%c)"), w1839, "R=Out of Range" ("element")) -> (w1850:string[])
                        n1409 = Build Array(w1850, w1849, w1846, w1838) -> (w1841:string[][])
                        n1410 = call-poly <vilib>:"Write Delimited Spreadsheet.vi"("file path (dialog if empty)"=w1837, "2D data"=w1841, "append to file? (new file:F)"=FALSE ("append to file? (F)"), "error in (no error)"=w1836, "transpose? (no:F)"=FALSE ("transpose? (F)"), "delimiter (\\t)"="," ("delimiter (\\t)")) -> ("error out"=w1835:errorcluster)  [unwired: 8 in, 1 out]
                      }
                      frame True {
                        # "To append"
                        n1411 = call-poly <vilib>:"Write Delimited Spreadsheet.vi"("file path (dialog if empty)"=w1856, "1D data"=w1853, "append to file? (new file:F)"=TRUE ("append to file? (F)"), "error in (no error)"=w1855, "transpose? (no:F)"=FALSE ("transpose? (F)"), "delimiter (\\t)"="," ("delimiter (\\t)")) -> ("error out"=w1854:errorcluster)  [unwired: 8 in, 1 out]
                      }
                    }
                    n1412 = local write "error"(w1826) -> ()
                  }
                  frame Enabled {
                  }
                }
              }
              frame #3 {
                n1413 = local read "SysFileDelete"() -> (w1862:i32)
                n1414 = Decrement(x=w1862) -> (x-1=w1861:i32)
                n1415 = local write "Msg"("Idle" ("Msg")) -> ()
                n1416 = local write "Save"(FALSE ("Update")) -> ()
                n1417 = Greater Than 0?(x=w1861) -> (x > 0?=w1860:bool)
                n1418 = local write "SysFileDelete"(w1861) -> ()
                n1419 = local write "New File"(w1860) -> ()
              }
            }
          }
        }
      }
      frame #19 {
        # "Read from file"
        n1420 = case shown="True" "Read" {
          frame False {
          }
          frame True {
            n1421 = stacked-sequence {
              frame #0 {
                n1422 = local write "Points"(i32[] [] ("Points")) -> ()
                n1423 = local write "All Results"(dbl[][][] [] ("All Results")) -> ()
                n1424 = local write "Msg"("Reading data" ("Msg")) -> ()
              }
              frame #1 {
                n1425 = local read "DUT Count"() -> (w1869:i32)
                n1426 = for {
                  N: w1869 -> [_]
                  i -> [w1870]
                  # "6-21-17 Modified"
                  n1427 = call-poly <vilib>:"Read Delimited Spreadsheet.vi"("format (%.3f)"="%.12e", "delimiter (\\t)"="," ("delimiter (\\t)")) -> ("new file path (Not A Path if cancelled)"=w1874:path, "all rows"=w1873:dbl[][])  [unwired: 8 in, 4 out]
                  n1428 = call <vilib>:"Check if File or Folder Exists.vi"("path"=w1874) -> ("file or folder exists?"=w1872:bool, "dup path"=w1871:path)  [unwired: 8 in, 1 out]
                  n1429 = case shown="True" w1872 {
                    tunnel: w1873 -> [_ w1885]
                    tunnel: w1871 -> [_ w1884]
                    tunnel: w1870 -> [_ w1883]
                    frame False {
                      n1430 = local read "All Results"() -> (w1880:dbl[][][])
                      n1431 = local read "Points"() -> (w1882:i32[])
                      n1432 = Build Array (concatenate)(w1882, 0 ("millisecond multiple")) -> (w1881:i32[])
                      n1433 = Build Array (concatenate)(w1880, dbl[][] [] ("array")) -> (w1879:dbl[][][])
                      n1434 = local write "All Results"(w1879) -> ()
                      n1435 = local write "Points"(w1881) -> ()
                    }
                    frame True {
                      n1436 = stacked-sequence {
                        tunnel: w1885 -> [w1886 _]
                        tunnel: w1884 -> [_ w1901]
                        tunnel: w1883 -> [_ w1900]
                        frame #0 {
                          n1437 = Delete From Array(array=w1886, length=4, index (row)=0) -> (array with subset deleted=w1888:dbl[][])  [unwired: 1 in, 1 out]
                          n1438 = local read "All Results"() -> (w1892:dbl[][][])
                          n1439 = Delete From Array(array=w1888, length=2, index (col)=0 ("index (row)")) -> (array with subset deleted=w1887:dbl[][])  [unwired: 1 in, 1 out]
                          n1440 = Array Size(array=w1887) -> (size(s)=w1897:i32[])
                          n1441 = Build Array (concatenate)(w1892, w1887) -> (w1891:dbl[][][])
                          n1442 = Index Array(array=w1897, index=0) -> (element=w1894:i32)
                          n1443 = local write "All Results"(w1891) -> ()
                          n1444 = local read "Points"() -> (w1895:i32[])
                          n1445 = Build Array (concatenate)(w1895, w1894) -> (w1893:i32[])
                          n1446 = local write "Points"(w1893) -> ()
                        }
                        frame #1 {
                          w1907 = "                " ("String")
                          n1447 = Strip Path(path=w1901) -> (name=w1909:string)  [unwired: 1 out]
                          n1448 = Match Pattern(string=w1909, regular expression=".CSV") -> (before substring=w1911:string)  [unwired: 1 in, 3 out]
                          n1449 = String Subset(string=w1911, length (rest)=16 ("length (rest)")) -> (substring=w1903:string)  [unwired: 1 in]
                          n1450 = String Length(string=w1903) -> (length=w1906:i32)
                          n1451 = String Length(string=w1907) -> (length=w1908:i32)
                          n1452 = Subtract(x=w1908, y=w1906) -> (x-y=w1905:i32)
                          n1453 = Replace Substring(2:w1906, 3:w1905, 4:w1903, 5:w1907) -> (1:w1902:string)  [unwired: 1 out]
                          n1454 = property on="Time" class="XYGraph (strict)"("Active Plot"=w1900, "Plot.Plot Name"=w1902) -> ()  [unwired: 2 in, 2 out]
                        }
                      }
                    }
                  }
                }
              }
              frame #2 {
                n1455 = local write "Update Graph"(TRUE ("Update")) -> ()
                n1456 = local write "Msg"("Idle" ("Msg")) -> ()
              }
            }
          }
        }
      }
      frame #20 {
        n1457 = local read "Parameter Displayed"() -> (w1916:u16)
        n1458 = local read "Display Parameter"() -> (w1915:u16)
        n1459 = Not Equal?(x=w1915, y=w1916) -> (x != y?=w1914:bool)
        n1460 = case shown="True" w1914 {
          frame False {
          }
          frame True {
            n1461 = local read "Display Parameter"() -> (w1917:u16)
            n1462 = local write "Update Graph"(TRUE ("Update")) -> ()
            n1463 = local write "Parameter Displayed"(w1917) -> ()
          }
        }
      }
      frame #21 {
        n1464 = property on="Time" class="XYGraph (strict)"() -> ("XScale.Range"=w1923:T4)  [unwired: 2 in, 2 out]
        n1465 = property on="Time 2" class="XYGraph (strict)"() -> ("XScale.Range"=w1922:T4)  [unwired: 2 in, 2 out]
        n1466 = Cluster To Array(cluster=w1923) -> (array=w1920:dbl[])
        n1467 = Cluster To Array(cluster=w1922) -> (array=w1919:dbl[])
        n1468 = Not Equal?(x=w1920, y=w1919) -> (x != y?=w1921:bool)
        n1469 = case shown="True" w1921 {
          frame False {
          }
          frame True {
            n1470 = property on="Time 2" class="XYGraph (strict)"() -> ("Plot Bounds"=w1931:T5)  [unwired: 2 in, 2 out]
            n1471 = property on="Time" class="XYGraph (strict)"() -> (error out=w1925:errorcluster, "Width"=w1933:u32, "XScale.Range"=w1934:T4, "Plot Bounds"=w1932:T5)  [unwired: 2 in, 1 out]
            n1472 = Unbundle By Name(w1932) -> ("Left"=w1928:i16, "Right"=w1927:i16)  [unwired: 2 out]
            n1473 = Unbundle By Name(w1931) -> ("Top"=w1929:i16, "Bottom"=w1930:i16)  [unwired: 2 out]
            n1474 = local write "Update Graph"(TRUE ("Update")) -> ()
            n1475 = Bundle By Name(cluster=w1931, "Left"=w1928, "Top"=w1929, "Right"=w1927, "Bottom"=w1930) -> (w1926:T5)
            n1476 = property on="Time 2" class="XYGraph (strict)"(error in=w1925, "Width"=w1933, "XScale.Range"=w1934, "Plot Bounds"=w1926) -> ()  [unwired: 1 in, 2 out]
          }
        }
      }
      frame #22 {
        # "Highlight Trace of Multi-Plot Graph for DUT with New Data"
        n1477 = local read "Display UUT #"() -> (w1939:i32)
        n1478 = local read "Display UUT # Old"() -> (w1940:i32)
        n1479 = Not Equal?(x=w1939, y=w1940) -> (x != y?=w1935:bool)
        n1480 = Equal To 0?(x=w1938) -> (x = 0?=w1937:bool)
        n1481 = Compound Arithmetic op=OR(w1935, w1937) -> (w1936:bool)
        n1482 = case shown="True" w1936 {
          tunnel: w1935 -> [_ w1941]
          frame False {
          }
          frame True {
            n1483 = flat-sequence {
              frame #0 {
                n1484 = local read "Display UUT # Old"() -> (w1943:i32)
                n1485 = property on="Time" class="XYGraph (strict)"("Active Plot"=w1943, "Plot.Line Width"=u8 0) -> ()  [unwired: 2 in, 2 out]
              }
              frame #1 {
                n1486 = local read "Display UUT #"() -> (w1944:i32)
                n1487 = local write "Display UUT # Old"(w1944) -> ()
                n1488 = property on="Time" class="XYGraph (strict)"("Active Plot"=w1944, "Cursor.Cursor Plot"=w1944, "Plot.Line Width"=u8 3) -> ()  [unwired: 2 in, 2 out]
              }
              frame #2 {
                n1489 = property on="Time" class="XYGraph (strict)"() -> ("Plot.Plot Color"=w1947:u32, "Plot.Plot Name"=w1946:string)  [unwired: 2 in, 2 out]
                n1490 = property on="Time" class="XYGraph (strict)"("Cursor.Cursor Color"=w1947, "Cursor.Cursor Name"=w1946) -> ()  [unwired: 2 in, 2 out]
              }
            }
            n1491 = local write "Update Graph"(w1941) -> ()
          }
        }
      }
      frame #23 {
        n1492 = property on="Time" class="XYGraph (strict)"() -> ("Cursor.Cursor X"=w1953:dbl)  [unwired: 2 in, 2 out]
        n1493 = local read "Old Cursor"() -> (w1952:dbl)
        n1494 = local read "Busy"() -> (w1951:bool)
        n1495 = Not Equal?(x=w1953, y=w1952) -> (x != y?=w1949:bool)
        n1496 = Not(x=w1951) -> (.not. x?=w1950:bool)
        n1497 = And(x=w1949, y=w1950) -> (x .and. y?=w1948:bool)
        n1498 = case shown="True" w1948 {
          frame False {
          }
          frame True {
            n1499 = local read "Display UUT #"() -> (w1963:i32)
            n1500 = local read "Points"() -> (w1961:i32[])
            n1501 = local read "All Results"() -> (w1962:dbl[][][])
            n1502 = Index Array(array=w1961, index=w1963) -> (element=w1959:i32)
            n1503 = property on="Time" class="XYGraph (strict)"() -> ("Cursor.Cursor X"=w1968:dbl)  [unwired: 2 in, 2 out]
            n1504 = Index Array(array=w1962, index (dim 0)=w1963, index (dim 2)=0 ("disabled index (col)")) -> (element=w1956:dbl[])  [unwired: 1 in]
            n1505 = Array Subset(array=w1956, length=w1959) -> (w1960:dbl[])  [unwired: 1 in]
            n1506 = To Time Stamp(1:w1960) -> (0:w1958:timestamp[])
            n1507 = To Time Stamp(1:w1968) -> (0:w1969:timestamp)
            n1508 = Subtract(x=w1958, y=w1969) -> (x-y=w1970:dbl[])
            n1509 = Absolute Value(x=w1970) -> (abs(x)=w1965:dbl[])
            n1510 = Array Max & Min(array=w1965) -> (min index (indices)=w1967:i32)  [unwired: 3 out]
            n1511 = property on="Time" class="XYGraph (strict)"() -> ("Cursor.Cursor X"=→"Curs":dbl, "Cursor.Cursor Y"=→"Pos":dbl)  [unwired: 2 in, 2 out]
            n1512 = Index Array(array=w1958, index=w1967) -> (element=w1964:timestamp)
            n1513 = To Double Precision Float(number=w1964) -> (double precision float=w1966:dbl)
            n1514 = local write "Old Cursor"(w1966) -> ()
            n1515 = property on="Time" class="XYGraph (strict)"("Cursor.Cursor X"=w1966) -> ()  [unwired: 2 in, 2 out]
          }
        }
      }
      frame #24 {
        # "Update graphs and power calculations."
        n1516 = local read "Update Graph"() -> (w1971:bool)
        n1517 = case shown="True" w1971 {
          frame False {
          }
          frame True {
            n1518 = stacked-sequence {
              frame #0 {
                w1972 = T2 [] ("Time")
                n1519 = local write "Time 2"(w1972) -> ()
                n1520 = local write "Time"(w1972) -> ()
              }
              frame #1 {
                n1521 = local read "DUT Count"() -> (w1973:i32)
                n1522 = for {
                  N: w1973 -> [_]
                  i -> [w1980]
                  n1523 = local read "Display Parameter"() -> (w1975:u16)
                  n1524 = local read "All Results"() -> (w1986:dbl[][][])
                  n1525 = local read "Points"() -> (w1981:i32[])
                  n1526 = Index Array(array=w1981, index=w1980) -> (element=w1977:i32)
                  n1527 = Index Array(array=w1986, index (dim 0)=w1980) -> (element=w1985:dbl[][])  [unwired: 2 in]
                  n1528 = Delete From Array(array=w1985, index (col)=0 ("disabled index (col)")) -> (deleted portion=w1979:dbl[], array with subset deleted=w1987:dbl[][])  [unwired: 2 in]
                  n1529 = Index Array(array=w1987, index (col)=w1975) -> (element=w1976:dbl[])  [unwired: 1 in]
                  n1530 = Array Subset(array=w1979, length=w1977) -> (w1978:dbl[])  [unwired: 1 in]
                  n1531 = To Time Stamp(1:w1978) -> (0:w1984:timestamp[])
                  n1532 = Array Subset(array=w1976, length=w1977) -> (w1974:dbl[])  [unwired: 1 in]
                  n1533 = local read "Time"() -> (w1983:T2)
                  n1534 = Bundle(w1984, w1974) -> (w1989:cluster{timestamp[], dbl[]})  [unwired: 1 in]
                  n1535 = Build Array (concatenate)(w1983, w1989) -> (w1988:T2)
                  n1536 = local write "Time"(w1988) -> ()
                }
              }
              frame #2 {
                # "2-12-20:\nChanged from\n14 DAQ system parameters to 11\nto eliminate non-functional temp\nreadings"
                n1537 = local read "Display UUT #"() -> (w2009:i32)
                n1538 = local read "All Results"() -> (w1998:dbl[][][])
                n1539 = local read "Points"() -> (w2003:i32[])
                n1540 = local read "FW Prm"() -> (w1995:string[])
                n1541 = local read "Sys Prm"() -> (w1993:string[])
                n1542 = local read "Meas N"() -> (w1992:i32)
                n1543 = Index Array(array=w1998, index (dim 0)=w2009) -> (element=w1999:dbl[][])  [unwired: 2 in]
                n1544 = Index Array(array=w2003, index=w2009) -> (element=w2006:i32)
                n1545 = Build Array (concatenate)(w1995, w1993) -> (w1994:string[])
                n1546 = Subtract(x=w1992, y=11) -> (x-y=w1990:i32)
                n1547 = Delete From Array(array=w1999, index (col)=0 ("disabled index (col)")) -> (deleted portion=w2004:dbl[], array with subset deleted=w1997:dbl[][])  [unwired: 2 in]
                n1548 = local read "Display Parameter"() -> (w2010:u16)
                n1549 = Index Array(array=w1997, index (col)=w1990) -> (element=w2007:dbl[])  [unwired: 1 in]
                n1550 = Array Subset(array=w2004, length=w2006) -> (w2005:dbl[])  [unwired: 1 in]
                n1551 = To Time Stamp(1:w2005) -> (0:w2000:timestamp[])
                n1552 = Array Subset(array=w2007, length=w2006) -> (w2008:dbl[])  [unwired: 1 in]
                n1553 = Index Array(array=w1994, index=w2010) -> (element=w2011:string)
                n1554 = property on="Time" class="XYGraph (strict)"("YScale.NameLbl.Text"=w2011) -> ()  [unwired: 2 in, 2 out]
                n1555 = local read "Time 2"() -> (w2001:T2)
                n1556 = Bundle(w2000, w2008) -> (w1996:cluster{timestamp[], dbl[]})  [unwired: 1 in]
                n1557 = Build Array (concatenate)(w2001, w1996) -> (w2012:T2)
                n1558 = local write "Time 2"(w2012) -> ()
              }
              frame #3 {
                n1559 = local write "Max Power"(-1000.0 ("Max Power")) -> ()
                n1560 = local write "Min Power"(1000.0 ("Max Power")) -> ()
                n1561 = local write "Start Power"(-1000.0 ("Max Power")) -> ()
              }
              frame #4 {
                # "Constant was 14."
                n1562 = local read "Display UUT #"() -> (w2032:i32)
                n1563 = local read "All Results"() -> (w2033:dbl[][][])
                n1564 = local read "Points"() -> (w2037:i32[])
                n1565 = local read "Meas N"() -> (w2018:i32)
                n1566 = local read "Warm-up, min"() -> (w2029:dbl)
                n1567 = local read "Stability Time, min"() -> (w2020:dbl)
                n1568 = Index Array(array=w2037, index=w2032) -> (element=w2031:i32)
                n1569 = Subtract(x=w2018, y=11 ("Offset Constant")) -> (x-y=w2016:i32)
                n1570 = Multiply(x=w2029, y=60.0) -> (x*y=w2027:dbl)
                n1571 = Multiply(x=w2020, y=60.0) -> (x*y=w2019:dbl)
                n1572 = Index Array(array=w2033, index (dim 0)=w2032, index (dim 2)=w2016) -> (element=w2034:dbl[])  [unwired: 1 in]
                n1573 = Index Array(array=w2033, index (dim 0)=w2032, index (dim 2)=0 ("disabled index (col)")) -> (element=w2035:dbl[])  [unwired: 1 in]
                n1574 = Array Subset(array=w2034, length=w2031) -> (w2030:dbl[])  [unwired: 1 in]
                n1575 = Array Subset(array=w2035, length=w2031) -> (w2024:dbl[])  [unwired: 1 in]
                n1576 = Index Array(array=w2024, index=0) -> (element=w2022:dbl)
                n1577 = Add(x=w2022, y=w2027) -> (x+y=w2026:dbl)
                n1578 = local write "First Point"(w2022) -> ()
                n1579 = Add(x=w2026, y=w2019) -> (x+y=w2025:dbl)
                n1580 = for {
                  N: w2031 -> [_]
                  tunnel: w2024 -> [w2043] mode=indexing
                  tunnel: w2030 -> [w2038] mode=indexing
                  tunnel: w2026 -> [w2044]
                  tunnel: w2025 -> [w2042]
                  # "Note:  Above comparsion will always fail the greater than limit check on 1st pass as the 2\nvalues are always equal and the loop will redundantly read all other previous data."
                  n1581 = Greater?(x=w2043, y=w2044) -> (0:w2041:bool)
                  n1582 = Less?(x=w2043, y=w2042) -> (x < y?=w2040:bool)
                  n1583 = And(x=w2041, y=w2040) -> (x .and. y?=w2039:bool)
                  n1584 = case shown="False" w2039 {
                    tunnel: w2038 -> [_ w2048]
                    frame False {
                    }
                    frame True {
                      n1585 = local read "Start Power"() -> (w2047:dbl)
                      n1586 = local read "Max Power"() -> (w2052:dbl)
                      n1587 = local read "Min Power"() -> (w2050:dbl)
                      n1588 = Less?(x=w2047, y=-999.0) -> (x < y?=w2045:bool)
                      n1589 = Max & Min(x=w2052, y=w2048) -> (max(x,y)=w2051:dbl)  [unwired: 1 out]
                      n1590 = Max & Min(x=w2050, y=w2048) -> (min(x,y)=w2049:dbl)  [unwired: 1 out]
                      n1591 = case shown="False" w2045 {
                        tunnel: w2048 -> [_ w2053]
                        frame False {
                        }
                        frame True {
                          n1592 = local write "Start Power"(w2053) -> ()
                        }
                      }
                      n1593 = local write "Max Power"(w2051) -> ()
                      n1594 = local write "Min Power"(w2049) -> ()
                    }
                  }
                }
              }
              frame #5 {
                n1595 = local read "Max Power"() -> (w2063:dbl)
                n1596 = local read "Min Power"() -> (w2062:dbl)
                n1597 = local read "Start Power"() -> (w2056:dbl)
                n1598 = Subtract(x=w2063, y=w2062) -> (x-y=w2061:dbl)
                n1599 = Divide(x=w2061, y=w2056) -> (x/y=w2060:dbl)
                n1600 = Multiply(x=100.0, y=w2060) -> (x*y=w2055:dbl)
                n1601 = Absolute Value(x=w2055) -> (abs(x)=w2054:dbl)
                n1602 = Less Or Equal?(x=w2054, y=2.0) -> (x <= y?=→"Results":bool)
                n1603 = local write "Max Deviation"(w2054) -> ()
              }
              frame #6 {
                n1604 = local write "Update Graph"(FALSE ("Update")) -> ()
              }
            }
          }
        }
      }
      frame #25 {
        # "5-26-17 added"
        n1605 = case shown="True" "Save Data" {
          frame False {
          }
          frame True {
            w2096 = FALSE ("transpose? (F)")
            # "Select\nwhich\nunit"
            # "Exclude time stamp by\ndeleting the \nentire 0th column"
            # "Extract time stamp column\nat 0th column"
            n1606 = local read "All Results"() -> (w2074:dbl[][][])
            n1607 = local read "Select Unit"() -> (w2070:i32)
            n1608 = Delete From Array(array=w2074, length=1 ("disabled index (col)"), index (dim 2)=0 ("disabled index (col)")) -> (array with subset deleted=w2071:dbl[][][])  [unwired: 2 in, 1 out]
            n1609 = Index Array(array=w2074, index (dim 0)=w2070, index (dim 2)=0 ("disabled index (col)")) -> (element=w2077:dbl[])  [unwired: 1 in]
            n1610 = Index Array(array=w2071, index (dim 0)=w2070) -> (element=w2069:dbl[][])  [unwired: 2 in]
            n1611 = Array Size(array=w2077) -> (size(s)=w2073:i32)
            n1612 = local read "Lambda, nm"() -> (w2089:i32[])
            n1613 = local read "Select Unit"() -> (w2094:i32)
            n1614 = local read "Serial"() -> (w2090:string[])
            n1615 = local read "Select Unit"() -> (w2093:i32)
            n1616 = Number To Exponential String(number=w2069, precision (6)=i16 6) -> (E-format string=w2068:string[][])  [unwired: 2 in]
            n1617 = for {
              N: w2073 -> [_]
              tunnel: w2077 -> [w2100] mode=indexing
              tunnel: [w2099] -> w2067 mode=indexing
              tunnel: w2068 -> [w2098] mode=indexing
              n1618 = To Time Stamp(1:w2100) -> (0:w2101:timestamp)
              n1619 = Format Date/Time String(time format string (%c)="%m/%d/%y", seconds (now)=w2101) -> (date/time string=w2106:string)  [unwired: 1 in]
              n1620 = Format Date/Time String(time format string (%c)="%H:%M:%S", seconds (now)=w2101) -> (date/time string=w2107:string)  [unwired: 1 in]
              n1621 = Number To Exponential String(number=w2100, precision (6)=i16 12) -> (E-format string=w2105:string)  [unwired: 2 in]
              n1622 = Build Array (concatenate)(w2106, w2107, w2105, w2098) -> (w2099:string[])
            }
            n1623 = Index Array(array=w2090, index=w2094) -> (element=w2092:string)
            n1624 = Number To Decimal String(number=w2089) -> (decimal integer string=w2088:string[])  [unwired: 1 in]
            n1625 = Index Array(array=w2088, index=w2093) -> (element=w2091:string)
            n1626 = local read "FW Prm"() -> (w2083:string[])
            n1627 = local read "Sys Prm"() -> (w2081:string[])
            n1628 = Build Array("Serial Number " ("time format string (%c)"), w2092) -> (w2085:string[])
            n1629 = Build Array("Color " ("time format string (%c)"), w2091) -> (w2084:string[])
            n1630 = Build Array (concatenate)(string[] ["Date", "Time", "Time Stamp"] ("element"), w2083, w2081) -> (w2082:string[])
            n1631 = local read "error"() -> (w2079:errorcluster)
            n1632 = Build Array (concatenate)(w2085, w2084, w2082, w2067) -> (w2080:string[][])
            n1633 = call-poly <vilib>:"Write Delimited Spreadsheet.vi"("2D data"=w2080, "append to file? (new file:F)"=w2096, "error in (no error)"=w2079, "transpose? (no:F)"=w2096, "delimiter (\\t)"="," ("delimiter (\\t)")) -> ("error out"=w2066:errorcluster)  [unwired: 9 in, 1 out]
            n1634 = call <vilib>:"Simple Error Handler.vi"("error in (no error)"=w2066) -> ()  [unwired: 4 in, 5 out]
          }
        }
      }
      frame #26 {
        n1635 = Wait Until Next ms Multiple(millisecond multiple=u32 100) -> ()  [unwired: 1 out]
      }
      frame #27 {
        # "5-11-17 Revised, added close power meter USB device sequence\n5-15-17 Revised, added command to turn off power supplies"
        n1636 = Or(x="Close Ports", y="Stop") -> (x .or. y?=w2111:bool)
        n1637 = case shown="True" w2111 {
          frame False {
          }
          frame True {
            n1638 = stacked-sequence {
              frame #0 {
                n1639 = local write "Msg"("Turning off Power Supplies..." ("Msg")) -> ()
              }
              frame #1 {
                # "PSs off"
                n1640 = local read "Supply-PM Count"() -> (w2113:i32)
                n1641 = local read "error"() -> (w2114:errorcluster)
                n1642 = for {
                  N: w2113 -> [_]
                  shift-right: [w2119] -> w2115
                  shift-left: w2114 -> [w2120]
                  i -> [w2118]
                  n1643 = local read "DUT Count"() -> (w2116:i32)
                  n1644 = local read "COMs"() -> (w2121:refnum<visa-resource-name>[])
                  n1645 = Add(x=w2116, y=w2118) -> (x+y=w2117:i32)
                  n1646 = Index Array(array=w2121, index=w2117) -> (element=w2123:refnum<visa-resource-name>)
                  n1647 = call "PS_ManCMD.vi"("Power Sup: T-On/F-Off"=FALSE, "error in"=w2120, "VISA resource name"=w2123) -> ("error out"=w2119:errorcluster)  [unwired: 2 in]
                }
                n1648 = local write "error"(w2115) -> ()
              }
              frame #2 {
                # "COMs"
                n1649 = local read "COMs"() -> (w2125:refnum<visa-resource-name>[])
                n1650 = Array Size(array=w2125) -> (size(s)=w2126:i32)
                n1651 = for {
                  N: w2126 -> [_]
                  tunnel: w2125 -> [w2129] mode=indexing
                  tunnel: [FALSE] -> w2124 mode=indexing
                  n1652 = local read "error"() -> (w2130:errorcluster)
                  n1653 = VISA Close(VISA resource name=w2129, error in (no error)=w2130) -> (error out=w2128:errorcluster)
                  n1654 = local write "error"(w2128) -> ()
                }
                n1655 = local write "Com Open"(w2124) -> ()
              }
              frame #3 {
                # "5-11-17, added close PM USBs"
                n1656 = local read "reference Out"() -> (w2133:refnum<k24>)
                n1657 = local read "error"() -> (w2132:errorcluster)
                n1658 = call "NewPort_PM_USB_CloseDevice(SubVI).vi"("error in"=w2132, "reference In"=w2133) -> ("error out"=w2131:errorcluster)  [unwired: 9 in]
                n1659 = local write "error"(w2131) -> ()
              }
            }
          }
        }
      }
      frame #28 {
        # "5-4-17, added"
        n1660 = local read "Stop"() -> (w2135:bool)
        n1661 = case shown="True" w2135 {
          tunnel: [FALSE TRUE] -> w2134
          frame False {
          }
          frame True {
            w2139 = FALSE ("Auto")
            # "PSs off"
            # "Deactivate Re-conf"
            # "Deactivate Ready"
            # "Disable Verify Lambda button"
            # "Enable N systems selection"
            # "If stop, reset Test Start button"
            n1662 = local write "New Test"(w2139) -> ()
            n1663 = local write "Start Test"(w2139) -> ()
            n1664 = local write "Re-conf Lambda"(w2139) -> ()
            n1665 = local write "Ready"(w2139) -> ()
            n1666 = property on="DUT Count" class="Ring (strict)"("DisabledEnum"=T3."Enabled" ("Disabled")) -> ()  [unwired: 2 in, 2 out]
            n1667 = property on="Verify WavL" class="Bool"("DisabledEnum"=T3."Enabled" ("Disabled")) -> ()  [unwired: 2 in, 2 out]
            n1668 = local write "Msg"("Test stopped." ("Msg")) -> ()
          }
        }
      }
    }
  }
